vi "COD主界面（列队使用）.vi"() -> (8 "多列列表框":i32(listbox))   [LabVIEW 2016, in "斯坦道CODMn.lvlib"]
uses:
  <vilib>/Analysis/6fits.llb/Curve Fitting Criteria.ctl
  <vilib>/Utility/miscctls.llb/LVPointTypeDef.ctl
  <vilib>/Utility/config.llb/Read Key (I32).vi
  <vilib>/Utility/config.llb/Read Key (Double).vi
  <vilib>/Utility/config.llb/Read Key (Boolean).vi
  <vilib>/Utility/config.llb/Write Key (Double).vi
  <vilib>/Utility/config.llb/Write Key (Boolean).vi
  <vilib>/Utility/config.llb/Write Key (I32).vi
  <vilib>/Waveform/WDTFileIO.llb/Read Waveform from File.vi
  <vilib>/ptbypt/NI_PtbyPt.lvlib
  <vilib>/Utility/config.llb/NI_LVConfig.lvlib
  <vilib>/Analysis/NI_AALPro.lvlib
panel:
  in  "MB通信方式选择":enum16{"串口", "TCP"}(ring)
  in  "采水泵排液时间/s:":i32
  in  "采水泵润洗时间/s:":i32
  in  "采水泵沉淀时间/s:":i32
  in  "采水泵进样时间/s:":i32
  in  "常规版/认证版":enum16{"常规版", "认证版", "浮台版"}(ring)
  in  "释放串口":bool
  in  "打开串口":bool
  in  "保存参数":dbl[](array[numeric])
  out "报警数字":i16
  out "CODMn工作状态":T1(ring)
  out "ORP-K":string
  out "ORP-B":string
  out "ORP-A":string
  out "x = y?":bool
  out "稀释倍数解释":string
  in  "CODMn跨度量程选择":enum32{"H", "L", "AUTO"}(ring)=enum."AUTO"
  in  "跨度液浓度":dbl
  in  "水样":dbl
  in  "蒸馏水":dbl
  in  "标液":dbl
  in  "质控样":dbl
  in  "加标回收":dbl
  in  "草酸钠":dbl
  in  "高锰酸钾":dbl
  in  "硫酸":dbl
  out "量程解释说明":string
  in  "高切低阈值:":dbl
  in  "低切高阈值:":dbl
  in  "自动切换量程:":enum16{"关闭", "自动切换测一次", "自动切换测两次"}(ring)
  in  "修正系数":dbl
  in  "标准液浓度":dbl
  in  "温度":dbl
  in  "恒温时间":dbl
  in  "基本量程":enum16{"L", "H"}(ring)
  in  "CODMn零点核查选择":enum16{"零点核查走纯水管", "零点核查走质控管"}(ring)
  in  "锁定按钮":bool
  in  "低量程稀释倍数:":i8=1
  out "切换量程连续测两次":bool
  in  "高量程稀释倍数:":i8=2
  in  "一键写入":bool
  in  "测量模式(公式)":u16(ring)=1 items=["水样测试"=1, "标样核查"=2, "零点核查"=3, "跨度核查"=4, "空白测试"=5, "平行样"=6, "加标回收"=7]
  out "基本量程(显示)":string
  out "测量模式(显示)":string
  in  "量程切换次数":u8
  out "数据时间":string
  out "断电排液标记":bool
  out "COM":string
  in  "启用5":bool
  in  "校准5":bool
  in  "泵滴定数5":dbl
  in  "浓度5":dbl
  in  "启用4":bool
  in  "校准4":bool
  in  "泵滴定数4":dbl
  in  "浓度4":dbl
  out "波形时间":timestamp
  in  "历史波形":bool
  out "滴定数-ORP值":u16[](array[numeric]) caption="数组"
  in  "关闭 3":bool
  in  "滴定曲线":bool
  out "ORP滴定曲线":u16[](graph)
  out "空白测试标记":bool
  out "跨度核查标记":bool
  out "启动选择 2":u16(ring) items=["水样测试", "标样核查", "零点核查", "跨度核查", "空白测试", "加标回收", "平行样", "校零", "校标"]
  in  "量程选择":enum16{"低量程", "高量程", "0-2量程"}(ring)
  in  "手动控制":bool
  in  "选用水样":enum16{"葡萄糖", "草酸钠"}(ring)
  in  "方程系数":cluster{"K":dbl, "b":dbl, "X^2":dbl} {"X^2" format="%#.6g"; "b" format="%#.6g"; "K" format="%#.6g"}
  out "多项式系数":dbl[](array[numeric])
  out "XY图":cluster{"X Values":dbl[], "Y Values":dbl[]}[](graph)
  in  "模型":enum32{"线性", "多项式"}(ring)
  out "启动时间":timestamp format="%<%Y/%m/%d %H:%M:%S>T"
  in  "关闭 2":bool
  out "r^2":dbl format="%.8g"
  out "拟合公式":string
  out "b":dbl format="%#.4g"
  out "K":dbl format="%#.4f"
  out "当前校准":i32
  in  "启用3":bool
  in  "启用2":bool
  in  "启用1":bool
  in  "校准3":bool
  in  "校准2":bool
  in  "校准1":bool
  in  "泵滴定数3":dbl
  in  "泵滴定数2":dbl
  in  "泵滴定数1":dbl
  in  "浓度3":dbl
  in  "浓度2":dbl
  in  "浓度1":dbl
  in  "写入":bool
  out "测量模式数字":i32
  out "零点核查标记":bool
  out "排液故障":bool
  out "进水样超量程":bool
  out "标样核查标记":bool
  out "平行样测量":bool
  out "加标回收测量":bool
  out "质控样测量":bool
  out "待机":bool
  out "校标错误":bool
  out "校零错误":bool
  out "测量错误":bool
  out "草酸钠报警":bool
  out "高锰酸钾报警":bool
  out "加热故障":bool
  out "温控器故障":bool
  out "ORP故障":bool
  out "排液标记":bool
  out "故障标记":bool
  out "校标标记":bool
  out "校零标记":bool
  out "通讯状态":bool
  out "水样测量":bool
  in  "读取":bool
  in  "返回":bool
  in  "校准配置":bool
  in  "零点泵计量数 2":dbl
  in  "标度泵计量数 2":dbl
  out "标度滴定值":dbl
  out "零点滴定值":dbl
  in  "保存":bool
  in  "关闭":bool
  out "测量数据区":T2 {"单位" items=["ug/L", "mg/L", "ppm", "mg/m3", "cm", "ppb", "ug/m3", "%", "nmol/mol", "umol/mol", "MPN/L", "MPN/100ml", "ng/m3", "NTU", "无量纲", "ms/cm", "us/cm", "℃", "mV", "万个/L"]}
  out "仪器时间":timestamp format="%<%Y/%m/%d %H:%M:%S>T"
  out "秒":u16
  out "分":u16
  out "COD浓度（mg/L)":dbl format="%.2g"
  out "进样管":dbl
  out "高锰酸钾":dbl
  out "草酸钠":dbl
  out "硫酸":dbl
  out "ORP显示":dbl
  out "温度":dbl
  out "加热":bool
  out "搅拌":bool
  out "进硫酸":bool
  out "进加标回收样":bool
  out "进质控样":bool
  out "进标液":bool
  out "进蒸馏水":bool
  out "进水样":bool
  out "进草酸钠":bool
  out "进高锰酸钾":bool
  out "定时启动":bool
  in  "启动":bool
  in  "故障清除":bool
  in  "参数配置":bool
  in  "停止":bool
  in  "单步启动":bool
  out "系统时间":timestamp
  in  "时间校准":bool
  out "报警簇":T3
  out "模式（受控）":u16
  # "测量时间："
  # "(水样~加标回收)"
  # "mV"
  # "℃"
  # "注：遇到加热故障和排液故障时仪器不能正常启动，\n必须排查故障并点击报警清除按钮方可运行。"
  # "mg/L"
  # "基本参数设置"
  # "校零校标结果"
  # "泵计量参数设置"
  # "校零结果："
  # "校零滴定值："
  # "加热恒温温度(℃):"
  # "水样："
  # "高锰酸钾："
  # "校标结果："
  # "标度滴定值："
  # "恒温时间(分钟):"
  # "草酸钠："
  # "蒸馏水："
  # "零点泵计量值："
  # "标准液浓度(mg/L):"
  # "硫酸："
  # "标液："
  # "标度泵计量值："
  # "修正系数："
  # "跨度液浓度："
  # "质控样:"
  # "基本量程(L、H)可选:"
  # "跨度量程选择："
  # "加标回收样："
  # "是否启用"
  # "泵滴定数"
  # "浓度"
  # "辅\n助\n计\n算\n区"
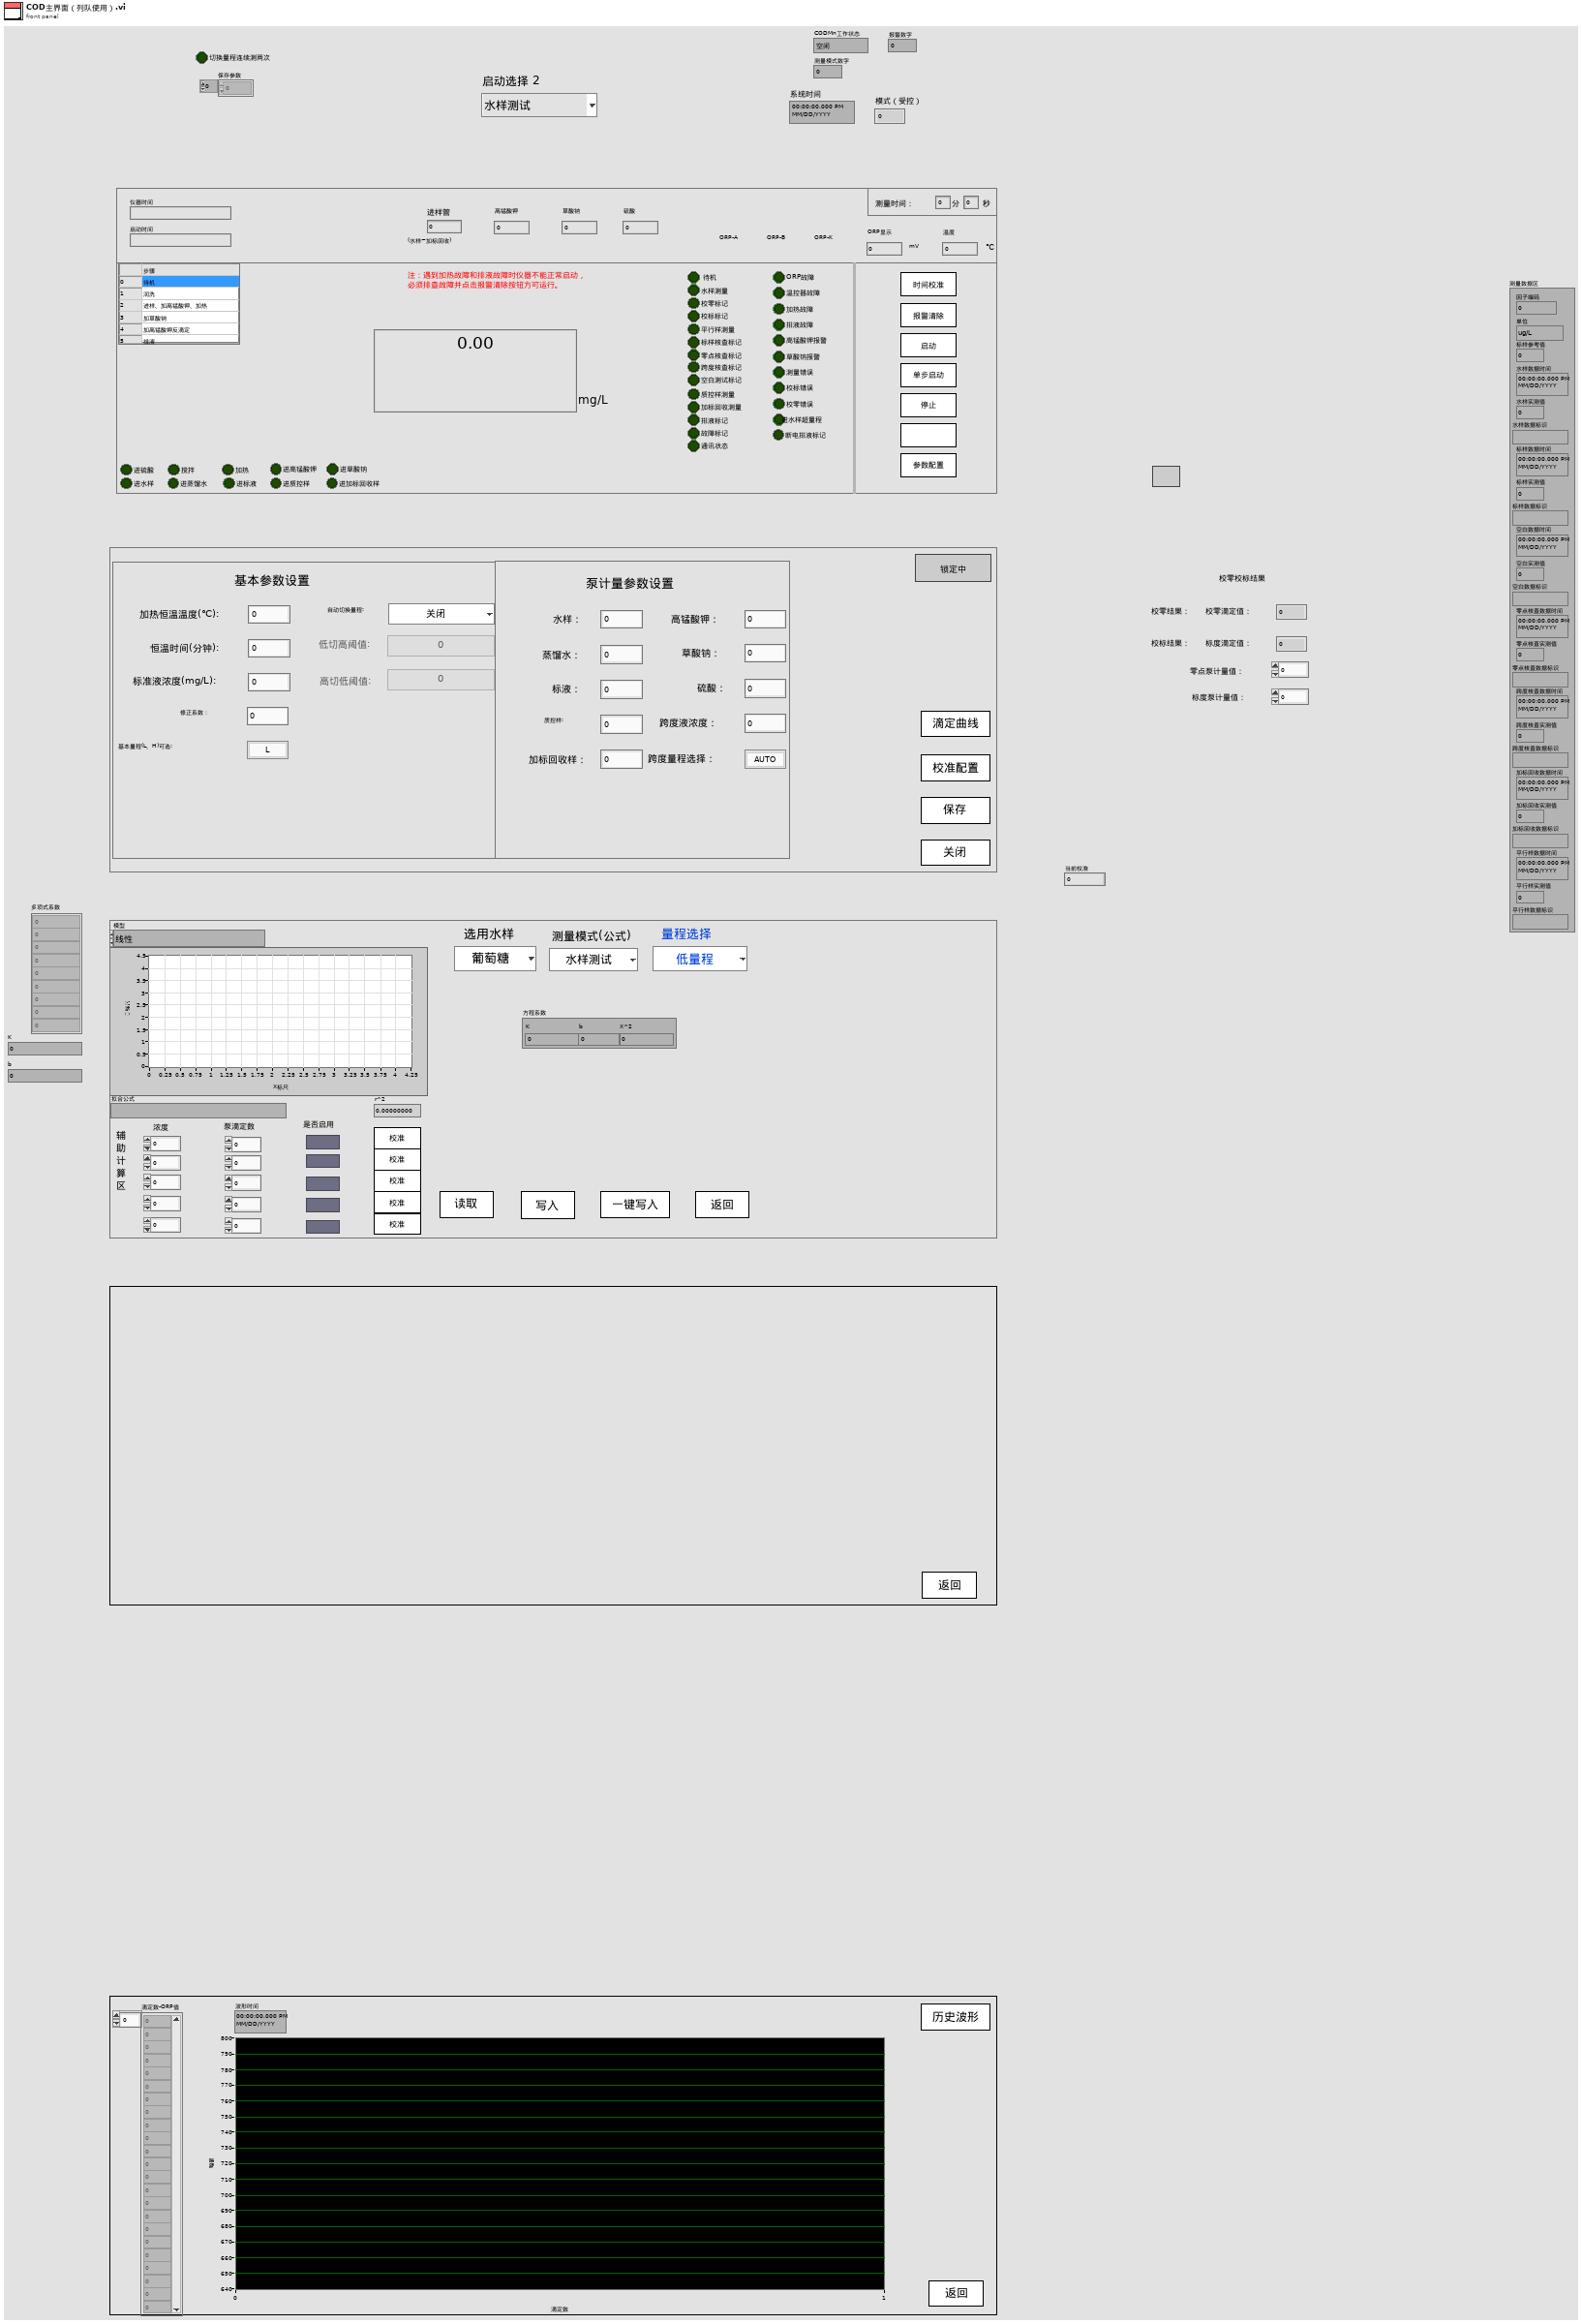
[diagram p1: front panel]
types:
  T1 = enum16{"空闲", "水样测试", "标样核查", "零点核查", "跨度核查", "空白测试", "平行样测试", "质控样", "空白校准", "标样校准", "加标回收"}
  T2 = cluster{"因子编码":u32, "单位":u16, "标样参考值":sgl, "水样数据时间":timestamp, "水样实测值":sgl, "水样数据标识":string, "标样数据时间":timestamp, "标样实测值":sgl, "标样数据标识":string, "空白数据时间":timestamp, "空白实测值":sgl, "空白数据标识":string, "零点核查数据时间":timestamp, "零点核查实测值":sgl, "零点核查数据标识":string, "跨度核查数据时间":timestamp, "跨度核查实测值":sgl, "跨度核查数据标识":string, "加标回收数据时间":timestamp, "加标回收实测值":sgl, "加标回收数据标识":string, "平行样数据时间":timestamp, "平行样实测值":sgl, "平行样数据标识":string}
  T3 = cluster{"ORP故障":bool, "温控器故障":bool, "加热故障":bool, "高锰酸钾报警":bool, "草酸钠报警":bool, "测量错误":bool, "校零错误":bool, "校标错误":bool, " 进水样超量程":bool, "排液阀故障":bool}
  T4 = cluster{"时间":timestamp, "测量模式":string, "数据类型":string, "检测值":sgl, "单位":string, "数据标识":string, "因子编码":string, "标样参考值":sgl, "ORP-A":sgl, "ORP-B":sgl, "ORP-K":sgl, "COD滴定值":sgl, "高锰酸钾滴定数":sgl, "温度":sgl, "量程":sgl}
  T5 = enum8{"Enabled", "Disabled", "Disabled and Grayed Out"}
  T6 = cluster{"数组 2[0]":sgl, "数组 2[1]":sgl, "数组 2[2]":sgl, "数组 2[3]":sgl, "数组 2[4]":sgl, "数组 2[5]":sgl, "数组 2[6]":sgl, "数组 2[7]":sgl, "数组 2[8]":sgl, "数组 2[9]":sgl, "数组 2[10]":sgl, "数组 2[11]":sgl, "数组 2[12]":sgl, "数组 2[13]":sgl, "数组 2[14]":sgl, "数组 2[15]":sgl, "数组 2[16]":sgl, "数组 2[17]":sgl, "数组 2[18]":sgl, "数组 2[19]":sgl, "数组 2[20]":sgl, "数组 2[21]":sgl, "数组 2[22]":sgl, "数组 2[23]":sgl, "数组 2[24]":sgl, "数组 2[25]":sgl, "数组 2[26]":sgl, "数组 2[27]":sgl, "数组 2[28]":sgl, "数组 2[29]":sgl, "数组 2[30]":sgl, "数组 2[31]":sgl, "数组 2[32]":sgl, "数组 2[33]":sgl, "数组 2[34]":sgl, "数组 2[35]":sgl, "数组 2[36]":sgl, "数组 2[37]":sgl, "数组 2[38]":sgl, "数组 2[39]":sgl, "数组 2[40]":sgl, "数组 2[41]":sgl}
  T7 = typedef "NI_AALPro.lvlib/Curve Fitting Criteria.ctl" = u16
  T8 = cluster{"测量模式":enum16{"水样测量", "标样核查", "零点核查", "跨度核查", "空白测试", "加标回收", "平行样", "校零", "校标"}}
  T9 = cluster{"仪器测试类型":enum16{"水样测试", "零点核查", "标样核查", "空白测试", "跨度核查", "加标回收", "平行样", "校零", "校标"}, "周期设置类型":enum16{"定点启动", "间隔启动"}, "定时功能启用":bool, "定时间隔":dbl, "24H周期设置":bool[]}
  T10 = typedef "LVDateTimeRec.ctl" = cluster{"秒数的小数部分":dbl, "秒":i32, "分":i32, "时":i32, "日":i32, "月":i32, "年":i32, "天数（周）":i32, "天数（年）":i32, "DST":i32}
  T11 = enum16{"水样测试", "零点核查", "标样核查", "空白测试", "跨度核查", "加标回收", "平行样", "校零", "校标"}
  T12 = cluster{"时间标识":timestamp, "设备":string, "日志信息":string}
  T13 = cluster{"时间标识":timestamp, "参数":string, "日志信息":string, "流程参数":string}
  T14 = cluster{"时间标识":timestamp, "设备":string, "日志信息":string, "流程参数":string}
  T15 = typedef "NI_LVConfig.lvlib/Config Data RefNum.ctl" = refnum<k1>
  T16 = typedef "LVPointTypeDef.ctl" = cluster{"Horizontal":i16, "Vertical":i16}
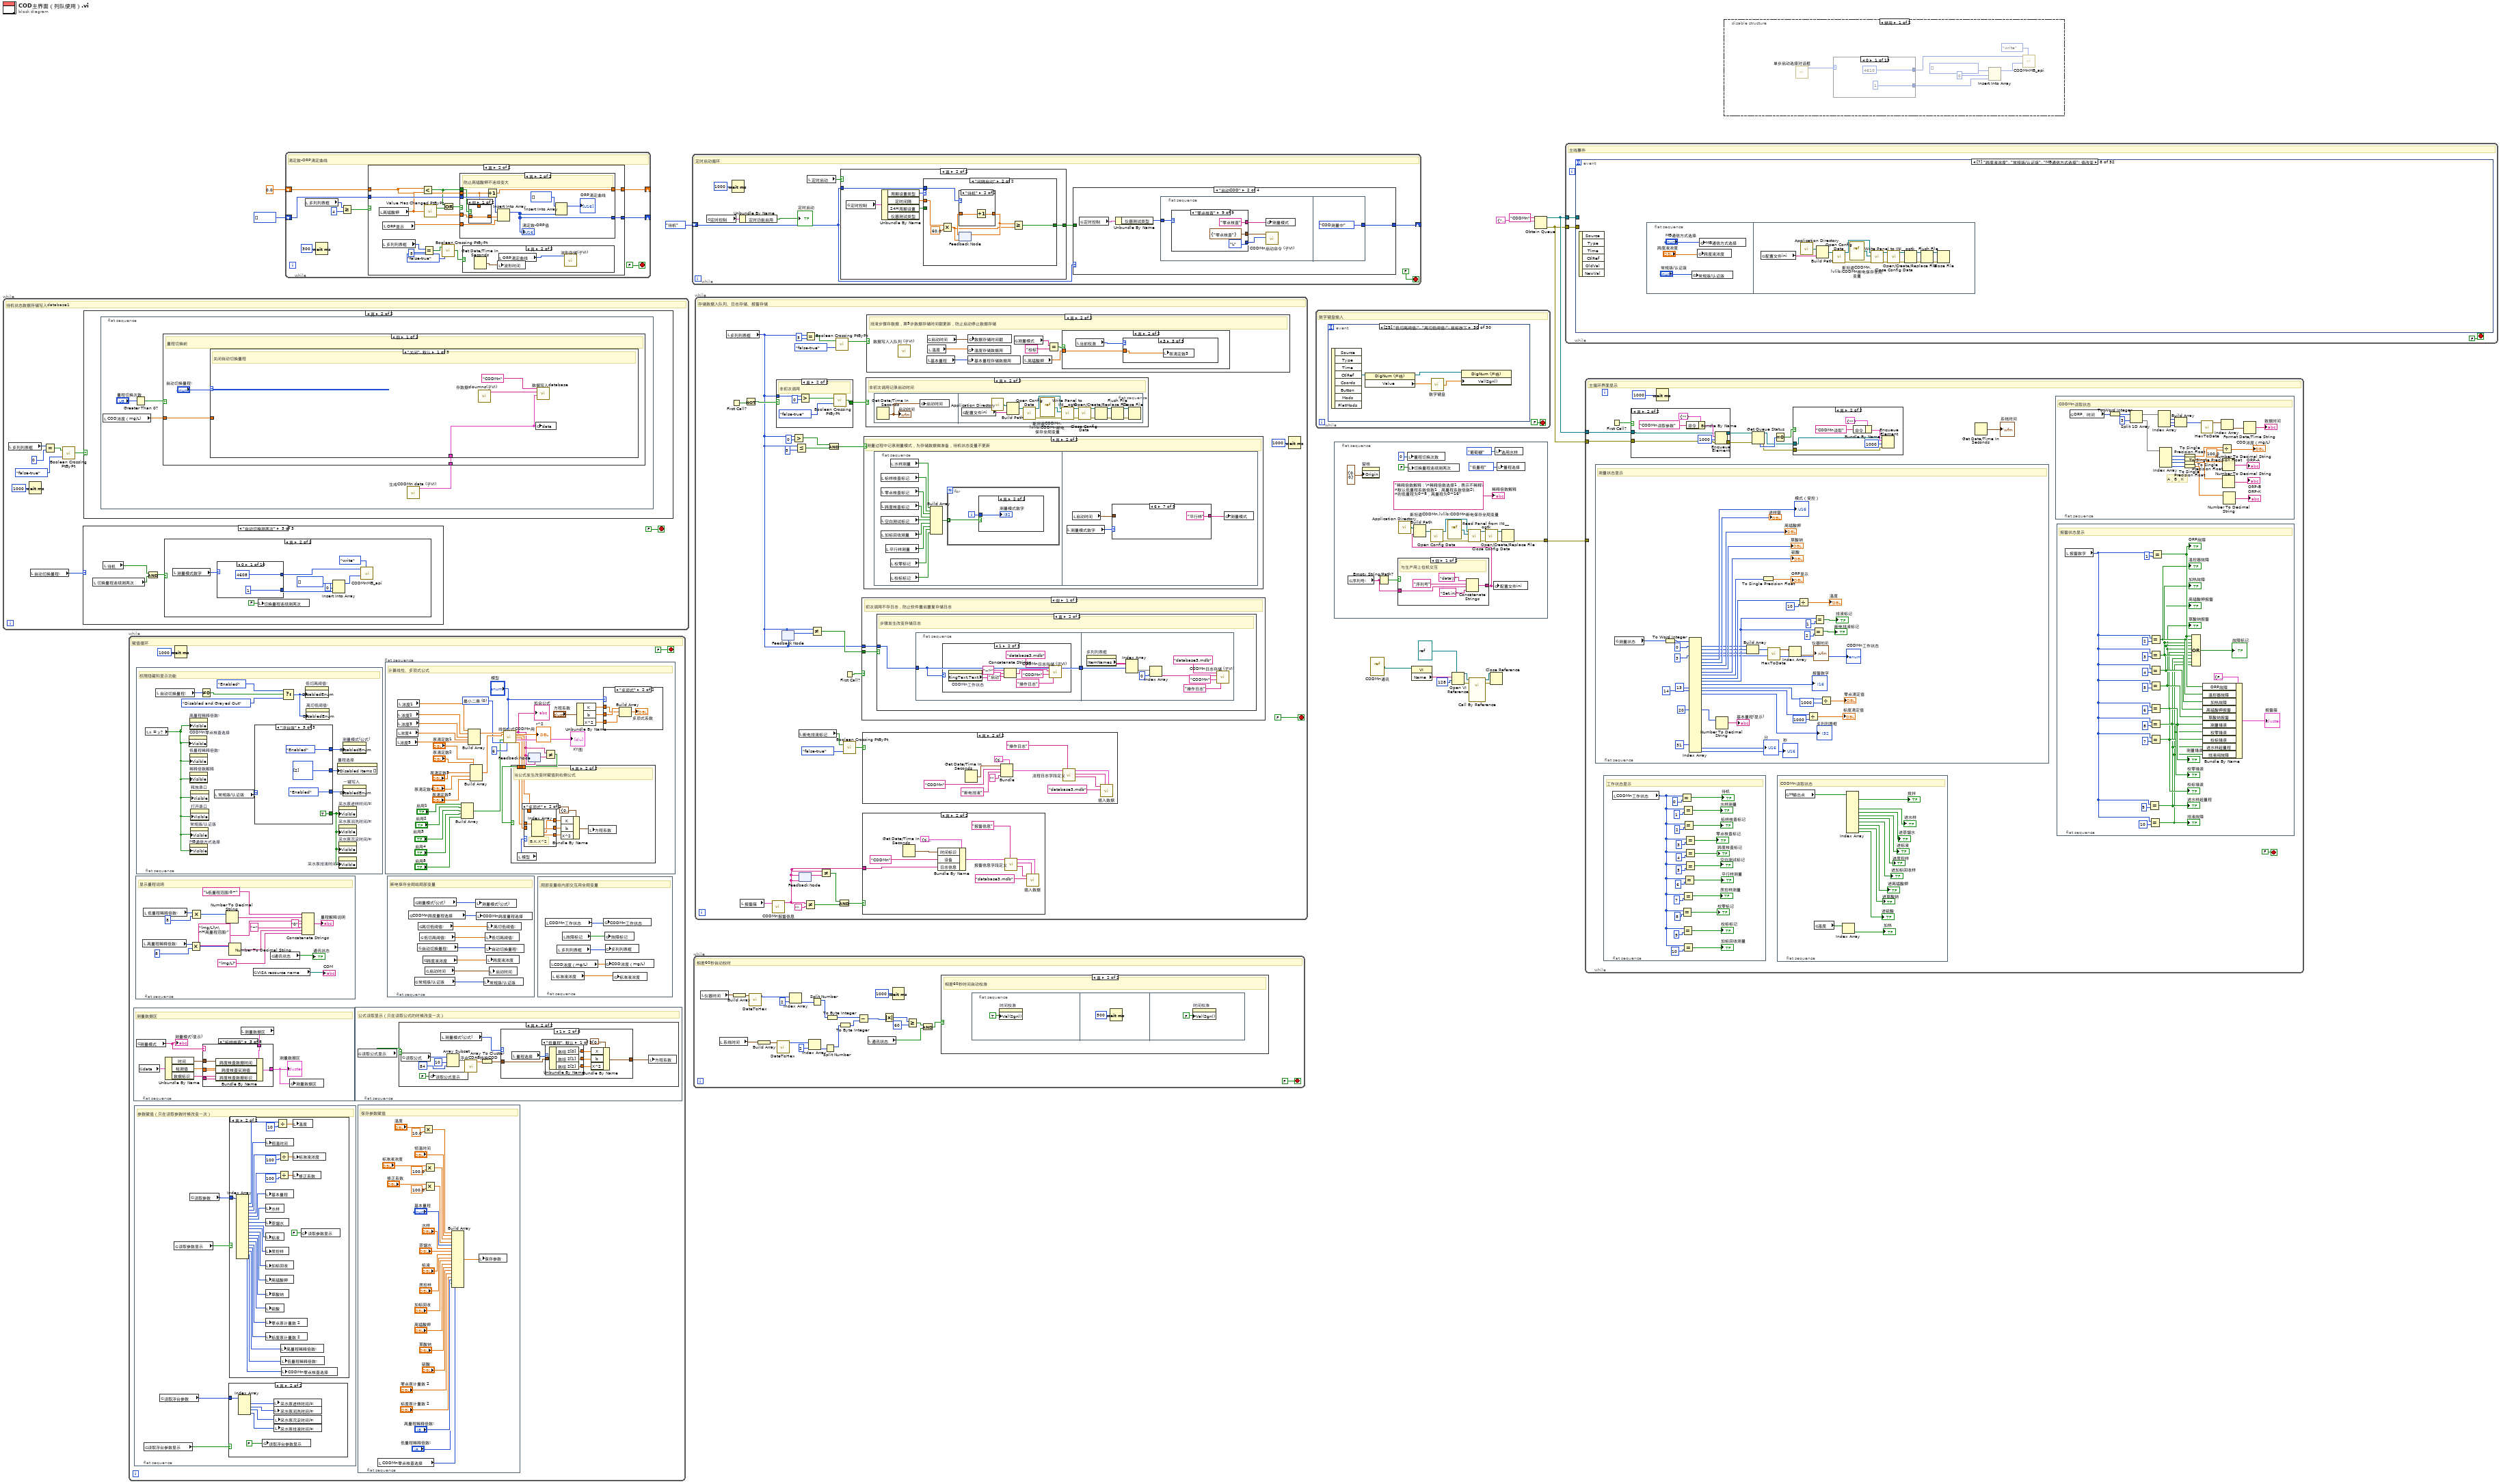
[diagram p0: block diagram]
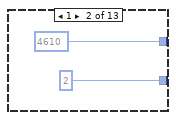
[diagram p2: hidden frame]
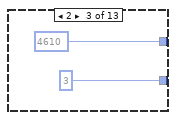
[diagram p3: hidden frame]
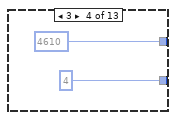
[diagram p4: hidden frame]
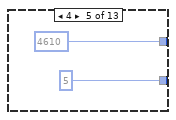
[diagram p5: hidden frame]
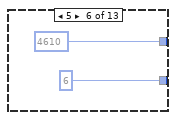
[diagram p6: hidden frame]
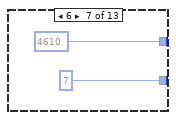
[diagram p7: hidden frame]
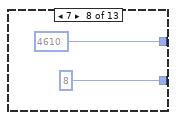
[diagram p8: hidden frame]
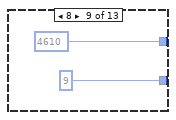
[diagram p9: hidden frame]
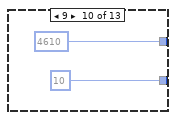
[diagram p10: hidden frame]
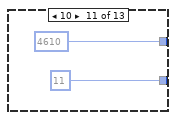
[diagram p11: hidden frame]
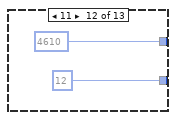
[diagram p12: hidden frame]
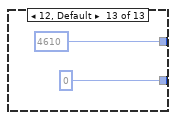
[diagram p13: hidden frame]
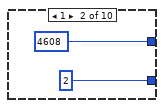
[diagram p19: hidden frame]
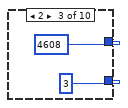
[diagram p20: hidden frame]
diagram:
  n1 = while {
    stop <- FALSE stop-if-true
    # "待机状态数据存储写入database1"
    n2 = local read "多列列表框"() -> (w22:i32)
    n3 = Wait (ms)(milliseconds to wait=u32 1000 ("等待时间（毫秒）")) -> ()  [unwired: 1 out]
    n4 = local read "自动切换量程:"() -> (w17:enum16{"关闭", "自动切换测一次", "自动切换测两次"})
    n5 = Equal?(x=w22, y=0) -> (x = y?=w20:bool)
    n6 = call <vilib>:"Boolean Crossing PtByPt.vi"("direction"=enum16{"either", "false-true", "true-false"}."false-true", "input"=w20) -> ("crossing"=w18:bool)  [unwired: 1 in]
    n7 = case shown="\"自动切换测两次\"" w17 {
      frame "关闭", Default {
      }
      frame "自动切换测一次" {
      }
      frame "自动切换测两次" {
        n8 = local read "切换量程连续测两次"() -> (w26:bool)
        n9 = local read "待机"() -> (w27:bool)
        n10 = Compound Arithmetic op=AND ("复合运算")(w27, w26) -> (w25:bool)
        n11 = case shown="真" w25 {
          frame False {
          }
          frame True {
            n12 = local read "测量模式数字"() -> (w32:i32)
            n13 = case shown="0" w32 {
              tunnel: [u16 4608 ("address") u16 4608 ("address") u16 4608 ("address") u16 4608 ("address") u16 4608 ("address") u16 4608 ("address") u16 4608 ("address") u16 4608 ("address") u16 4608 ("address") u16 4608 ("address")] -> w28
              tunnel: [u16 1 ("address") u16 2 ("address") u16 3 ("address") u16 4 ("address") u16 5 ("address") u16 7 ("address") u16 6 ("address") u16 8 ("address") u16 9 ("address") u16 0 ("address")] -> w35
              frame 0 {
              }
              frame 1 {
              }
              frame 2 {
              }
              frame 3 {
              }
              frame 4 {
              }
              frame 5 {
              }
              frame 6 {
              }
              frame 7 {
              }
              frame 8 {
              }
              frame 9, Default {
              }
            }
            n14 = local write "切换量程连续测两次"(FALSE ("切换量程连续测两次")) -> ()
            n15 = Insert Into Array(array=u16[] [] ("values"), index=0 ("索引"), new element=w35) -> (w29:u16[])
            n16 = call "CODMnMB_api.vi"("STEP"=enum16{"open", "read", "write", "close"}."write", "values"=w29, "starting address"=w28) -> ()  [unwired: 5 in, 4 out]
          }
        }
      }
    }
    n17 = case shown="真" w18 {
      frame False {
      }
      frame True {
        n18 = flat-sequence {
          frame #0 {
            n19 = local read "COD浓度（mg/L)"() -> (w56:dbl)
            n20 = Greater Than 0?(x="量程切换次数") -> (x > 0?=w57:bool)
            n21 = call "生成CODMn data (子VI).vi"() -> ("data"=w59:T4)  [unwired: 11 in]
            n22 = case shown="假" w57 {
              tunnel: w59 -> [w61 w116]
              tunnel: w56 -> [w60 _]
              frame False {
                # "量程切换前"
                n23 = case shown="\"关闭\", 默认" "自动切换量程:" {
                  tunnel: w61 -> [w63 w68 w92]
                  tunnel: w60 -> [_ w67 w91]
                  frame "关闭", Default {
                    # "关闭自动切换量程"
                    n24 = call "存数据cloumns(子VI).vi"() -> ("数组"=w65:string[])  [unwired: 11 in]
                    n25 = global write "COD读取DATA全局.vi" "data"(w63) -> ()
                    n26 = call "数据写入database.vi"("data"=w63, "columns"=w65, "table"="CODMn") -> ()  [unwired: 8 in, 1 out]
                  }
                  frame "自动切换测一次" {
                    # "自动切换量程选择是否重测"
                    n27 = global read "COD测量模式全局.vi" "测量模式"() -> (w74:string)
                    n28 = Not Equal?(x=w74, y="水样测试") -> (x != y?=w72:bool)
                    n29 = case shown="假" w72 {
                      tunnel: [w75 w76] -> w71
                      tunnel: w67 -> [w75 _]
                      frame False {
                      }
                      frame True {
                        n30 = global read "COD读取DATA全局.vi" "测量数据区"() -> (w77:T2)
                        n31 = Unbundle By Name(w77) -> ("水样实测值"=w76:sgl)
                      }
                    }
                    n32 = local read "基本量程"() -> (w66:enum16{"L", "H"})
                    n33 = case shown="\"H\"" w66 {
                      tunnel: w71 -> [w78 w84]
                      frame "L", Default {
                        n34 = Greater?(x=w78, y="低切高阈值:") -> (0:w79:bool)
                        n35 = case shown="假" w79 {
                          frame False {
                          }
                          frame True {
                            n36 = call "CODMnMB_api.vi"("STEP"=enum16{"open", "read", "write", "close"}."write", "values"=u16[] [1], "starting address"=u16 4276) -> ()  [unwired: 5 in, 4 out]
                          }
                        }
                      }
                      frame "H" {
                        n37 = Less?(x=w84, y="高切低阈值:") -> (x < y?=w85:bool)
                        n38 = case shown="真" w85 {
                          frame False {
                          }
                          frame True {
                            n39 = call "CODMnMB_api.vi"("STEP"=enum16{"open", "read", "write", "close"}."write", "values"=u16[] [0], "starting address"=u16 4276) -> ()  [unwired: 5 in, 4 out]
                          }
                        }
                      }
                    }
                    n40 = call "存数据cloumns(子VI).vi"() -> ("数组"=w70:string[])  [unwired: 11 in]
                    n41 = global write "COD读取DATA全局.vi" "data"(w68) -> ()
                    n42 = call "数据写入database.vi"("data"=w68, "columns"=w70, "table"="CODMn") -> ()  [unwired: 8 in, 1 out]
                  }
                  frame "自动切换测两次" {
                    # "自动切换量程选择是否重测"
                    n43 = local read "基本量程"() -> (w90:enum16{"L", "H"})
                    n44 = case shown="\"H\"" w90 {
                      tunnel: w91 -> [w94 w105]
                      tunnel: w92 -> [w93 w104]
                      frame "L", Default {
                        n45 = local read "低切高阈值:"() -> (w95:dbl)
                        n46 = Greater?(x=w94, y=w95) -> (0:w96:bool)
                        n47 = case shown="假" w96 {
                          tunnel: w93 -> [w97 _]
                          frame False {
                            n48 = call "存数据cloumns(子VI).vi"() -> ("数组"=w99:string[])  [unwired: 11 in]
                            n49 = global write "COD读取DATA全局.vi" "data"(w97) -> ()
                            n50 = call "数据写入database.vi"("data"=w97, "columns"=w99, "table"="CODMn") -> ()  [unwired: 8 in, 1 out]
                          }
                          frame True {
                            n51 = call "CODMnMB_api.vi"("STEP"=enum16{"open", "read", "write", "close"}."write", "values"=u16[] [1], "starting address"=u16 4276) -> ()  [unwired: 5 in, 4 out]
                            "切换量程连续测两次" <- TRUE ("切换量程连续测两次")
                          }
                        }
                      }
                      frame "H" {
                        n52 = local read "高切低阈值:"() -> (w106:dbl)
                        n53 = Less?(x=w105, y=w106) -> (x < y?=w107:bool)
                        n54 = case shown="真" w107 {
                          tunnel: w104 -> [w108 _]
                          frame False {
                            n55 = call "存数据cloumns(子VI).vi"() -> ("数组"=w110:string[])  [unwired: 11 in]
                            n56 = global write "COD读取DATA全局.vi" "data"(w108) -> ()
                            n57 = call "数据写入database.vi"("data"=w108, "columns"=w110, "table"="CODMn") -> ()  [unwired: 8 in, 1 out]
                          }
                          frame True {
                            # "重测第一次不存数据"
                            n58 = call "CODMnMB_api.vi"("STEP"=enum16{"open", "read", "write", "close"}."write", "values"=u16[] [0], "starting address"=u16 4276) -> ()  [unwired: 5 in, 4 out]
                            n59 = local write "切换量程连续测两次"(TRUE ("切换量程连续测两次")) -> ()
                          }
                        }
                      }
                    }
                  }
                }
              }
              frame True {
                # "防止无限切量程"
                n60 = local write "量程切换次数"(u8 0 ("量程切换次数")) -> ()
                n61 = call "存数据cloumns(子VI).vi"() -> ("数组"=w118:string[])  [unwired: 11 in]
                n62 = call "数据写入database.vi"("data"=w116, "columns"=w118, "table"="CODMn") -> ()  [unwired: 8 in, 1 out]
                n63 = global write "COD读取DATA全局.vi" "data"(w116) -> ()
              }
            }
          }
        }
      }
    }
  }
  n64 = while {
    stop <- FALSE stop-if-true
    # "赋值循环"
    n65 = flat-sequence {
      frame #0 {
        # "测量数据区"
        n66 = global read "COD测量模式全局.vi" "测量模式"() -> (w386:string)
        "测量模式(显示)" <- w386
        n67 = global read "COD读取DATA全局.vi" "data"() -> (w391:T4)
        n68 = Unbundle By Name(w391) -> ("时间"=w390:timestamp, "检测值"=w389:sgl, "数据标识"=w388:string)
        n69 = local read "测量数据区"() -> (w392:T2)
        n70 = case shown="\"标样核查\"" w386 {
          tunnel: w392 -> [w393 w398 w403 w408 w413 w418 w423 w428]
          tunnel: [w393 w397 w399 w407 w412 w417 w419 w427] -> w387
          tunnel: w390 -> [_ w396 w402 w406 w411 w416 w422 w426]
          tunnel: w389 -> [_ w395 w401 w405 w410 w415 w421 w425]
          tunnel: w388 -> [_ w394 w400 w404 w409 w414 w420 w424]
          frame "", Default {
          }
          frame "水样测试" {
            n71 = Bundle By Name(cluster=w398, "水样数据时间"=w396, "水样实测值"=w395, "水样数据标识"=w394) -> (w397:T2)
          }
          frame "标样核查" {
            n72 = Bundle By Name(cluster=w403, "跨度核查数据时间"=w402, "跨度核查实测值"=w401, "跨度核查数据标识"=w400) -> (w399:T2)
          }
          frame "零点核查" {
            n73 = Bundle By Name(cluster=w408, "零点核查数据时间"=w406, "零点核查实测值"=w405, "零点核查数据标识"=w404) -> (w407:T2)
          }
          frame "加标回收" {
            n74 = Bundle By Name(cluster=w413, "加标回收数据时间"=w411, "加标回收实测值"=w410, "加标回收数据标识"=w409) -> (w412:T2)
          }
          frame "平行样" {
            n75 = Bundle By Name(cluster=w418, "平行样数据时间"=w416, "平行样实测值"=w415, "平行样数据标识"=w414) -> (w417:T2)
          }
          frame "校零" {
            n76 = Bundle By Name(cluster=w423, "空白数据时间"=w422, "空白实测值"=w421, "空白数据标识"=w420) -> (w419:T2)
          }
          frame "校标" {
            n77 = Bundle By Name(cluster=w428, "标样数据时间"=w426, "标样实测值"=w425, "标样数据标识"=w424) -> (w427:T2)
          }
        }
        "测量数据区" <- w387
        n78 = global write "COD读取DATA全局.vi" "测量数据区"(w387) -> ()
      }
    }
    n79 = flat-sequence {
      frame #0 {
        # "参数赋值（只在读取参数时候改变一次）"
        n80 = global read "COD读取DATA全局.vi" "读取浮台参数显示"() -> (w152:bool)
        n81 = global read "COD读取DATA全局.vi" "读取浮台参数"() -> (w151:u16[])
        n82 = global read "COD读取DATA全局.vi" "读取参数显示"() -> (w153:bool)
        n83 = global read "COD读取DATA全局.vi" "读取参数"() -> (w154:u16[])
        n84 = case shown="真" w152 {
          tunnel: w151 -> [_ w160]
          frame False {
          }
          frame True {
            n85 = Index Array(array=w160) -> (element #1=w159:u16, element #2=w158:u16, element #3=w157:u16, element #4=w156:u16)  [unwired: 4 in]
            n86 = global write "COD读取DATA全局.vi" "读取浮台参数显示"(FALSE ("读取参数显示")) -> ()
            n87 = local write "采水泵进样时间/s:"(w159) -> ()
            n88 = local write "采水泵润洗时间/s:"(w158) -> ()
            n89 = local write "采水泵沉淀时间/s:"(w157) -> ()
            n90 = local write "采水泵排液时间/s:"(w156) -> ()
          }
        }
        n91 = case shown="真" w153 {
          tunnel: w154 -> [_ w162]
          frame False {
          }
          frame True {
            n92 = Index Array(array=w162) -> (element #1=w174:u16, element #2=w186:u16, element #3=w167:u16, element #4=w172:u16, element #5=w170:u16, element #6=w169:u16, element #7=w185:u16, element #8=w184:u16, element #9=w183:u16, element #10=w182:u16, element #11=w181:u16, element #12=w180:u16, element #13=w179:u16, element #14=w178:u16, element #15=w177:u16, element #16=w165:u16, element #17=w164:u16, element #18=w163:u16)  [unwired: 18 in]
            n93 = local write "恒温时间"(w186) -> ()
            n94 = local write "基本量程"(w170) -> ()
            n95 = local write "水样"(w169) -> ()
            n96 = local write "蒸馏水"(w185) -> ()
            n97 = local write "标液"(w184) -> ()
            n98 = local write "质控样"(w183) -> ()
            n99 = local write "加标回收"(w182) -> ()
            n100 = local write "高锰酸钾"(w181) -> ()
            n101 = local write "草酸钠"(w180) -> ()
            n102 = local write "硫酸"(w179) -> ()
            n103 = local write "零点泵计量数 2"(w178) -> ()
            n104 = local write "标度泵计量数 2"(w177) -> ()
            n105 = Divide(x=w174, y=u16 10) -> (x/y=w175:dbl)
            n106 = Divide(x=w167, y=u16 100) -> (x/y=w166:dbl)
            n107 = Divide(x=w172, y=u16 100) -> (x/y=w171:dbl)
            n108 = local write "高量程稀释倍数:"(w165) -> ()
            n109 = local write "低量程稀释倍数:"(w164) -> ()
            n110 = local write "CODMn零点核查选择"(w163) -> ()
            n111 = local write "温度"(w175) -> ()
            n112 = local write "标准液浓度"(w166) -> ()
            n113 = local write "修正系数"(w171) -> ()
            n114 = global write "COD读取DATA全局.vi" "读取参数显示"(FALSE ("读取参数显示")) -> ()
          }
        }
      }
    }
    n115 = flat-sequence {
      frame #0 {
        # "显示量程说明"
        n116 = local read "高量程稀释倍数:"() -> (w440:i8)
        n117 = local read "低量程稀释倍数:"() -> (w450:i8)
        n118 = Multiply(x=w440, y=i8 8) -> (x*y=w438:i8)
        n119 = Multiply(x=w450, y=i8 8) -> (x*y=w442:i8)
        n120 = Number To Decimal String(number=w442) -> (decimal integer string=w447:string)  [unwired: 1 in]
        n121 = Number To Decimal String(number=w438) -> (decimal integer string=w445:string)  [unwired: 1 in]
        n122 = global read "CODMn断电保存全局变量.vi" "VISA resource name"() -> (→"COM":refnum<visa-resource-name>)
        n123 = global read "COD读取DATA全局.vi" "通讯状态"() -> (→"通讯状态":bool)
        n124 = Concatenate Strings("L低量程范围:0~" ("量程解释说明"), w447, "(mg/L)\n\nH高量程范围:" ("量程解释说明"), "0" ("字符串"), "~" ("量程解释说明"), w445, "(mg/L)" ("量程解释说明")) -> (→"量程解释说明":string)
      }
    }
    n125 = flat-sequence {
      frame #0 {
        # "权限隐藏和显示功能"
        n126 = local read "x = y?"() -> (w453:bool)
        n127 = local read "自动切换量程:"() -> (w460:enum16{"关闭", "自动切换测一次", "自动切换测两次"})
        n128 = property on="CODMn零点核查选择" class="Enum (严格)"("Visible"=w453) -> ()  [unwired: 2 in, 2 out]
        n129 = property on="高量程稀释倍数:" class="DigNum (严格)"("Visible"=w453) -> ()  [unwired: 2 in, 2 out]
        n130 = property on="低量程稀释倍数:" class="DigNum (严格)"("Visible"=w453) -> ()  [unwired: 2 in, 2 out]
        n131 = property on="稀释倍数解释" class="Str"("Visible"=w453) -> ()  [unwired: 2 in, 2 out]
        n132 = property on="MB通信方式选择" class="Enum (严格)"("Visible"=w453) -> ()  [unwired: 2 in, 2 out]
        n133 = property on="常规版/认证版" class="Enum (严格)"("Visible"=w453) -> ()  [unwired: 2 in, 2 out]
        n134 = property on="释放串口" class="Bool"("Visible"=w453) -> ()  [unwired: 2 in, 2 out]
        n135 = property on="打开串口" class="Bool"("Visible"=w453) -> ()  [unwired: 2 in, 2 out]
        n136 = Not Equal To 0?(x=w460) -> (x != 0?=w459:bool)
        n137 = local read "常规版/认证版"() -> (w458:enum16{"常规版", "认证版", "浮台版"})
        n138 = case shown="\"浮台版\"" w458 {
          tunnel: [T5."Enabled" ("禁用") T5."Disabled and Grayed Out" ("禁用") T5."Enabled" ("禁用")] -> w457
          tunnel: [i32[] [2] ("禁用项[]") i32[] [] ("禁用项[]") i32[] [2] ("禁用项[]")] -> w456
          tunnel: [T5."Enabled" ("禁用") T5."Disabled and Grayed Out" ("禁用") T5."Enabled" ("禁用")] -> w455
          tunnel: [FALSE FALSE TRUE] -> w454
          frame "常规版", Default {
          }
          frame "认证版" {
            w469 = u16 1 items=["水样测试"=1, "标样核查"=2, "零点核查"=3, "跨度核查"=4, "空白测试"=5, "平行样"=6, "加标回收"=7] ("测量模式(公式)")
            n139 = global write "CODMn断电保存全局变量.vi" "测量模式(公式)"(w469) -> ()
          }
          frame "浮台版" {
          }
        }
        n140 = Select(t=T5."Enabled" ("禁用"), s=w459, f=T5."Disabled and Grayed Out" ("禁用")) -> (s? t:f=w461:T5)
        n141 = property on="低切高阈值:" class="DigNum (严格)"("DisabledEnum"=w461) -> ()  [unwired: 2 in, 2 out]
        n142 = property on="高切低阈值:" class="DigNum (严格)"("DisabledEnum"=w461) -> ()  [unwired: 2 in, 2 out]
        n143 = property on="量程选择" class="Enum (严格)"("Disabled Items []"=w456) -> ()  [unwired: 2 in, 2 out]
        n144 = property on="采水泵进样时间/s:" class="DigNum (严格)"("Visible"=w454) -> ()  [unwired: 2 in, 2 out]
        n145 = property on="采水泵润洗时间/s:" class="DigNum (严格)"("Visible"=w454) -> ()  [unwired: 2 in, 2 out]
        n146 = property on="采水泵沉淀时间/s:" class="DigNum (严格)"("Visible"=w454) -> ()  [unwired: 2 in, 2 out]
        n147 = property on="采水泵排液时间/s:" class="DigNum (严格)"("Visible"=w454) -> ()  [unwired: 2 in, 2 out]
        n148 = property on="测量模式(公式)" class="Ring (严格)"("DisabledEnum"=w457) -> ()  [unwired: 2 in, 2 out]
        n149 = property on="一键写入" class="Bool (严格)"("DisabledEnum"=w455) -> ()  [unwired: 2 in, 2 out]
      }
    }
    n150 = Wait (ms)(milliseconds to wait=u32 1000 ("等待时间（毫秒）")) -> ()  [unwired: 1 out]
    n151 = flat-sequence {
      frame #0 {
        # "公式读取显示（只在读取公式的时候改变一次）"
        n152 = global read "COD读取DATA全局.vi" "读取公式显示"() -> (w187:bool)
        n153 = case shown="真" w187 {
          frame False {
          }
          frame True {
            n154 = global read "COD读取DATA全局.vi" "读取公式"() -> (w196:u16[])
            n155 = global write "COD读取DATA全局.vi" "读取公式显示"(FALSE ("读取参数显示")) -> ()
            n156 = local read "测量模式(公式)"() -> (w194:u16)
            n157 = Array Subset(array=w196, index=10 ("索引"), length=84 ("长度")) -> (w191:u16[])
            n158 = call "浮点CDAB转换COD.vi"("数组"=w191) -> ("数组 2"=w192:sgl[])  [unwired: 10 in]
            n159 = Array To Cluster(array=w192) -> (cluster=w195:T6)
            n160 = case shown="1" w194 {
              tunnel: [cluster{"X":dbl, "b":dbl, "X^2":dbl} {"X"=999.0, "b"=999.0, "X^2"=999.0} ("方程系数") w199 w218 w237 w256 w275 w294 w313] -> w193
              tunnel: w195 -> [_ w198 w217 w236 w255 w274 w293 w312]
              frame 0, Default {
              }
              frame 1 {
                n161 = local read "量程选择"() -> (w201:enum16{"低量程", "高量程", "0-2量程"})
                n162 = case shown="\"低量程\", 默认" w201 {
                  tunnel: w198 -> [w208 w212 w216]
                  tunnel: [w207 w211 w215] -> w204
                  tunnel: [w206 w210 w214] -> w203
                  tunnel: [w205 w209 w213] -> w202
                  frame "低量程", Default {
                    n163 = Unbundle By Name(w208) -> ("数组 2[0]"=w207:sgl, "数组 2[1]"=w206:sgl, "数组 2[2]"=w205:sgl)
                  }
                  frame "高量程" {
                    n164 = Unbundle By Name(w212) -> ("数组 2[3]"=w211:sgl, "数组 2[4]"=w210:sgl, "数组 2[5]"=w209:sgl)
                  }
                  frame "0-2量程" {
                    n165 = Unbundle By Name(w216) -> ("数组 2[6]"=w215:sgl, "数组 2[7]"=w214:sgl, "数组 2[8]"=w213:sgl)
                  }
                }
                n166 = Bundle By Name(cluster=cluster{"X":dbl, "b":dbl, "X^2":dbl} {"X"=0.0, "b"=0.0, "X^2"=0.0} ("方程系数"), "X"=w204, "b"=w203, "X^2"=w202) -> (w199:cluster{"X":dbl, "b":dbl, "X^2":dbl})
              }
              frame 2 {
                n167 = local read "量程选择"() -> (w220:enum16{"低量程", "高量程", "0-2量程"})
                n168 = case shown="\"高量程\"" w220 {
                  tunnel: w217 -> [w227 w231 w235]
                  tunnel: [w226 w230 w234] -> w223
                  tunnel: [w225 w229 w233] -> w222
                  tunnel: [w224 w228 w232] -> w221
                  frame "低量程", Default {
                    n169 = Unbundle By Name(w227) -> ("数组 2[6]"=w226:sgl, "数组 2[7]"=w225:sgl, "数组 2[8]"=w224:sgl)
                  }
                  frame "高量程" {
                    n170 = Unbundle By Name(w231) -> ("数组 2[9]"=w230:sgl, "数组 2[10]"=w229:sgl, "数组 2[11]"=w228:sgl)
                  }
                  frame "0-2量程" {
                    n171 = Unbundle By Name(w235) -> ("数组 2[6]"=w234:sgl, "数组 2[7]"=w233:sgl, "数组 2[8]"=w232:sgl)
                  }
                }
                n172 = Bundle By Name(cluster=cluster{"X":dbl, "b":dbl, "X^2":dbl} {"X"=0.0, "b"=0.0, "X^2"=0.0} ("方程系数"), "X"=w223, "b"=w222, "X^2"=w221) -> (w218:cluster{"X":dbl, "b":dbl, "X^2":dbl})
              }
              frame 3 {
                n173 = local read "量程选择"() -> (w239:enum16{"低量程", "高量程", "0-2量程"})
                n174 = case shown="\"高量程\"" w239 {
                  tunnel: w236 -> [w246 w250 w254]
                  tunnel: [w245 w249 w253] -> w242
                  tunnel: [w244 w248 w252] -> w241
                  tunnel: [w243 w247 w251] -> w240
                  frame "低量程", Default {
                    n175 = Unbundle By Name(w246) -> ("数组 2[12]"=w245:sgl, "数组 2[13]"=w244:sgl, "数组 2[14]"=w243:sgl)
                  }
                  frame "高量程" {
                    n176 = Unbundle By Name(w250) -> ("数组 2[15]"=w249:sgl, "数组 2[16]"=w248:sgl, "数组 2[17]"=w247:sgl)
                  }
                  frame "0-2量程" {
                    n177 = Unbundle By Name(w254) -> ("数组 2[6]"=w253:sgl, "数组 2[7]"=w252:sgl, "数组 2[8]"=w251:sgl)
                  }
                }
                n178 = Bundle By Name(cluster=cluster{"X":dbl, "b":dbl, "X^2":dbl} {"X"=0.0, "b"=0.0, "X^2"=0.0} ("方程系数"), "X"=w242, "b"=w241, "X^2"=w240) -> (w237:cluster{"X":dbl, "b":dbl, "X^2":dbl})
              }
              frame 4 {
                n179 = local read "量程选择"() -> (w258:enum16{"低量程", "高量程", "0-2量程"})
                n180 = case shown="\"高量程\"" w258 {
                  tunnel: w255 -> [w265 w269 w273]
                  tunnel: [w264 w268 w272] -> w261
                  tunnel: [w263 w267 w271] -> w260
                  tunnel: [w262 w266 w270] -> w259
                  frame "低量程", Default {
                    n181 = Unbundle By Name(w265) -> ("数组 2[18]"=w264:sgl, "数组 2[19]"=w263:sgl, "数组 2[20]"=w262:sgl)
                  }
                  frame "高量程" {
                    n182 = Unbundle By Name(w269) -> ("数组 2[21]"=w268:sgl, "数组 2[22]"=w267:sgl, "数组 2[23]"=w266:sgl)
                  }
                  frame "0-2量程" {
                    n183 = Unbundle By Name(w273) -> ("数组 2[6]"=w272:sgl, "数组 2[7]"=w271:sgl, "数组 2[8]"=w270:sgl)
                  }
                }
                n184 = Bundle By Name(cluster=cluster{"X":dbl, "b":dbl, "X^2":dbl} {"X"=0.0, "b"=0.0, "X^2"=0.0} ("方程系数"), "X"=w261, "b"=w260, "X^2"=w259) -> (w256:cluster{"X":dbl, "b":dbl, "X^2":dbl})
              }
              frame 5 {
                n185 = local read "量程选择"() -> (w277:enum16{"低量程", "高量程", "0-2量程"})
                n186 = case shown="\"高量程\"" w277 {
                  tunnel: w274 -> [w284 w288 w292]
                  tunnel: [w283 w287 w291] -> w280
                  tunnel: [w282 w286 w290] -> w279
                  tunnel: [w281 w285 w289] -> w278
                  frame "低量程", Default {
                    n187 = Unbundle By Name(w284) -> ("数组 2[24]"=w283:sgl, "数组 2[25]"=w282:sgl, "数组 2[26]"=w281:sgl)
                  }
                  frame "高量程" {
                    n188 = Unbundle By Name(w288) -> ("数组 2[27]"=w287:sgl, "数组 2[28]"=w286:sgl, "数组 2[29]"=w285:sgl)
                  }
                  frame "0-2量程" {
                    n189 = Unbundle By Name(w292) -> ("数组 2[6]"=w291:sgl, "数组 2[7]"=w290:sgl, "数组 2[8]"=w289:sgl)
                  }
                }
                n190 = Bundle By Name(cluster=cluster{"X":dbl, "b":dbl, "X^2":dbl} {"X"=0.0, "b"=0.0, "X^2"=0.0} ("方程系数"), "X"=w280, "b"=w279, "X^2"=w278) -> (w275:cluster{"X":dbl, "b":dbl, "X^2":dbl})
              }
              frame 6 {
                n191 = local read "量程选择"() -> (w296:enum16{"低量程", "高量程", "0-2量程"})
                n192 = case shown="\"高量程\"" w296 {
                  tunnel: w293 -> [w303 w307 w311]
                  tunnel: [w302 w306 w310] -> w299
                  tunnel: [w301 w305 w309] -> w298
                  tunnel: [w300 w304 w308] -> w297
                  frame "低量程", Default {
                    n193 = Unbundle By Name(w303) -> ("数组 2[30]"=w302:sgl, "数组 2[31]"=w301:sgl, "数组 2[32]"=w300:sgl)
                  }
                  frame "高量程" {
                    n194 = Unbundle By Name(w307) -> ("数组 2[33]"=w306:sgl, "数组 2[34]"=w305:sgl, "数组 2[35]"=w304:sgl)
                  }
                  frame "0-2量程" {
                    n195 = Unbundle By Name(w311) -> ("数组 2[6]"=w310:sgl, "数组 2[7]"=w309:sgl, "数组 2[8]"=w308:sgl)
                  }
                }
                n196 = Bundle By Name(cluster=cluster{"X":dbl, "b":dbl, "X^2":dbl} {"X"=0.0, "b"=0.0, "X^2"=0.0} ("方程系数"), "X"=w299, "b"=w298, "X^2"=w297) -> (w294:cluster{"X":dbl, "b":dbl, "X^2":dbl})
              }
              frame 7 {
                n197 = local read "量程选择"() -> (w315:enum16{"低量程", "高量程", "0-2量程"})
                n198 = case shown="\"高量程\"" w315 {
                  tunnel: w312 -> [w322 w326 w330]
                  tunnel: [w321 w325 w329] -> w318
                  tunnel: [w320 w324 w328] -> w317
                  tunnel: [w319 w323 w327] -> w316
                  frame "低量程", Default {
                    n199 = Unbundle By Name(w322) -> ("数组 2[36]"=w321:sgl, "数组 2[37]"=w320:sgl, "数组 2[38]"=w319:sgl)
                  }
                  frame "高量程" {
                    n200 = Unbundle By Name(w326) -> ("数组 2[39]"=w325:sgl, "数组 2[40]"=w324:sgl, "数组 2[41]"=w323:sgl)
                  }
                  frame "0-2量程" {
                    n201 = Unbundle By Name(w330) -> ("数组 2[6]"=w329:sgl, "数组 2[7]"=w328:sgl, "数组 2[8]"=w327:sgl)
                  }
                }
                n202 = Bundle By Name(cluster=cluster{"X":dbl, "b":dbl, "X^2":dbl} {"X"=0.0, "b"=0.0, "X^2"=0.0} ("方程系数"), "X"=w318, "b"=w317, "X^2"=w316) -> (w313:cluster{"X":dbl, "b":dbl, "X^2":dbl})
              }
            }
            n203 = local write "方程系数"(w193) -> ()
          }
        }
      }
    }
    n204 = flat-sequence {
      frame #0 {
        # "保存参数赋值"
        n205 = local read "CODMn零点核查选择"() -> (w122:enum16{"零点核查走纯水管", "零点核查走质控管"})
        n206 = Multiply(x="温度", y=10.0) -> (x*y=w131:dbl)
        n207 = Multiply(x="标准液浓度", y=100.0) -> (x*y=w125:dbl)
        n208 = Multiply(x="修正系数", y=100.0) -> (x*y=w128:dbl)
        n209 = Build Array(w131, "恒温时间", w125, w128, "基本量程", "水样", "蒸馏水", "标液", "质控样", "加标回收", "高锰酸钾", "草酸钠", "硫酸", "零点泵计量数 2", "标度泵计量数 2", "高量程稀释倍数:", "低量程稀释倍数:", w122) -> (w121:dbl[])
        n210 = local write "保存参数"(w121) -> ()
      }
    }
    n211 = flat-sequence {
      frame #0 {
        w358 = T7 0 items=["最小二乘", "最小绝对残差", "Bisquare"] ("method")
        # "计算线性、多项式公式"
        n212 = local read "浓度5"() -> (w352:dbl)
        n213 = local read "浓度4"() -> (w353:dbl)
        n214 = local read "浓度2"() -> (w362:dbl)
        n215 = local read "浓度3"() -> (w363:dbl)
        n216 = local read "浓度1"() -> (w361:dbl)
        n217 = Build Array("启用1", "启用2", "启用3", "启用4", "启用5") -> (w346:bool[])
        n218 = Build Array(w361, w362, w363, w353, w352) -> (w360:dbl[])
        n219 = Build Array("泵滴定数1", "泵滴定数2", "泵滴定数3", "泵滴定数4", "泵滴定数5") -> (w359:dbl[])
        n220 = call "线性公式CODMn用.vi"("标液浓度"=w360, "监测浓度"=w359, "启用"=w346, "method"=w358, "模型"="模型", "精度"=6) -> ("拟合方程"=w339:string, "r^2"=→"r^2":dbl, "slope"=w337:dbl, "intercept"=w338:dbl, "XY图"=→"XY图":cluster{"X Values":dbl[], "Y Values":dbl[]}[], "Polynomial Coefficients"=w354:dbl[])  [unwired: 8 in]
        "拟合公式" <- w339
        n221 = feedback-in #1(w339) -> ()
        n222 = feedback #1(w339) -> (w340:string)
        n223 = Not Equal?(x=w339, y=w340) -> (x != y?=w336:bool)
        n224 = case shown="真" w336 {
          tunnel: w354 -> [_ w371]
          tunnel: w338 -> [_ w373]
          tunnel: w337 -> [_ w374]
          frame False {
          }
          frame True {
            # "当公式发生改变时赋值到右侧公式"
            n225 = local read "模型"() -> (w376:enum32{"线性", "多项式"})
            n226 = case shown="\"多项式\"" w376 {
              tunnel: [w381 w383] -> w375
              tunnel: w374 -> [w381 _]
              tunnel: w373 -> [w380 _]
              tunnel: [w380 w384] -> w372
              tunnel: w371 -> [_ w385]
              tunnel: [0.0 ("数值") w382] -> w370
              frame "线性", Default {
              }
              frame "多项式" {
                # "B,K,X^2"
                n227 = Index Array(array=w385) -> (element #1=w384:dbl, element #2=w383:dbl, element #3=w382:dbl)  [unwired: 3 in]
              }
            }
            n228 = Bundle By Name(cluster=cluster{"K":dbl, "b":dbl, "X^2":dbl} {"K"=0.0, "b"=0.0, "X^2"=0.0} ("方程系数"), "K"=w375, "b"=w372, "X^2"=w370) -> (w377:cluster{"K":dbl, "b":dbl, "X^2":dbl})
            n229 = local write "方程系数"(w377) -> ()
          }
        }
        n230 = Unbundle By Name("方程系数") -> ("K"=w333:dbl, "b"=w332:dbl, "X^2"=w331:dbl)
        n231 = case shown="\"多项式\"" "模型" {
          tunnel: w333 -> [w365 w368]
          tunnel: w332 -> [w364 w369]
          tunnel: w331 -> [_ w367]
          frame "线性", Default {
            "K" <- w365
            "b" <- w364
          }
          frame "多项式" {
            n232 = Build Array(w369, w368, w367) -> (→"多项式系数":dbl[])
          }
        }
      }
    }
    n233 = flat-sequence {
      frame #0 {
        # "断电保存全局给局部变量"
        n234 = global read "CODMn断电保存全局变量.vi" "CODMn跨度量程选择"() -> (w435:enum32{"H", "L", "AUTO"})
        n235 = global read "CODMn断电保存全局变量.vi" "测量模式(公式)"() -> (w436:u16)
        n236 = global read "CODMn断电保存全局变量.vi" "常规版/认证版"() -> (w429:enum16{"常规版", "认证版", "浮台版"})
        n237 = global read "CODMn断电保存全局变量.vi" "自动切换量程:"() -> (w432:enum16{"关闭", "自动切换测一次", "自动切换测两次"})
        n238 = global read "CODMn断电保存全局变量.vi" "高切低阈值:"() -> (w434:dbl)
        n239 = global read "CODMn断电保存全局变量.vi" "低切高阈值:"() -> (w433:dbl)
        n240 = global read "CODMn断电保存全局变量.vi" "跨度液浓度"() -> (w431:dbl)
        n241 = global read "CODMn断电保存全局变量.vi" "启动时间"() -> (w430:timestamp)
        n242 = local write "测量模式(公式)"(w436) -> ()
        n243 = local write "CODMn跨度量程选择"(w435) -> ()
        n244 = local write "常规版/认证版"(w429) -> ()
        n245 = local write "自动切换量程:"(w432) -> ()
        n246 = local write "低切高阈值:"(w433) -> ()
        n247 = local write "跨度液浓度"(w431) -> ()
        n248 = local write "高切低阈值:"(w434) -> ()
        n249 = local write "启动时间"(w430) -> ()
      }
    }
    n250 = flat-sequence {
      frame #0 {
        # "局部变量给内部交互用全局变量"
        n251 = local read "CODMn工作状态"() -> (w150:T1)
        n252 = local read "COD浓度（mg/L)"() -> (w147:dbl)
        n253 = local read "标准液浓度"() -> (w146:dbl)
        n254 = local read "多列列表框"() -> (w148:i32)
        n255 = local read "故障标记"() -> (w149:bool)
        n256 = global write "COD测量模式全局.vi" "CODMn工作状态"(w150) -> ()
        n257 = global write "COD读取DATA全局.vi" "故障标记"(w149) -> ()
        n258 = global write "运行时序全局变量.vi" "多列列表框"(w148) -> ()
        n259 = global write "COD浓度全局变量.vi" "COD浓度（mg/L)"(w147) -> ()
        n260 = global write "COD浓度全局变量.vi" "标准液浓度"(w146) -> ()
      }
    }
  }
  n261 = while {
    shift-right: [w482] -> _
    shift-left: u16[] [] ("ORP滴定曲线") -> [w483]
    shift-right: [w477] -> _
    shift-left: 0.0 -> [w478]
    stop <- FALSE stop-if-true
    # "滴定数-ORP滴定曲线"
    n262 = local read "多列列表框"() -> (w481:i32)
    n263 = Wait (ms)(milliseconds to wait=u32 300 ("等待时间（毫秒）")) -> ()  [unwired: 1 out]
    n264 = Greater Or Equal?(x=w481, y=4) -> (x >= y?=w479:bool)
    n265 = case shown="真" w479 {
      tunnel: w483 -> [_ w502]
      tunnel: [u16[] [] ("ORP滴定曲线") w501] -> w482
      tunnel: w478 -> [_ w490]
      tunnel: [0.0 w489] -> w477
      frame False {
      }
      frame True {
        n266 = local read "高锰酸钾"() -> (w492:dbl)
        n267 = local read "多列列表框"() -> (w497:i32)
        n268 = local read "ORP显示"() -> (w498:dbl)
        n269 = Less?(x=w490, y=w492) -> (x < y?=w488:bool)
        n270 = Equal?(x=w497, y=5) -> (x = y?=w495:bool)
        n271 = call <vilib>:"Value Has Changed PtByPt.vi"("input data point"=w492) -> ("has changed"=w500:bool, "output data point"=w499:dbl)  [unwired: 1 in]
        n272 = call <vilib>:"Boolean Crossing PtByPt.vi"("direction"=enum16{"either", "false-true", "true-false"}."false-true", "input"=w495) -> ("crossing"=w493:bool)  [unwired: 1 in]
        n273 = Or(x=w488, y=w500) -> (x .or. y?=w491:bool)
        n274 = case shown="真" w491 {
          tunnel: w502 -> [w509 w523]
          tunnel: [w508 w522] -> w501
          tunnel: w499 -> [w510 w516]
          tunnel: w498 -> [w506 w521]
          tunnel: w490 -> [w505 w518]
          tunnel: [w505 w520] -> w489
          tunnel: w488 -> [_ w519]
          frame False {
            n275 = Equal To 0?(x=w510) -> (x = 0?=w507:bool)
            n276 = case shown="真" w507 {
              tunnel: [w511 w514] -> w508
              tunnel: w509 -> [w511 _]
              tunnel: w506 -> [_ w513]
              frame False {
              }
              frame True {
                n277 = Insert Into Array(array=u16[] [] ("ORP滴定曲线"), index=0 ("索引"), new element=w513) -> (w514:u16[])
                n278 = local write "滴定数-ORP值"(w514) -> ()
              }
            }
          }
          frame True {
            # "防止高锰酸钾不连续变大"
            n279 = case shown="假" w519 {
              tunnel: w518 -> [_ w527]
              tunnel: [w526 w527] -> w517
              tunnel: w516 -> [w526 _]
              frame False {
              }
              frame True {
              }
            }
            n280 = Increment(x=w518) -> (x+1=w520:dbl)
            n281 = Insert Into Array(array=w523, index=w517, new element=w521) -> (w522:u16[])
            "滴定数-ORP值" <- w522
            n282 = Insert Into Array(array=u16[] [] ("ORP滴定曲线"), new element=w522) -> (→"ORP滴定曲线":u16[])  [unwired: 1 in]
          }
        }
        n283 = case shown="真" w493 {
          frame False {
          }
          frame True {
            n284 = Get Date/Time In Seconds() -> (seconds since 1Jan1904=w503:timestamp)
            n285 = local write "波形时间"(w503) -> ()
            n286 = local read "ORP滴定曲线"() -> (w504:u16[])
            n287 = call "波形存储(子VI).vi"("ORP滴定曲线"=w504) -> ()  [unwired: 11 in]
          }
        }
      }
    }
  }
  n288 = while {
    shift-right: [w533] -> _
    shift-left: enum16{"待机", "启动COD", "COD测量中", "延时"}."待机" -> [w532]
    stop <- FALSE stop-if-true
    # "定时启动循环"
    n289 = global read "CODMn断电保存全局变量.vi" "定时控制"() -> (w529:T9)
    n290 = Wait (ms)(milliseconds to wait=u32 1000 ("等待时间（毫秒）")) -> ()  [unwired: 1 out]
    n291 = Unbundle By Name(w529) -> ("定时功能启用"=→"定时启动":bool)
    n292 = local read "定时启动"() -> (w530:bool)
    n293 = case shown="真" w530 {
      tunnel: w532 -> [_ w588]
      tunnel: [_ w587] -> w531
      frame False {
      }
      frame True {
        n294 = global read "CODMn断电保存全局变量.vi" "定时控制"() -> (w586:T9)
        n295 = Unbundle By Name(w586) -> ("周期设置类型"=w589:enum16{"定点启动", "间隔启动"}, "定时间隔"=w590:dbl, "24H周期设置"=w591:bool[])  [unwired: 1 out]
        n296 = case shown="\"间隔启动\"" w589 {
          tunnel: w590 -> [_ w608]
          tunnel: w591 -> [w594 _]
          tunnel: w588 -> [w592 w611]
          tunnel: [w593 w606] -> w587
          frame "定点启动", Default {
            n297 = case shown="\"待机\", 默认" w592 {
              tunnel: w594 -> [w602 _]
              tunnel: [w595 _] -> w593
              frame "待机", Default {
                n298 = Get Date/Time In Seconds() -> (seconds since 1Jan1904=w604:timestamp)
                n299 = Seconds To Date/Time(time stamp (now)=w604) -> (date time rec=w603:T10)  [unwired: 1 in]
                n300 = Unbundle By Name(w603) -> ("时"=w601:i32, "分"=w599:i32, "秒"=w600:i32)
                n301 = Equal To 0?(x=w599) -> (x = 0?=w597:bool)
                n302 = Equal To 0?(x=w600) -> (x = 0?=w596:bool)
                n303 = Index Array(array=w602, index=w601) -> (element=w598:bool)
                n304 = Compound Arithmetic op=AND ("复合运算")(w598, w597, w596) -> (w595:bool)
              }
              frame "启动COD" {
              }
            }
          }
          frame "间隔启动" {
            n305 = Multiply(x=w608, y=60.0) -> (x*y=w605:dbl)
            n306 = feedback #2(w605) -> (w610:dbl)
            n307 = case shown="\"待机\"" w611 {
              tunnel: w610 -> [_ w613]
              tunnel: [_ w612] -> w609
              frame Default {
              }
              frame "待机" {
                n308 = Increment(x=w613) -> (x+1=w612:dbl)
              }
            }
            n309 = feedback-in #2(w609) -> ()
            n310 = Greater Or Equal?(x=w609, y=w605) -> (x >= y?=w606:bool)
          }
        }
      }
    }
    n311 = case shown="\"启动COD\"" w532 {
      tunnel: [w536 w542 w576 enum16{"待机", "启动COD", "COD测量中", "延时"}."待机"] -> w533
      tunnel: w531 -> [w539 _ _ _]
      frame "待机", Default {
        n312 = Select(t=enum16{"待机", "启动COD", "COD测量中", "延时"}."启动COD", s=w539, f=enum16{"待机", "启动COD", "COD测量中", "延时"}."待机") -> (s? t:f=w536:enum16{"待机", "启动COD", "COD测量中", "延时"})
      }
      frame "启动COD" {
        n313 = global read "CODMn断电保存全局变量.vi" "定时控制"() -> (w540:T9)
        n314 = Unbundle By Name(w540) -> ("仪器测试类型"=w541:T11)
        n315 = flat-sequence {
          tunnel: w541 -> [w546]
          tunnel: [enum16{"待机", "启动COD", "COD测量中", "延时"}."COD测量中"] -> w542
          frame #0 {
            n316 = case shown="\"零点核查\"" w546 {
              tunnel: [T8 {"测量模式"=enum."水样测量"} ("启动测量模式") T8 {"测量模式"=enum."标样核查"} ("启动测量模式") T8 {"测量模式"=enum."空白测试"} ("启动测量模式") T8 {"测量模式"=enum."跨度核查"} ("启动测量模式") T8 {"测量模式"=enum."加标回收"} ("启动测量模式") T8 {"测量模式"=enum."平行样"} ("启动测量模式") T8 {"测量模式"=enum."校零"} ("启动测量模式") T8 {"测量模式"=enum."校标"} ("启动测量模式") T8 {"测量模式"=enum."零点核查"} ("启动测量模式")] -> w545
              tunnel: ["水样测试" ("测量模式") "标样核查" ("测量模式") "空白测试" ("测量模式") "跨度核查" ("测量模式") "加标回收" ("测量模式") "平行样" ("测量模式") "校零" ("测量模式") "校标" ("测量模式") "零点核查" ("测量模式")] -> w544
              tunnel: [enum32{"H", "L", "AUTO"}."AUTO" ("CODMn跨度量程选择") w550 enum32{"H", "L", "AUTO"}."L" ("CODMn跨度量程选择") w556 enum32{"H", "L", "AUTO"}."AUTO" ("CODMn跨度量程选择") enum32{"H", "L", "AUTO"}."AUTO" ("CODMn跨度量程选择") enum32{"H", "L", "AUTO"}."L" ("CODMn跨度量程选择") enum32{"H", "L", "AUTO"}."AUTO" ("CODMn跨度量程选择") enum32{"H", "L", "AUTO"}."L" ("CODMn跨度量程选择")] -> w543
              frame "水样测试", Default {
              }
              frame "标样核查" {
                n317 = local read "CODMn跨度量程选择"() -> (w550:enum32{"H", "L", "AUTO"})
              }
              frame "空白测试" {
              }
              frame "跨度核查" {
                n318 = local read "CODMn跨度量程选择"() -> (w556:enum32{"H", "L", "AUTO"})
              }
              frame "加标回收" {
              }
              frame "平行样" {
              }
              frame "校零" {
              }
              frame "校标" {
              }
              frame "零点核查" {
              }
            }
            n319 = global write "COD测量模式全局.vi" "测量模式"(w544) -> ()
            n320 = call "CODMn启动命令 (子VI).vi"("CODMn量程切换"=w543, "启动测量模式"=w545) -> ()  [unwired: 10 in]
          }
          frame #1 {
          }
        }
      }
      frame "COD测量中" {
        n321 = flat-sequence {
          tunnel: [w577] -> w575
          tunnel: [w584] -> w576
          tunnel: w575 -> [w584]
          frame #0 {
            n322 = global read "运行时序全局变量.vi" "多列列表框"() -> (w582:i32)
            n323 = Equal?(x=w582, y=0) -> (x = y?=w580:bool)
            n324 = Select(t=enum16{"待机", "启动COD", "COD测量中", "延时"}."延时", s=w580, f=enum16{"待机", "启动COD", "COD测量中", "延时"}."COD测量中") -> (s? t:f=w577:enum16{"待机", "启动COD", "COD测量中", "延时"})
          }
          frame #1 {
            n325 = Wait (ms)(milliseconds to wait=u32 5000 ("等待时间（毫秒）")) -> ()  [unwired: 1 out]
          }
        }
      }
      frame "延时" {
      }
    }
  }
  n326 = while {
    stop <- FALSE stop-if-true
    # "相差60秒自动校时"
    n327 = local read "仪器时间"() -> (w617:timestamp)
    n328 = local read "系统时间"() -> (w618:timestamp)
    n329 = Build Array(w617) -> (w616:timestamp[])
    n330 = call "DateToHex.vi"("DATE"=w616) -> ("数组"=w629:u16[])  [unwired: 10 in]
    n331 = Build Array(w618) -> (w635:timestamp[])
    n332 = call "DateToHex.vi"("DATE"=w635) -> ("数组"=w634:u16[])  [unwired: 10 in]
    n333 = Index Array(array=w629, index=2 ("索引")) -> (element=w631:u16)
    n334 = Index Array(array=w634, index=2 ("索引")) -> (element=w632:u16)
    n335 = Split Number(x=w631) -> (hi(x)=w625:u8)  [unwired: 1 out]
    n336 = Split Number(x=w632) -> (hi(x)=w628:u8)  [unwired: 1 out]
    n337 = To Byte Integer(number=w625) -> (8bit integer=w624:i8)
    n338 = To Byte Integer(number=w628) -> (8bit integer=w627:i8)
    n339 = Subtract(x=w624, y=w627) -> (x-y=w626:i8)
    n340 = local read "通讯状态"() -> (w620:bool)
    n341 = Absolute Value(x=w626) -> (abs(x)=w623:i8)
    n342 = Wait (ms)(milliseconds to wait=u32 1000 ("等待时间（毫秒）")) -> ()  [unwired: 1 out]
    n343 = Greater Or Equal?(x=w623, y=i8 60) -> (x >= y?=w621:bool)
    n344 = And(x=w621, y=w620) -> (x .and. y?=w619:bool)
    n345 = case shown="真" w619 {
      frame False {
      }
      frame True {
        # "相差60秒时间自动校准"
        n346 = flat-sequence {
          frame #0 {
            n347 = property on="时间校准" class="Bool (严格)"("Val(Sgnl)"=TRUE ("值(信号)")) -> ()  [unwired: 2 in, 2 out]
          }
          frame #1 {
            n348 = Wait (ms)(milliseconds to wait=u32 500 ("等待时间（毫秒）")) -> ()  [unwired: 1 out]
          }
          frame #2 {
            n349 = property on="时间校准" class="Bool (严格)"("Val(Sgnl)"=FALSE ("值(信号)")) -> ()  [unwired: 2 in, 2 out]
          }
        }
      }
    }
  }
  n350 = while {
    stop <- FALSE stop-if-true
    # "存储数据入队列、日志存储、报警存储"
    n351 = local read "多列列表框"() -> (w639:i32)
    n352 = First Call?() -> (First Call?: T/F=w642:bool)
    n353 = local read "报警簇"() -> (w643:T3)
    n354 = Not(x=w642) -> (.not. x?=w640:bool)
    n355 = call "CODMn报警信息.vi"("报警簇"=w643) -> ("CODMN报警信息"=w644:string)  [unwired: 10 in]
    n356 = case shown="真" w640 {
      selector: w640 -> [w667 _]
      tunnel: w639 -> [_ w669]
      tunnel: [w667 w668] -> w641
      frame False {
      }
      frame True {
        # "非初次调用"
        n357 = Greater?(x=w669, y=u16 0) -> (0:w672:bool)
        n358 = call <vilib>:"Boolean Crossing PtByPt.vi"("direction"=enum16{"either", "false-true", "true-false"}."false-true", "input"=w672) -> ("crossing"=w668:bool)  [unwired: 1 in]
      }
    }
    n359 = feedback #3(w639) -> (w655:i32)
    n360 = feedback-in #3(w639) -> ()
    n361 = Greater?(x=w639, y=u16 0) -> (0:w666:bool)
    n362 = Less Or Equal?(x=w639, y=u16 5) -> (x <= y?=w663:bool)
    n363 = local read "断电排液标记"() -> (w651:bool)
    n364 = feedback #4(w644) -> (w645:string)
    n365 = feedback-in #4(w644) -> ()
    n366 = Not Equal?(x=w644, y="") -> (x != y?=w649:bool)
    n367 = Equal?(x=w639, y=u16 5) -> (x = y?=w659:bool)
    n368 = Not Equal?(x=w639, y=w655) -> (x != y?=w656:bool)
    n369 = Not Equal?(x=w644, y=w645) -> (x != y?=w646:bool)
    n370 = And(x=w666, y=w663) -> (x .and. y?=w664:bool)
    n371 = call <vilib>:"Boolean Crossing PtByPt.vi"("direction"=enum16{"either", "false-true", "true-false"}."false-true", "input"=w659) -> ("crossing"=w661:bool)  [unwired: 1 in]
    n372 = And(x=w646, y=w649) -> (x .and. y?=w647:bool)
    n373 = call <vilib>:"Boolean Crossing PtByPt.vi"("direction"=enum16{"either", "false-true", "true-false"}."false-true", "input"=w651) -> ("crossing"=w650:bool)  [unwired: 1 in]
    n374 = First Call?() -> (First Call?: T/F=w657:bool)
    n375 = case shown="假" w657 {
      tunnel: w656 -> [w695 _]
      tunnel: w639 -> [w694 _]
      frame False {
        # "初次调用不存日志，防止软件重启重复存储日志"
        n376 = case shown="真" w695 {
          tunnel: w694 -> [_ w697]
          frame False {
          }
          frame True {
            # "步骤发生改变存储日志"
            n377 = flat-sequence {
              tunnel: w697 -> [w698]
              tunnel: [w698] -> w696
              tunnel: w696 -> [w718]
              frame #0 {
                n378 = case shown="1" w698 {
                  frame 0 {
                    n379 = global read "COD测量模式全局.vi" "测量模式"() -> (w705:string)
                    n380 = Concatenate Strings("-->", w705, "结束" ("字符串")) -> (w704:string)
                    n381 = call "CODMn日志存储 (子VI).vi"("table输入"="操作日志", "参数"="CODMn" ("table输入"), "日志信息"=w704, "database"="database3.mdb") -> ()  [unwired: 8 in]
                  }
                  frame 1 {
                    n382 = property on="CODMn工作状态" class="Enum (严格)"() -> ("RingText.Text"=w708:string)  [unwired: 2 in, 2 out]
                    n383 = Concatenate Strings("-->", w708, "启动" ("字符串")) -> (w706:string)
                    n384 = call "CODMn日志存储 (子VI).vi"("table输入"="操作日志", "参数"="CODMn" ("table输入"), "日志信息"=w706, "database"="database3.mdb") -> ()  [unwired: 8 in]
                  }
                  frame 2, Default {
                  }
                }
              }
              frame #1 {
                n385 = property on="多列列表框" class="MCListbox (严格)"() -> ("ItemNames"=w716:string[][])  [unwired: 2 in, 2 out]
                n386 = Index Array(array=w716, index (row)=w718) -> (element=w715:string[])  [unwired: 1 in]
                n387 = Index Array(array=w715, index=0 ("索引")) -> (element=w713:string)
                n388 = call "CODMn日志存储 (子VI).vi"("table输入"="操作日志", "参数"="CODMn" ("table输入"), "日志信息"=w713, "database"="database3.mdb") -> ()  [unwired: 8 in]
              }
            }
          }
        }
      }
      frame True {
      }
    }
    n389 = case shown="真" w650 {
      frame False {
      }
      frame True {
        n390 = Get Date/Time In Seconds() -> (seconds since 1Jan1904=w688:timestamp)
        n391 = Bundle(cluster=T13 {"时间标识"=timestamp(0 s since 1904-01-01), "参数"="", "日志信息"="", "流程参数"=""} ("data in"), "时间标识"=w688, "参数"="CODMn" ("table输入"), "日志信息"="断电排液", "流程参数"="" ("table输入")) -> (w686:T13)
        n392 = call "流程日志字段定义.vi"("table输入"="操作日志", "data in"=w686) -> ("table输出"=w691:string, "columns"=w692:string[], "data out"=w693:T14)  [unwired: 7 in]
        n393 = call "插入数据.vi"("data"=w693, "columns"=w692, "database"="database3.mdb", "table"=w691) -> ()  [unwired: 7 in, 1 out]
      }
    }
    n394 = case shown="真" w647 {
      tunnel: w644 -> [_ w673]
      frame False {
      }
      frame True {
        n395 = Get Date/Time In Seconds() -> (seconds since 1Jan1904=w675:timestamp)
        n396 = Bundle By Name(cluster=T12 {"时间标识"=timestamp(0 s since 1904-01-01), "设备"="", "日志信息"=""} ("data in"), "时间标识"=w675, "设备"="CODMn", "日志信息"=w673) -> (w676:T12)
        n397 = call "报警信息字段定义.vi"("table输入"="报警信息", "data in"=w676) -> ("table输出"=w680:string, "columns"=w681:string[], "data out"=w682:T12)  [unwired: 7 in]
        n398 = call "插入数据.vi"("data"=w682, "columns"=w681, "database"="database3.mdb", "table"=w680) -> ()  [unwired: 7 in, 1 out]
      }
    }
    n399 = case shown="真" w664 {
      frame False {
      }
      frame True {
        # "测量过程中记录测量模式，为存储数据做准备，待机状态变量不更新"
        n400 = flat-sequence {
          frame #0 {
            n401 = local read "标样核查标记"() -> (w744:bool)
            n402 = local read "零点核查标记"() -> (w743:bool)
            n403 = local read "跨度核查标记"() -> (w741:bool)
            n404 = local read "空白测试标记"() -> (w740:bool)
            n405 = local read "加标回收测量"() -> (w739:bool)
            n406 = local read "平行样测量"() -> (w738:bool)
            n407 = local read "水样测量"() -> (w745:bool)
            n408 = local read "校零标记"() -> (w737:bool)
            n409 = local read "校标标记"() -> (w736:bool)
            n410 = Build Array(w745, w744, w743, w741, w740, w739, w738, w737, w736) -> (w742:bool[])
            n411 = for {
              tunnel: w742 -> [w747] mode=indexing
              i -> [w746]
              n412 = case shown="真" w747 {
                tunnel: w746 -> [_ w748]
                frame False {
                }
                frame True {
                  "测量模式数字" <- w748
                }
              }
            }
          }
          frame #1 {
            n413 = local read "测量模式数字"() -> (w751:i32)
            n414 = local read "启动时间"() -> (w749:timestamp)
            n415 = case shown="6" w751 {
              tunnel: ["水样测试" ("测量模式") "标样核查" ("测量模式") "零点核查" ("测量模式") "跨度核查" ("测量模式") "空白测试" ("测量模式") "加标回收" ("测量模式") "平行样" ("测量模式") "校零" ("测量模式") "校标" ("测量模式")] -> w750
              tunnel: w749 -> [w752 _ _ _ _ w758 _ _ _]
              frame 0, Default {
                n416 = global write "COD测量模式全局.vi" "水样启动时间"(w752) -> ()
              }
              frame 1 {
              }
              frame 2 {
              }
              frame 3 {
              }
              frame 4 {
              }
              frame 5 {
                n417 = global write "COD测量模式全局.vi" "加标回收启动时间"(w758) -> ()
              }
              frame 6 {
              }
              frame 7 {
              }
              frame 8 {
              }
            }
            n418 = global write "COD测量模式全局.vi" "测量模式"(w750) -> ()
          }
        }
      }
    }
    n419 = case shown="真" w641 {
      frame False {
      }
      frame True {
        # "非初次调用记录启动时间"
        n420 = flat-sequence {
          frame #0 {
            n421 = Get Date/Time In Seconds() -> (seconds since 1Jan1904=w721:timestamp)
            "启动时间" <- w721
            n422 = global write "CODMn断电保存全局变量.vi" "启动时间"(w721) -> ()
          }
          frame #1 {
            n423 = global read "COD读取DATA全局.vi" "配置文件ini"() -> (w722:string)
            n424 = call <vilib>:"Application Directory.vi"() -> ("Application Directory"=w735:path)
            n425 = Build Path(base path=w735, name or relative path=w722) -> (appended path=w734:path)
            n426 = call <vilib>:"Open Config Data.vi"("configuration file path"=w734) -> ("error out"=w730:errorcluster, "refnum"=w733:T15)  [unwired: 8 in, 1 out]
            n427 = vi-ref "斯坦道CODMn.lvlib:CODMn断电保存全局变量.vi"() -> (w732:refnum<vi>)
            n428 = call <userlib>:"Write Panel to INI__ogtk.vi"("error in (no error)"=w730, "VI ref"=w732, "refnum"=w733) -> ("error out"=w729:errorcluster, "refnum out"=w731:T15)  [unwired: 7 in]
            n429 = call <vilib>:"Close Config Data.vi"("error in (no error)"=w729, "refnum"=w731) -> ("error out"=w724:errorcluster, "file path"=w723:path)  [unwired: 8 in]
            n430 = Open/Create/Replace File(file path (use dialog)=w723, error in=w724) -> (refnum out=w727:refnum<file>, error out=w728:errorcluster)  [unwired: 4 in, 1 out]
            n431 = Flush File(refnum=w727, error in=w728) -> (refnum out=w726:refnum<file>, error out=w725:errorcluster)
            n432 = Close File(refnum=w726, error in=w725) -> ()  [unwired: 2 out]
          }
        }
      }
    }
    n433 = case shown="真" w661 {
      frame False {
      }
      frame True {
        # "排液步骤存数据，第5步数据存储时间戳更新，防止启动停止数据存储"
        n434 = call "数据写入入队列 (子VI).vi"() -> ()  [unwired: 12 in]
        n435 = local read "基本量程"() -> (w763:enum16{"L", "H"})
        n436 = global read "CODMn断电保存全局变量.vi" "启动时间"() -> (w769:timestamp)
        n437 = local read "温度"() -> (w764:dbl)
        n438 = global write "COD读取DATA全局.vi" "温度存储数据用"(w764) -> ()
        n439 = global write "COD读取DATA全局.vi" "基本量程存储数据用"(w763) -> ()
        n440 = global write "COD读取DATA全局.vi" "数据存储时间戳"(w769) -> ()
        n441 = global read "COD测量模式全局.vi" "测量模式"() -> (w768:string)
        n442 = local read "高锰酸钾"() -> (w765:dbl)
        n443 = Equal?(x=w768, y="校标") -> (x = y?=w766:bool)
        n444 = case shown="真" w766 {
          tunnel: w765 -> [_ w770]
          frame False {
          }
          frame True {
            n445 = local read "当前校准"() -> (w771:i32)
            n446 = case shown="3" w771 {
              tunnel: w770 -> [w772 w773 w774 w775 w776]
              frame 1, Default {
                n447 = local write "泵滴定数1"(w772) -> ()
              }
              frame 2 {
                n448 = local write "泵滴定数2"(w773) -> ()
              }
              frame 3 {
                n449 = local write "泵滴定数3"(w774) -> ()
              }
              frame 4 {
                n450 = local write "泵滴定数4"(w775) -> ()
              }
              frame 5 {
                n451 = local write "泵滴定数5"(w776) -> ()
              }
            }
          }
        }
      }
    }
    n452 = Wait (ms)(milliseconds to wait=u32 1000 ("等待时间（毫秒）")) -> ()  [unwired: 1 out]
  }
  n453 = while {
    stop <- FALSE stop-if-true
    # "数字键盘输入"
    n454 = event shown="[29] \"低切高阈值:\", \"高切低阈值:\": 鼠标按下" {
      selector: _ -> [_ _ _ _ _ _ _ _ _ _ _ _ _ _ _ _ _ _ _ _ _ _ _ _ _ _ _ _ _ _]
      dyn-events: _ -> [_ _ _ _ _ _ _ _ _ _ _ _ _ _ _ _ _ _ _ _ _ _ _ _ _ _ _ _ _ _]
      timeout: _ -> [_ _ _ _ _ _ _ _ _ _ _ _ _ _ _ _ _ _ _ _ _ _ _ _ _ _ _ _ _ _]
      event Timeout {
        n455 = event-data() -> ()  [unwired: 1 in, 3 out]
      }
      event "温度": Mouse Down {
        n456 = event-data() -> ()  [unwired: 1 in, 8 out]
        n457 = local read "温度"() -> (w779:dbl)
        n458 = call "数字键盘.vi"("OldNumber"=w779) -> ("NewNumber"=w778:sgl)
        n459 = local write "温度"(w778) -> ()
      }
      event "恒温时间": Mouse Down {
        n460 = event-data() -> ()  [unwired: 1 in, 8 out]
        n461 = local read "恒温时间"() -> (w780:dbl)
        n462 = call "数字键盘.vi"("OldNumber"=w780) -> ("NewNumber"=w781:sgl)
        n463 = local write "恒温时间"(w781) -> ()
      }
      event "标准液浓度": Mouse Down {
        n464 = event-data() -> ()  [unwired: 1 in, 8 out]
        n465 = local read "标准液浓度"() -> (w783:dbl)
        n466 = call "数字键盘.vi"("OldNumber"=w783) -> ("NewNumber"=w782:sgl)
        n467 = local write "标准液浓度"(w782) -> ()
      }
      event "修正系数": Mouse Down {
        n468 = event-data() -> ()  [unwired: 1 in, 8 out]
        n469 = local read "修正系数"() -> (w784:dbl)
        n470 = call "数字键盘.vi"("OldNumber"=w784) -> ("NewNumber"=w785:sgl)
        n471 = local write "修正系数"(w785) -> ()
      }
      event "水样": Mouse Down {
        n472 = event-data() -> ()  [unwired: 1 in, 8 out]
        n473 = local read "水样"() -> (w786:dbl)
        n474 = call "数字键盘.vi"("OldNumber"=w786) -> ("NewNumber"=w787:sgl)
        n475 = local write "水样"(w787) -> ()
      }
      event "蒸馏水": Mouse Down {
        n476 = event-data() -> ()  [unwired: 1 in, 8 out]
        n477 = local read "蒸馏水"() -> (w788:dbl)
        n478 = call "数字键盘.vi"("OldNumber"=w788) -> ("NewNumber"=w789:sgl)
        n479 = local write "蒸馏水"(w789) -> ()
      }
      event "标液": Mouse Down {
        n480 = event-data() -> ()  [unwired: 1 in, 8 out]
        n481 = local read "标液"() -> (w790:dbl)
        n482 = call "数字键盘.vi"("OldNumber"=w790) -> ("NewNumber"=w791:sgl)
        n483 = local write "标液"(w791) -> ()
      }
      event "质控样": Mouse Down {
        n484 = event-data() -> ()  [unwired: 1 in, 8 out]
        n485 = local read "质控样"() -> (w792:dbl)
        n486 = call "数字键盘.vi"("OldNumber"=w792) -> ("NewNumber"=w793:sgl)
        n487 = local write "质控样"(w793) -> ()
      }
      event "加标回收": Mouse Down {
        n488 = event-data() -> ()  [unwired: 1 in, 8 out]
        n489 = local read "加标回收"() -> (w794:dbl)
        n490 = call "数字键盘.vi"("OldNumber"=w794) -> ("NewNumber"=w795:sgl)
        n491 = local write "加标回收"(w795) -> ()
      }
      event "草酸钠": Mouse Down {
        n492 = event-data() -> ()  [unwired: 1 in, 8 out]
        n493 = local read "草酸钠"() -> (w796:dbl)
        n494 = call "数字键盘.vi"("OldNumber"=w796) -> ("NewNumber"=w797:sgl)
        n495 = local write "草酸钠"(w797) -> ()
      }
      event "高锰酸钾": Mouse Down {
        n496 = event-data() -> ()  [unwired: 1 in, 8 out]
        n497 = local read "高锰酸钾"() -> (w798:dbl)
        n498 = call "数字键盘.vi"("OldNumber"=w798) -> ("NewNumber"=w799:sgl)
        n499 = local write "高锰酸钾"(w799) -> ()
      }
      event "硫酸": Mouse Down {
        n500 = event-data() -> ()  [unwired: 1 in, 8 out]
        n501 = local read "硫酸"() -> (w800:dbl)
        n502 = call "数字键盘.vi"("OldNumber"=w800) -> ("NewNumber"=w801:sgl)
        n503 = local write "硫酸"(w801) -> ()
      }
      event "零点泵计量数 2": Mouse Down {
        n504 = event-data() -> ()  [unwired: 1 in, 8 out]
        n505 = local read "零点泵计量数 2"() -> (w802:dbl)
        n506 = call "数字键盘.vi"("OldNumber"=w802) -> ("NewNumber"=w803:sgl)
        n507 = local write "零点泵计量数 2"(w803) -> ()
      }
      event "标度泵计量数 2": Mouse Down {
        n508 = event-data() -> ()  [unwired: 1 in, 8 out]
        n509 = local read "标度泵计量数 2"() -> (w804:dbl)
        n510 = call "数字键盘.vi"("OldNumber"=w804) -> ("NewNumber"=w805:sgl)
        n511 = local write "标度泵计量数 2"(w805) -> ()
      }
      event "高量程稀释倍数:": Mouse Down {
        n512 = event-data() -> ()  [unwired: 1 in, 8 out]
        n513 = local read "高量程稀释倍数:"() -> (w807:i8)
        n514 = call "数字键盘.vi"("OldNumber"=w807) -> ("NewNumber"=w806:sgl)
        n515 = local write "高量程稀释倍数:"(w806) -> ()
      }
      event "低量程稀释倍数:": Mouse Down {
        n516 = event-data() -> ()  [unwired: 1 in, 8 out]
        n517 = local read "低量程稀释倍数:"() -> (w809:i8)
        n518 = call "数字键盘.vi"("OldNumber"=w809) -> ("NewNumber"=w808:sgl)
        n519 = local write "低量程稀释倍数:"(w808) -> ()
      }
      event "浓度1": Mouse Down {
        n520 = event-data() -> ()  [unwired: 1 in, 8 out]
        n521 = local read "浓度1"() -> (w811:dbl)
        n522 = call "数字键盘.vi"("OldNumber"=w811) -> ("NewNumber"=w810:sgl)
        n523 = property on="浓度1" class="DigNum (严格)"("Val(Sgnl)"=w810) -> ()  [unwired: 2 in, 2 out]
      }
      event "浓度2": Mouse Down {
        n524 = event-data() -> ()  [unwired: 1 in, 8 out]
        n525 = local read "浓度2"() -> (w813:dbl)
        n526 = call "数字键盘.vi"("OldNumber"=w813) -> ("NewNumber"=w812:sgl)
        n527 = property on="浓度2" class="DigNum (严格)"("Val(Sgnl)"=w812) -> ()  [unwired: 2 in, 2 out]
      }
      event "浓度3": Mouse Down {
        n528 = event-data() -> ()  [unwired: 1 in, 8 out]
        n529 = local read "浓度3"() -> (w815:dbl)
        n530 = call "数字键盘.vi"("OldNumber"=w815) -> ("NewNumber"=w814:sgl)
        n531 = property on="浓度3" class="DigNum (严格)"("Val(Sgnl)"=w814) -> ()  [unwired: 2 in, 2 out]
      }
      event "浓度4": Mouse Down {
        n532 = event-data() -> ()  [unwired: 1 in, 8 out]
        n533 = local read "浓度4"() -> (w817:dbl)
        n534 = call "数字键盘.vi"("OldNumber"=w817) -> ("NewNumber"=w816:sgl)
        n535 = property on="浓度4" class="DigNum (严格)"("Val(Sgnl)"=w816) -> ()  [unwired: 2 in, 2 out]
      }
      event "浓度5": Mouse Down {
        n536 = event-data() -> ()  [unwired: 1 in, 8 out]
        n537 = local read "浓度5"() -> (w819:dbl)
        n538 = call "数字键盘.vi"("OldNumber"=w819) -> ("NewNumber"=w818:sgl)
        n539 = property on="浓度5" class="DigNum (严格)"("Val(Sgnl)"=w818) -> ()  [unwired: 2 in, 2 out]
      }
      event "跨度液浓度": Mouse Down {
        n540 = event-data() -> ()  [unwired: 1 in, 8 out]
        n541 = local read "跨度液浓度"() -> (w821:dbl)
        n542 = call "数字键盘.vi"("OldNumber"=w821) -> ("NewNumber"=w820:sgl)
        n543 = property on="跨度液浓度" class="DigNum (严格)"("Val(Sgnl)"=w820) -> ()  [unwired: 2 in, 2 out]
      }
      event "跨度液浓度": Value Change {
        n544 = event-data() -> ()  [unwired: 1 in, 6 out]
        n545 = call <vilib>:"Application Directory.vi"() -> ("Application Directory"=w825:path)
        n546 = Build Path(base path=w825, name or relative path="data\\Set.ini" ("名称或相对路径")) -> (appended path=w827:path)
        n547 = local read "跨度液浓度"() -> (w822:dbl)
        n548 = call <vilib>:"Open Config Data.vi"("configuration file path"=w827) -> ("error out"=w829:errorcluster, "refnum"=w828:T15)  [unwired: 8 in, 1 out]
        n549 = call-poly <vilib>:"Write Key.vi"("section"="CODMn参数" ("key"), "error in (no error)"=w829, "value"=w822, "key"="跨度液浓度", "refnum"=w828) -> ("error out"=w831:errorcluster, "refnum out"=w830:T15)  [unwired: 4 in, 1 out]
        n550 = call <vilib>:"Close Config Data.vi"("error in (no error)"=w831, "refnum"=w830) -> ()  [unwired: 8 in, 2 out]
      }
      event "泵滴定数1": Mouse Down {
        n551 = event-data() -> ()  [unwired: 1 in, 8 out]
        n552 = local read "泵滴定数1"() -> (w833:dbl)
        n553 = call "数字键盘.vi"("OldNumber"=w833) -> ("NewNumber"=w832:sgl)
        n554 = property on="泵滴定数1" class="DigNum (严格)"("Val(Sgnl)"=w832) -> ()  [unwired: 2 in, 2 out]
      }
      event "泵滴定数2": Mouse Down {
        n555 = event-data() -> ()  [unwired: 1 in, 8 out]
        n556 = local read "泵滴定数2"() -> (w835:dbl)
        n557 = call "数字键盘.vi"("OldNumber"=w835) -> ("NewNumber"=w834:sgl)
        n558 = property on="泵滴定数2" class="DigNum (严格)"("Val(Sgnl)"=w834) -> ()  [unwired: 2 in, 2 out]
      }
      event "泵滴定数3": Mouse Down {
        n559 = event-data() -> ()  [unwired: 1 in, 8 out]
        n560 = local read "泵滴定数3"() -> (w837:dbl)
        n561 = call "数字键盘.vi"("OldNumber"=w837) -> ("NewNumber"=w836:sgl)
        n562 = property on="泵滴定数3" class="DigNum (严格)"("Val(Sgnl)"=w836) -> ()  [unwired: 2 in, 2 out]
      }
      event "泵滴定数4": Mouse Down {
        n563 = event-data() -> ()  [unwired: 1 in, 8 out]
        n564 = local read "泵滴定数4"() -> (w839:dbl)
        n565 = call "数字键盘.vi"("OldNumber"=w839) -> ("NewNumber"=w838:sgl)
        n566 = property on="泵滴定数4" class="DigNum (严格)"("Val(Sgnl)"=w838) -> ()  [unwired: 2 in, 2 out]
      }
      event "泵滴定数5": Mouse Down {
        n567 = event-data() -> ()  [unwired: 1 in, 8 out]
        n568 = local read "泵滴定数5"() -> (w841:dbl)
        n569 = call "数字键盘.vi"("OldNumber"=w841) -> ("NewNumber"=w840:sgl)
        n570 = property on="泵滴定数5" class="DigNum (严格)"("Val(Sgnl)"=w840) -> ()  [unwired: 2 in, 2 out]
      }
      event "低切高阈值:", "高切低阈值:": Mouse Down {
        n571 = event-data() -> ("CtlRef"=w845:refnum<vi>)  [unwired: 1 in, 7 out]
        n572 = property class="DigNum (严格)"(reference=w845) -> (reference out=w844:refnum<vi>, "Value"=w843:dbl)  [unwired: 1 in, 1 out]
        n573 = call "数字键盘.vi"("OldNumber"=w843) -> ("NewNumber"=w842:sgl)
        n574 = property class="DigNum (严格)"(reference=w844, "Val(Sgnl)"=w842) -> ()  [unwired: 1 in, 2 out]
      }
    }
  }
  n575 = flat-sequence {
    tunnel: [w849] -> w3
    frame #0 {
      n576 = global read "COD读取DATA全局.vi" "序列号:"() -> (w847:string)
      n577 = property on="窗格" class="Pane"("Origin"=T16 {"Horizontal"=0, "Vertical"=0} ("原点")) -> ()  [unwired: 2 in, 2 out]
      n578 = Empty String/Path?(string/path=w847) -> (empty?=w848:bool)
      n579 = case shown="假" w848 {
        tunnel: w847 -> [w866 _]
        tunnel: [w865 "data\\sys.ini" ("名称或相对路径")] -> w846
        frame False {
          # "与生产用上位机交互"
          n580 = Concatenate Strings("data\\" ("字符串"), "序列号" ("字符串"), w866, "Set.ini" ("名称或相对路径")) -> (w865:string)
        }
        frame True {
        }
      }
      n581 = call <vilib>:"Application Directory.vi"() -> ("Application Directory"=w858:path)
      n582 = local write "量程切换次数"(u8 0 ("量程切换次数")) -> ()
      n583 = local write "切换量程连续测两次"(FALSE ("切换量程连续测两次")) -> ()
      n584 = Build Path(base path=w858, name or relative path=w846) -> (appended path=w857:path)
      n585 = call <vilib>:"Open Config Data.vi"("configuration file path"=w857) -> ("error out"=w853:errorcluster, "refnum"=w856:T15)  [unwired: 8 in, 1 out]
      n586 = vi-ref "斯坦道CODMn.lvlib:CODMn断电保存全局变量.vi"() -> (w855:refnum<vi>)
      n587 = call <userlib>:"Read Panel from INI__ogtk.vi"("error in (no error)"=w853, "VI ref"=w855, "refnum"=w856) -> ("error out"=w852:errorcluster, "refnum out"=w854:T15)  [unwired: 7 in]
      n588 = call <vilib>:"Close Config Data.vi"("error in (no error)"=w852, "refnum"=w854) -> ("error out"=w851:errorcluster, "file path"=w850:path)  [unwired: 8 in]
      n589 = global write "COD读取DATA全局.vi" "配置文件ini"(w846) -> ()
      n590 = local write "选用水样"(enum16{"葡萄糖", "草酸钠"}."葡萄糖" ("选用水样")) -> ()
      n591 = local write "量程选择"(enum16{"低量程", "高量程", "0-2量程"}."低量程" ("量程选择")) -> ()
      n592 = Open/Create/Replace File(file path (use dialog)=w850, error in=w851) -> (error out=w849:errorcluster)  [unwired: 4 in, 2 out]
      "稀释倍数解释" <- "稀释倍数解释：\n稀释倍数选择1，表示不稀释\n默认低量程系数倍数1，高量程系数倍数2\n则低量程为0~8，高量程为0~16" ("稀释倍数解释")
    }
  }
  n593 = vi-ref "CODMn通讯.vi"() -> (w2:refnum<vi>)
  n594 = property class="VI"(reference=w2) -> ("Name"=w4:string)  [unwired: 1 in, 2 out]
  n595 = Open VI Reference(type specifier VI Refnum (for type only)=refnum<vi> refnum, vi path=w4, options=128 ("选项")) -> (vi reference=w6:refnum<vi>, error out=w8:errorcluster)  [unwired: 3 in]
  n596 = call-by-ref "?"(reference=w6, error in=w8) -> (reference out=w10:refnum<vi>, error out=w9:errorcluster)  [unwired: 12 in]
  n597 = Close Reference(reference=w10, error in (no error)=w9) -> ()  [unwired: 1 out]
  n598 = Obtain Queue(name (unnamed)="CODMn" ("名称（未命名）"), element data type=cluster{"命令":string} {"命令"="启用模块"} ("元素")) -> (queue out=w12:refnum<queue>, error out=w11:errorcluster)  [unwired: 3 in, 1 out]
  n599 = while {
    tunnel: w12 -> [w872]
    tunnel: w11 -> [w871]
    stop <- FALSE stop-if-true
    # "主线事件"
    n600 = event shown="[7] \"跨度液浓度\", \"常规版/认证版\", \"MB通信方式选择\": 值改变" {
      selector: _ -> [_ _ _ _ _ _ _ _ _ _ _ _ _ _ _ _ _ _ _ _ _ _ _ _ _ _ _ _ _ _ _ _]
      dyn-events: _ -> [_ _ _ _ _ _ _ _ _ _ _ _ _ _ _ _ _ _ _ _ _ _ _ _ _ _ _ _ _ _ _ _]
      timeout: _ -> [_ _ _ _ _ _ _ _ _ _ _ _ _ _ _ _ _ _ _ _ _ _ _ _ _ _ _ _ _ _ _ _]
      tunnel: w872 -> [_ _ _ _ _ w929 _ _ _ _ _ _ _ _ _ _ _ _ _ _ _ _ _ _ w1520 _ _ _ _ w1738 w1749 _]
      tunnel: w871 -> [_ _ _ _ _ w928 _ _ _ _ _ _ _ _ _ _ _ _ _ _ _ _ _ _ w1519 _ _ _ _ w1737 w1748 _]
      event "单步启动": Mouse Down {
        n601 = event-data() -> ()  [unwired: 1 in, 8 out]
        n602 = call "CODMn手动控制框.vi"() -> ()  [unwired: 12 in]
      }
      event "启动": Mouse Down {
        n603 = event-data() -> ()  [unwired: 1 in, 8 out]
        n604 = flat-sequence {
          tunnel: [w875] -> w874
          tunnel: w874 -> [w881]
          frame #0 {
            n605 = call "启动测量模式选择对话框.vi"() -> ("启动选择 2"=w875:u16)  [unwired: 11 in]
            "启动选择 2" <- w875
          }
          frame #1 {
            n606 = case shown="9, 默认" w881 {
              tunnel: [u16 4608 ("address") u16 4608 ("address") u16 4608 ("address") u16 4608 ("address") u16 4608 ("address") u16 4608 ("address") u16 4608 ("address") u16 4608 ("address") u16 4608 ("address") u16 4608 ("address")] -> w877
              tunnel: [u16 1 ("address") u16 2 ("address") u16 3 ("address") u16 4 ("address") u16 5 ("address") u16 7 ("address") u16 6 ("address") u16 8 ("address") u16 9 ("address") u16 0 ("address")] -> w882
              frame 0 {
              }
              frame 1 {
              }
              frame 2 {
              }
              frame 3 {
              }
              frame 4 {
              }
              frame 5 {
              }
              frame 6 {
              }
              frame 7 {
              }
              frame 8 {
              }
              frame 9, Default {
              }
            }
            n607 = Not Equal?(x=w881, y=u16 9) -> (x != y?=w879:bool)
            n608 = global write "CODMN外部API.vi" "手动启动CODMn"(w879) -> ()
            n609 = Insert Into Array(array=u16[] [] ("values"), index=0 ("索引"), new element=w882) -> (w876:u16[])
            n610 = call "CODMnMB_api.vi"("STEP"=enum16{"open", "read", "write", "close"}."write", "values"=w876, "starting address"=w877) -> ()  [unwired: 5 in, 4 out]
          }
        }
      }
      event "停止": Value Change {
        n611 = event-data() -> ()  [unwired: 1 in, 6 out]
        n612 = Two Button Dialog(message="确认是否停止？" ("消息"), 1:"否" ("F按钮名称（“取消”）"), 2:"是" ("T按钮名称（“确定”）")) -> (T button?=w907:bool)
        n613 = case shown="真" w907 {
          frame False {
          }
          frame True {
            n614 = call "CODMnMB_api.vi"("STEP"=enum16{"open", "read", "write", "close"}."write", "values"=u16[] [11], "starting address"=u16 4608) -> ()  [unwired: 5 in, 4 out]
          }
        }
      }
      event "手动控制": Value Change {
        n615 = event-data() -> ()  [unwired: 1 in, 6 out]
        n616 = call "数字密码键盘.vi"() -> ("NewNumber"=w912:sgl)  [unwired: 1 in]
        n617 = Equal?(x=w912, y=8.0) -> (x = y?=w913:bool)
        n618 = case shown="假" w913 {
          frame False {
            n619 = call "窗口弹出对话框(子VI).vi"("消息"="密码错误") -> ()  [unwired: 10 in, 1 out]
          }
          frame True {
          }
        }
      }
      event "锁定按钮": Mouse Down {
        n620 = event-data() -> ("CtlRef"=w918:refnum<vi>)  [unwired: 1 in, 7 out]
        n621 = property class="Bool (严格)"(reference=w918) -> ("Value"=w917:bool)  [unwired: 1 in, 2 out]
        n622 = case shown="真" w917 {
          selector: w917 -> [w919 _]
          tunnel: [w919 w920] -> w916
          frame False {
          }
          frame True {
            n623 = call "数字密码键盘.vi"() -> ("NewNumber"=w921:sgl)  [unwired: 1 in]
            n624 = Equal?(x=w921, y=8.0) -> (x = y?=w920:bool)
            n625 = case shown="假" w920 {
              selector: w920 -> [w924 _]
              frame False {
                n626 = One Button Dialog(message="密码错误!" ("消息")) -> ()  [unwired: 1 in, 1 out]
                n627 = local write "锁定按钮"(w924) -> ()
              }
              frame True {
                n628 = One Button Dialog(message="解锁成功!" ("消息")) -> ()  [unwired: 1 in, 1 out]
              }
            }
          }
        }
        "x = y?" <- w916
      }
      event "参数配置": Value Change {
        (unwired) u16 20 ("number of holding registers")
        (unwired) u16 4272 ("starting address")
        n629 = event-data() -> ()  [unwired: 1 in, 6 out]
        n630 = property on="窗格" class="Pane"("Origin"=T16 {"Horizontal"=0, "Vertical"=650} ("原点")) -> ()  [unwired: 2 in, 2 out]
        n631 = Bundle By Name(cluster=cluster{"命令":string} {"命令"=""} ("元素"), "命令"="CODMn读取参数" ("名称（未命名）")) -> (w930:cluster{"命令":string})
        n632 = Enqueue Element(queue=w929, element=w930, error in (no error)=w928) -> ()  [unwired: 1 in, 3 out]
        n633 = global read "COD读取DATA全局.vi" "配置文件ini"() -> (w926:string)
        n634 = call <vilib>:"Application Directory.vi"() -> ("Application Directory"=w933:path)
        n635 = Build Path(base path=w933, name or relative path=w926) -> (appended path=w934:path)
        n636 = call <vilib>:"Open Config Data.vi"("configuration file path"=w934) -> ("error out"=w938:errorcluster, "refnum"=w935:T15)  [unwired: 8 in, 1 out]
        n637 = vi-ref "斯坦道CODMn.lvlib:CODMn断电保存全局变量.vi"() -> (w936:refnum<vi>)
        n638 = call <userlib>:"Read Panel from INI__ogtk.vi"("error in (no error)"=w938, "VI ref"=w936, "refnum"=w935) -> ("error out"=w939:errorcluster, "refnum out"=w937:T15)  [unwired: 7 in]
        n639 = call <vilib>:"Close Config Data.vi"("error in (no error)"=w939, "refnum"=w937) -> ("error out"=w940:errorcluster, "file path"=w941:path)  [unwired: 8 in]
        n640 = Open/Create/Replace File(file path (use dialog)=w941, error in=w940) -> (error out=w927:errorcluster)  [unwired: 4 in, 2 out]
        n641 = call <vilib>:"Clear Errors.vi"("error in (no error)"=w927) -> ()  [unwired: 5 in, 2 out]
      }
      event "保存": Mouse Down {
        n642 = event-data() -> ()  [unwired: 1 in, 8 out]
        n643 = call "CODMnMB_api.vi"("STEP"=enum16{"open", "read", "write", "close"}."write", "values"="保存参数", "starting address"=u16 4272) -> ("error out"=w949:errorcluster)  [unwired: 5 in, 3 out]
        n644 = Build Array("采水泵进样时间/s:", "采水泵润洗时间/s:", "采水泵沉淀时间/s:", "采水泵排液时间/s:") -> (w943:i32[])
        n645 = call "CODMnMB_api.vi"("STEP"=enum16{"open", "read", "write", "close"}."write", "Error in"=w949, "values"=w943, "starting address"=u16 5596) -> ()  [unwired: 4 in, 4 out]
      }
      event "跨度液浓度", "常规版/认证版", "MB通信方式选择": Value Change {
        n646 = event-data() -> ()  [unwired: 1 in, 6 out]
        n647 = flat-sequence {
          frame #0 {
            n648 = global write "CODMn断电保存全局变量.vi" "常规版/认证版"("常规版/认证版") -> ()
            n649 = global write "CODMn断电保存全局变量.vi" "跨度液浓度"("跨度液浓度") -> ()
            n650 = global write "CODMn断电保存全局变量.vi" "MB通信方式选择"("MB通信方式选择") -> ()
          }
          frame #1 {
            n651 = global read "COD读取DATA全局.vi" "配置文件ini"() -> (w957:string)
            n652 = call <vilib>:"Application Directory.vi"() -> ("Application Directory"=w970:path)
            n653 = Build Path(base path=w970, name or relative path=w957) -> (appended path=w969:path)
            n654 = call <vilib>:"Open Config Data.vi"("configuration file path"=w969) -> ("error out"=w965:errorcluster, "refnum"=w968:T15)  [unwired: 8 in, 1 out]
            n655 = vi-ref "斯坦道CODMn.lvlib:CODMn断电保存全局变量.vi"() -> (w967:refnum<vi>)
            n656 = call <userlib>:"Write Panel to INI__ogtk.vi"("error in (no error)"=w965, "VI ref"=w967, "refnum"=w968) -> ("error out"=w964:errorcluster, "refnum out"=w966:T15)  [unwired: 7 in]
            n657 = call <vilib>:"Close Config Data.vi"("error in (no error)"=w964, "refnum"=w966) -> ("error out"=w959:errorcluster, "file path"=w958:path)  [unwired: 8 in]
            n658 = Open/Create/Replace File(file path (use dialog)=w958, error in=w959) -> (refnum out=w962:refnum<file>, error out=w963:errorcluster)  [unwired: 4 in, 1 out]
            n659 = Flush File(refnum=w962, error in=w963) -> (refnum out=w961:refnum<file>, error out=w960:errorcluster)
            n660 = Close File(refnum=w961, error in=w960) -> ()  [unwired: 2 out]
          }
        }
      }
      event "校准配置": Value Change {
        n661 = event-data() -> ()  [unwired: 1 in, 6 out]
        n662 = property on="窗格" class="Pane"("Origin"=T16 {"Horizontal"=0, "Vertical"=1300} ("原点")) -> ()  [unwired: 2 in, 2 out]
        n663 = global read "COD读取DATA全局.vi" "配置文件ini"() -> (w971:string)
        n664 = call <vilib>:"Application Directory.vi"() -> ("Application Directory"=w1021:path)
        n665 = Build Path(base path=w1021, name or relative path=w971) -> (appended path=w1020:path)
        n666 = call <vilib>:"Open Config Data.vi"("configuration file path"=w1020) -> ("error out"=w990:errorcluster, "refnum"=w991:T15)  [unwired: 8 in, 1 out]
        n667 = local read "量程选择"() -> (w997:enum16{"低量程", "高量程", "0-2量程"})
        n668 = call-poly <vilib>:"Read Key.vi"("section"="CODMn模型选择" ("key"), "error in (no error)"=w990, "key"="线性和多项式", "refnum"=w991) -> ("error out"=w987:errorcluster, "value"=w989:i32, "refnum out"=w988:T15)  [unwired: 4 in, 1 out]
        n669 = case shown="\"0-2量程\"" w997 {
          tunnel: ["低量程" "高量程" "0-2量程"] -> w995
          frame "低量程", Default {
          }
          frame "高量程" {
          }
          frame "0-2量程" {
          }
        }
        n670 = local write "模型"(w989) -> ()
        n671 = call-poly <vilib>:"Read Key.vi"("section"="标线选择", "error in (no error)"=w987, "key"="选用水样", "refnum"=w988) -> ("error out"=w985:errorcluster, "value"=w972:i32, "refnum out"=w986:T15)  [unwired: 4 in, 1 out]
        n672 = case shown="0, 默认" w972 {
          tunnel: ["葡萄糖标线" ("section") "草酸钠标线" ("section")] -> w996
          frame 0, Default {
          }
          frame 1 {
          }
        }
        n673 = local write "选用水样"(w972) -> ()
        n674 = Concatenate Strings(w996, w995) -> (w994:string)
        n675 = call-poly <vilib>:"Read Key.vi"("section"=w994, "error in (no error)"=w985, "key"="浓度1", "refnum"=w986) -> ("error out"=w1025:errorcluster, "value"=w1023:dbl, "refnum out"=w1024:T15)  [unwired: 4 in, 1 out]
        n676 = local write "浓度1"(w1023) -> ()
        n677 = call-poly <vilib>:"Read Key.vi"("section"=w994, "error in (no error)"=w1025, "key"="浓度2", "refnum"=w1024) -> ("error out"=w1039:errorcluster, "value"=w1026:dbl, "refnum out"=w1038:T15)  [unwired: 4 in, 1 out]
        n678 = local write "浓度2"(w1026) -> ()
        n679 = call-poly <vilib>:"Read Key.vi"("section"=w994, "error in (no error)"=w1039, "key"="浓度3", "refnum"=w1038) -> ("error out"=w1040:errorcluster, "value"=w1028:dbl, "refnum out"=w1037:T15)  [unwired: 4 in, 1 out]
        n680 = local write "浓度3"(w1028) -> ()
        n681 = call-poly <vilib>:"Read Key.vi"("section"=w994, "error in (no error)"=w1040, "key"="泵滴定数1", "refnum"=w1037) -> ("error out"=w1041:errorcluster, "value"=w1030:dbl, "refnum out"=w1036:T15)  [unwired: 4 in, 1 out]
        n682 = local write "泵滴定数1"(w1030) -> ()
        n683 = call-poly <vilib>:"Read Key.vi"("section"=w994, "error in (no error)"=w1041, "key"="泵滴定数2", "refnum"=w1036) -> ("error out"=w1035:errorcluster, "value"=w1033:dbl, "refnum out"=w1042:T15)  [unwired: 4 in, 1 out]
        n684 = local write "泵滴定数2"(w1033) -> ()
        n685 = call-poly <vilib>:"Read Key.vi"("section"=w994, "error in (no error)"=w1035, "key"="泵滴定数3", "refnum"=w1042) -> ("error out"=w1047:errorcluster, "value"=w1046:dbl, "refnum out"=w1043:T15)  [unwired: 4 in, 1 out]
        n686 = local write "泵滴定数3"(w1046) -> ()
        n687 = call-poly <vilib>:"Read Key.vi"("section"=w994, "error in (no error)"=w1047, "key"="浓度4", "refnum"=w1043) -> ("error out"=w1048:errorcluster, "value"=w978:dbl, "refnum out"=w1044:T15)  [unwired: 4 in, 1 out]
        n688 = local write "浓度4"(w978) -> ()
        n689 = call-poly <vilib>:"Read Key.vi"("section"=w994, "error in (no error)"=w1048, "key"="浓度5", "refnum"=w1044) -> ("error out"=w983:errorcluster, "value"=w977:dbl, "refnum out"=w984:T15)  [unwired: 4 in, 1 out]
        n690 = local write "浓度5"(w977) -> ()
        n691 = call-poly <vilib>:"Read Key.vi"("section"=w994, "error in (no error)"=w983, "key"="泵滴定数4", "refnum"=w984) -> ("error out"=w1049:errorcluster, "value"=w976:dbl, "refnum out"=w1045:T15)  [unwired: 4 in, 1 out]
        n692 = local write "泵滴定数4"(w976) -> ()
        n693 = call-poly <vilib>:"Read Key.vi"("section"=w994, "error in (no error)"=w1049, "key"="泵滴定数5", "refnum"=w1045) -> ("error out"=w981:errorcluster, "value"=w975:dbl, "refnum out"=w982:T15)  [unwired: 4 in, 1 out]
        n694 = local write "泵滴定数5"(w975) -> ()
        n695 = call-poly <vilib>:"Read Key.vi"("section"=w994, "error in (no error)"=w981, "key"="当前选用的校准", "refnum"=w982) -> ("error out"=w1016:errorcluster, "value"=w1018:i32, "refnum out"=w1017:T15)  [unwired: 4 in, 1 out]
        n696 = local write "当前校准"(w1018) -> ()
        n697 = call-poly <vilib>:"Read Key.vi"("section"=w994, "error in (no error)"=w1016, "key"="启用1", "refnum"=w1017) -> ("error out"=w1013:errorcluster, "value"=w1002:bool, "refnum out"=w1014:T15)  [unwired: 4 in, 1 out]
        n698 = local write "启用1"(w1002) -> ()
        n699 = call-poly <vilib>:"Read Key.vi"("section"=w994, "error in (no error)"=w1013, "key"="启用2", "refnum"=w1014) -> ("error out"=w1011:errorcluster, "value"=w1001:bool, "refnum out"=w1012:T15)  [unwired: 4 in, 1 out]
        n700 = local write "启用2"(w1001) -> ()
        n701 = call-poly <vilib>:"Read Key.vi"("section"=w994, "error in (no error)"=w1011, "key"="启用3", "refnum"=w1012) -> ("error out"=w1009:errorcluster, "value"=w1000:bool, "refnum out"=w1010:T15)  [unwired: 4 in, 1 out]
        n702 = local write "启用3"(w1000) -> ()
        n703 = call-poly <vilib>:"Read Key.vi"("section"=w994, "error in (no error)"=w1009, "key"="启用4", "refnum"=w1010) -> ("error out"=w1007:errorcluster, "value"=w974:bool, "refnum out"=w1008:T15)  [unwired: 4 in, 1 out]
        n704 = local write "启用4"(w974) -> ()
        n705 = call-poly <vilib>:"Read Key.vi"("section"=w994, "error in (no error)"=w1007, "key"="启用5", "refnum"=w1008) -> ("error out"=w979:errorcluster, "value"=w973:bool, "refnum out"=w980:T15)  [unwired: 4 in, 1 out]
        n706 = local write "启用5"(w973) -> ()
        n707 = call <vilib>:"Close Config Data.vi"("error in (no error)"=w979, "refnum"=w980) -> ()  [unwired: 8 in, 2 out]
      }
      event "选用水样": Value Change {
        (unwired) "浓度6" ("key")
        n708 = event-data() -> ()  [unwired: 1 in, 6 out]
        n709 = property on="窗格" class="Pane"("Origin"=T16 {"Horizontal"=0, "Vertical"=1300} ("原点")) -> ()  [unwired: 2 in, 2 out]
        n710 = local read "量程选择"() -> (w1074:enum16{"低量程", "高量程", "0-2量程"})
        n711 = global read "COD读取DATA全局.vi" "配置文件ini"() -> (w1060:string)
        n712 = case shown="\"0-2量程\"" w1074 {
          tunnel: ["低量程" "高量程" "0-2量程"] -> w1075
          frame "低量程", Default {
          }
          frame "高量程" {
          }
          frame "0-2量程" {
          }
        }
        n713 = case shown="\"葡萄糖\", 默认" "选用水样" {
          tunnel: ["葡萄糖标线" ("section") "草酸钠标线" ("section")] -> w1076
          frame "葡萄糖", Default {
          }
          frame "草酸钠" {
          }
        }
        n714 = call <vilib>:"Application Directory.vi"() -> ("Application Directory"=w1099:path)
        n715 = Build Path(base path=w1099, name or relative path=w1060) -> (appended path=w1098:path)
        n716 = call <vilib>:"Open Config Data.vi"("configuration file path"=w1098) -> ("error out"=w1100:errorcluster, "refnum"=w1101:T15)  [unwired: 8 in, 1 out]
        n717 = Concatenate Strings(w1076, w1075) -> (w1073:string)
        n718 = call-poly <vilib>:"Read Key.vi"("section"=w1073, "error in (no error)"=w1100, "key"="浓度1", "refnum"=w1101) -> ("error out"=w1105:errorcluster, "value"=w1103:dbl, "refnum out"=w1104:T15)  [unwired: 4 in, 1 out]
        n719 = local write "浓度1"(w1103) -> ()
        n720 = call-poly <vilib>:"Read Key.vi"("section"=w1073, "error in (no error)"=w1105, "key"="浓度2", "refnum"=w1104) -> ("error out"=w1119:errorcluster, "value"=w1106:dbl, "refnum out"=w1118:T15)  [unwired: 4 in, 1 out]
        n721 = local write "浓度2"(w1106) -> ()
        n722 = call-poly <vilib>:"Read Key.vi"("section"=w1073, "error in (no error)"=w1119, "key"="浓度3", "refnum"=w1118) -> ("error out"=w1120:errorcluster, "value"=w1108:dbl, "refnum out"=w1117:T15)  [unwired: 4 in, 1 out]
        n723 = local write "浓度3"(w1108) -> ()
        n724 = call-poly <vilib>:"Read Key.vi"("section"=w1073, "error in (no error)"=w1120, "key"="泵滴定数1", "refnum"=w1117) -> ("error out"=w1121:errorcluster, "value"=w1110:dbl, "refnum out"=w1116:T15)  [unwired: 4 in, 1 out]
        n725 = local write "泵滴定数1"(w1110) -> ()
        n726 = call-poly <vilib>:"Read Key.vi"("section"=w1073, "error in (no error)"=w1121, "key"="泵滴定数2", "refnum"=w1116) -> ("error out"=w1115:errorcluster, "value"=w1113:dbl, "refnum out"=w1122:T15)  [unwired: 4 in, 1 out]
        n727 = local write "泵滴定数2"(w1113) -> ()
        n728 = call-poly <vilib>:"Read Key.vi"("section"=w1073, "error in (no error)"=w1115, "key"="泵滴定数3", "refnum"=w1122) -> ("error out"=w1127:errorcluster, "value"=w1126:dbl, "refnum out"=w1123:T15)  [unwired: 4 in, 1 out]
        n729 = local write "泵滴定数3"(w1126) -> ()
        n730 = call-poly <vilib>:"Read Key.vi"("section"=w1073, "error in (no error)"=w1127, "key"="浓度4", "refnum"=w1123) -> ("error out"=w1128:errorcluster, "value"=w1068:dbl, "refnum out"=w1124:T15)  [unwired: 4 in, 1 out]
        n731 = local write "浓度4"(w1068) -> ()
        n732 = call-poly <vilib>:"Read Key.vi"("section"=w1073, "error in (no error)"=w1128, "key"="浓度5", "refnum"=w1124) -> ("error out"=w1071:errorcluster, "value"=w1067:dbl, "refnum out"=w1072:T15)  [unwired: 4 in, 1 out]
        n733 = local write "浓度5"(w1067) -> ()
        n734 = call-poly <vilib>:"Read Key.vi"("section"=w1073, "error in (no error)"=w1071, "key"="泵滴定数4", "refnum"=w1072) -> ("error out"=w1129:errorcluster, "value"=w1066:dbl, "refnum out"=w1125:T15)  [unwired: 4 in, 1 out]
        n735 = local write "泵滴定数4"(w1066) -> ()
        n736 = call-poly <vilib>:"Read Key.vi"("section"=w1073, "error in (no error)"=w1129, "key"="泵滴定数5", "refnum"=w1125) -> ("error out"=w1069:errorcluster, "value"=w1065:dbl, "refnum out"=w1070:T15)  [unwired: 4 in, 1 out]
        n737 = local write "泵滴定数5"(w1065) -> ()
        n738 = call-poly <vilib>:"Read Key.vi"("section"=w1073, "error in (no error)"=w1069, "key"="当前选用的校准", "refnum"=w1070) -> ("error out"=w1094:errorcluster, "value"=w1096:i32, "refnum out"=w1095:T15)  [unwired: 4 in, 1 out]
        n739 = call-poly <vilib>:"Read Key.vi"("section"=w1073, "error in (no error)"=w1094, "key"="启用1", "refnum"=w1095) -> ("error out"=w1091:errorcluster, "value"=w1080:bool, "refnum out"=w1092:T15)  [unwired: 4 in, 1 out]
        n740 = local write "当前校准"(w1096) -> ()
        n741 = local write "启用1"(w1080) -> ()
        n742 = call-poly <vilib>:"Read Key.vi"("section"=w1073, "error in (no error)"=w1091, "key"="启用2", "refnum"=w1092) -> ("error out"=w1089:errorcluster, "value"=w1079:bool, "refnum out"=w1090:T15)  [unwired: 4 in, 1 out]
        n743 = local write "启用2"(w1079) -> ()
        n744 = call-poly <vilib>:"Read Key.vi"("section"=w1073, "error in (no error)"=w1089, "key"="启用3", "refnum"=w1090) -> ("error out"=w1087:errorcluster, "value"=w1078:bool, "refnum out"=w1088:T15)  [unwired: 4 in, 1 out]
        n745 = local write "启用3"(w1078) -> ()
        n746 = call-poly <vilib>:"Read Key.vi"("section"=w1073, "error in (no error)"=w1087, "key"="启用4", "refnum"=w1088) -> ("error out"=w1085:errorcluster, "value"=w1062:bool, "refnum out"=w1086:T15)  [unwired: 4 in, 1 out]
        n747 = local write "启用4"(w1062) -> ()
        n748 = call-poly <vilib>:"Read Key.vi"("section"=w1073, "error in (no error)"=w1085, "key"="启用5", "refnum"=w1086) -> ("error out"=w1063:errorcluster, "value"=w1061:bool, "refnum out"=w1064:T15)  [unwired: 4 in, 1 out]
        n749 = local write "启用5"(w1061) -> ()
        n750 = call <vilib>:"Close Config Data.vi"("error in (no error)"=w1063, "refnum"=w1064) -> ()  [unwired: 8 in, 2 out]
      }
      event "量程选择": Value Change {
        n751 = event-data() -> ()  [unwired: 1 in, 6 out]
        n752 = local read "选用水样"() -> (w1157:enum16{"葡萄糖", "草酸钠"})
        n753 = global read "COD读取DATA全局.vi" "配置文件ini"() -> (w1140:string)
        n754 = property on="窗格" class="Pane"("Origin"=T16 {"Horizontal"=0, "Vertical"=1300} ("原点")) -> ()  [unwired: 2 in, 2 out]
        n755 = case shown="\"葡萄糖\", 默认" w1157 {
          tunnel: ["葡萄糖标线" ("section") "草酸钠标线" ("section")] -> w1156
          frame "葡萄糖", Default {
          }
          frame "草酸钠" {
          }
        }
        n756 = case shown="\"0-2量程\"" "量程选择" {
          tunnel: ["低量程" "高量程" "0-2量程"] -> w1153
          frame "低量程", Default {
          }
          frame "高量程" {
          }
          frame "0-2量程" {
          }
        }
        n757 = call <vilib>:"Application Directory.vi"() -> ("Application Directory"=w1179:path)
        n758 = Build Path(base path=w1179, name or relative path=w1140) -> (appended path=w1178:path)
        n759 = call <vilib>:"Open Config Data.vi"("configuration file path"=w1178) -> ("error out"=w1180:errorcluster, "refnum"=w1181:T15)  [unwired: 8 in, 1 out]
        n760 = Concatenate Strings(w1156, w1153) -> (w1155:string)
        n761 = call-poly <vilib>:"Read Key.vi"("section"=w1155, "error in (no error)"=w1180, "key"="浓度1", "refnum"=w1181) -> ("error out"=w1185:errorcluster, "value"=w1183:dbl, "refnum out"=w1184:T15)  [unwired: 4 in, 1 out]
        n762 = local write "浓度1"(w1183) -> ()
        n763 = call-poly <vilib>:"Read Key.vi"("section"=w1155, "error in (no error)"=w1185, "key"="浓度2", "refnum"=w1184) -> ("error out"=w1199:errorcluster, "value"=w1186:dbl, "refnum out"=w1198:T15)  [unwired: 4 in, 1 out]
        n764 = local write "浓度2"(w1186) -> ()
        n765 = call-poly <vilib>:"Read Key.vi"("section"=w1155, "error in (no error)"=w1199, "key"="浓度3", "refnum"=w1198) -> ("error out"=w1200:errorcluster, "value"=w1188:dbl, "refnum out"=w1197:T15)  [unwired: 4 in, 1 out]
        n766 = local write "浓度3"(w1188) -> ()
        n767 = call-poly <vilib>:"Read Key.vi"("section"=w1155, "error in (no error)"=w1200, "key"="泵滴定数1", "refnum"=w1197) -> ("error out"=w1201:errorcluster, "value"=w1190:dbl, "refnum out"=w1196:T15)  [unwired: 4 in, 1 out]
        n768 = local write "泵滴定数1"(w1190) -> ()
        n769 = call-poly <vilib>:"Read Key.vi"("section"=w1155, "error in (no error)"=w1201, "key"="泵滴定数2", "refnum"=w1196) -> ("error out"=w1195:errorcluster, "value"=w1193:dbl, "refnum out"=w1202:T15)  [unwired: 4 in, 1 out]
        n770 = local write "泵滴定数2"(w1193) -> ()
        n771 = call-poly <vilib>:"Read Key.vi"("section"=w1155, "error in (no error)"=w1195, "key"="泵滴定数3", "refnum"=w1202) -> ("error out"=w1207:errorcluster, "value"=w1206:dbl, "refnum out"=w1203:T15)  [unwired: 4 in, 1 out]
        n772 = local write "泵滴定数3"(w1206) -> ()
        n773 = call-poly <vilib>:"Read Key.vi"("section"=w1155, "error in (no error)"=w1207, "key"="浓度4", "refnum"=w1203) -> ("error out"=w1208:errorcluster, "value"=w1144:dbl, "refnum out"=w1204:T15)  [unwired: 4 in, 1 out]
        n774 = local write "浓度4"(w1144) -> ()
        n775 = call-poly <vilib>:"Read Key.vi"("section"=w1155, "error in (no error)"=w1208, "key"="浓度5", "refnum"=w1204) -> ("error out"=w1151:errorcluster, "value"=w1143:dbl, "refnum out"=w1152:T15)  [unwired: 4 in, 1 out]
        n776 = local write "浓度5"(w1143) -> ()
        n777 = call-poly <vilib>:"Read Key.vi"("section"=w1155, "error in (no error)"=w1151, "key"="泵滴定数4", "refnum"=w1152) -> ("error out"=w1209:errorcluster, "value"=w1142:dbl, "refnum out"=w1205:T15)  [unwired: 4 in, 1 out]
        n778 = local write "泵滴定数4"(w1142) -> ()
        n779 = call-poly <vilib>:"Read Key.vi"("section"=w1155, "error in (no error)"=w1209, "key"="泵滴定数5", "refnum"=w1205) -> ("error out"=w1149:errorcluster, "value"=w1141:dbl, "refnum out"=w1150:T15)  [unwired: 4 in, 1 out]
        n780 = local write "泵滴定数5"(w1141) -> ()
        n781 = call-poly <vilib>:"Read Key.vi"("section"=w1155, "error in (no error)"=w1149, "key"="当前选用的校准", "refnum"=w1150) -> ("error out"=w1174:errorcluster, "value"=w1176:i32, "refnum out"=w1175:T15)  [unwired: 4 in, 1 out]
        n782 = local write "当前校准"(w1176) -> ()
        n783 = call-poly <vilib>:"Read Key.vi"("section"=w1155, "error in (no error)"=w1174, "key"="启用1", "refnum"=w1175) -> ("error out"=w1171:errorcluster, "value"=w1160:bool, "refnum out"=w1172:T15)  [unwired: 4 in, 1 out]
        n784 = local write "启用1"(w1160) -> ()
        n785 = call-poly <vilib>:"Read Key.vi"("section"=w1155, "error in (no error)"=w1171, "key"="启用2", "refnum"=w1172) -> ("error out"=w1169:errorcluster, "value"=w1159:bool, "refnum out"=w1170:T15)  [unwired: 4 in, 1 out]
        n786 = local write "启用2"(w1159) -> ()
        n787 = call-poly <vilib>:"Read Key.vi"("section"=w1155, "error in (no error)"=w1169, "key"="启用3", "refnum"=w1170) -> ("error out"=w1167:errorcluster, "value"=w1158:bool, "refnum out"=w1168:T15)  [unwired: 4 in, 1 out]
        n788 = local write "启用3"(w1158) -> ()
        n789 = call-poly <vilib>:"Read Key.vi"("section"=w1155, "error in (no error)"=w1167, "key"="启用4", "refnum"=w1168) -> ("error out"=w1165:errorcluster, "value"=w1146:bool, "refnum out"=w1166:T15)  [unwired: 4 in, 1 out]
        n790 = local write "启用4"(w1146) -> ()
        n791 = call-poly <vilib>:"Read Key.vi"("section"=w1155, "error in (no error)"=w1165, "key"="启用5", "refnum"=w1166) -> ("error out"=w1147:errorcluster, "value"=w1145:bool, "refnum out"=w1148:T15)  [unwired: 4 in, 1 out]
        n792 = local write "启用5"(w1145) -> ()
        n793 = call <vilib>:"Close Config Data.vi"("error in (no error)"=w1147, "refnum"=w1148) -> ()  [unwired: 8 in, 2 out]
      }
      event "返回": Value Change {
        w1234 = "CODMn" ("section")
        n794 = event-data() -> ()  [unwired: 1 in, 6 out]
        n795 = global read "COD读取DATA全局.vi" "配置文件ini"() -> (w1220:string)
        n796 = property on="窗格" class="Pane"("Origin"=T16 {"Horizontal"=0, "Vertical"=0} ("原点")) -> ()  [unwired: 2 in, 2 out]
        n797 = call <vilib>:"Application Directory.vi"() -> ("Application Directory"=w1286:path)
        n798 = Build Path(base path=w1286, name or relative path=w1220) -> (appended path=w1285:path)
        n799 = local read "浓度1"() -> (w1281:dbl)
        n800 = call <vilib>:"Open Config Data.vi"("configuration file path"=w1285) -> ("error out"=w1283:errorcluster, "refnum"=w1284:T15)  [unwired: 8 in, 1 out]
        n801 = local read "浓度2"() -> (w1265:dbl)
        n802 = call-poly <vilib>:"Write Key.vi"("section"=w1234, "error in (no error)"=w1283, "value"=w1281, "key"="浓度1", "refnum"=w1284) -> ("error out"=w1280:errorcluster, "refnum out"=w1279:T15)  [unwired: 4 in, 1 out]
        n803 = local read "浓度3"() -> (w1261:dbl)
        n804 = call-poly <vilib>:"Write Key.vi"("section"=w1234, "error in (no error)"=w1280, "value"=w1265, "key"="浓度2", "refnum"=w1279) -> ("error out"=w1278:errorcluster, "refnum out"=w1277:T15)  [unwired: 4 in, 1 out]
        n805 = local read "泵滴定数1"() -> (w1259:dbl)
        n806 = call-poly <vilib>:"Write Key.vi"("section"=w1234, "error in (no error)"=w1278, "value"=w1261, "key"="浓度3", "refnum"=w1277) -> ("error out"=w1276:errorcluster, "refnum out"=w1275:T15)  [unwired: 4 in, 1 out]
        n807 = call-poly <vilib>:"Write Key.vi"("section"=w1234, "error in (no error)"=w1276, "value"=w1259, "key"="泵滴定数1", "refnum"=w1275) -> ("error out"=w1274:errorcluster, "refnum out"=w1273:T15)  [unwired: 4 in, 1 out]
        n808 = local read "泵滴定数2"() -> (w1257:dbl)
        n809 = call-poly <vilib>:"Write Key.vi"("section"=w1234, "error in (no error)"=w1274, "value"=w1257, "key"="泵滴定数2", "refnum"=w1273) -> ("error out"=w1272:errorcluster, "refnum out"=w1271:T15)  [unwired: 4 in, 1 out]
        n810 = local read "泵滴定数3"() -> (w1255:dbl)
        n811 = local read "浓度4"() -> (w1222:dbl)
        n812 = call-poly <vilib>:"Write Key.vi"("section"=w1234, "error in (no error)"=w1272, "value"=w1255, "key"="泵滴定数3", "refnum"=w1271) -> ("error out"=w1270:errorcluster, "refnum out"=w1269:T15)  [unwired: 4 in, 1 out]
        n813 = call-poly <vilib>:"Write Key.vi"("section"=w1234, "error in (no error)"=w1270, "value"=w1222, "key"="浓度4", "refnum"=w1269) -> ("error out"=w1263:errorcluster, "refnum out"=w1264:T15)  [unwired: 4 in, 1 out]
        n814 = local read "浓度5"() -> (w1221:dbl)
        n815 = call-poly <vilib>:"Write Key.vi"("section"=w1234, "error in (no error)"=w1263, "value"=w1221, "key"="浓度5", "refnum"=w1264) -> ("error out"=w1231:errorcluster, "refnum out"=w1232:T15)  [unwired: 4 in, 1 out]
        n816 = local read "泵滴定数4"() -> (w1223:dbl)
        n817 = call-poly <vilib>:"Write Key.vi"("section"=w1234, "error in (no error)"=w1231, "value"=w1223, "key"="泵滴定数4", "refnum"=w1232) -> ("error out"=w1268:errorcluster, "refnum out"=w1267:T15)  [unwired: 4 in, 1 out]
        n818 = local read "泵滴定数5"() -> (w1224:dbl)
        n819 = call-poly <vilib>:"Write Key.vi"("section"=w1234, "error in (no error)"=w1268, "value"=w1224, "key"="泵滴定数5", "refnum"=w1267) -> ("error out"=w1229:errorcluster, "refnum out"=w1230:T15)  [unwired: 4 in, 1 out]
        n820 = local read "启用1"() -> (w1243:bool)
        n821 = call-poly <vilib>:"Write Key.vi"("section"=w1234, "error in (no error)"=w1229, "value"=w1243, "key"="启用1", "refnum"=w1230) -> ("error out"=w1239:errorcluster, "refnum out"=w1242:T15)  [unwired: 4 in, 1 out]
        n822 = local read "启用2"() -> (w1240:bool)
        n823 = call-poly <vilib>:"Write Key.vi"("section"=w1234, "error in (no error)"=w1239, "value"=w1240, "key"="启用2", "refnum"=w1242) -> ("error out"=w1250:errorcluster, "refnum out"=w1249:T15)  [unwired: 4 in, 1 out]
        n824 = local read "启用3"() -> (w1238:bool)
        n825 = call-poly <vilib>:"Write Key.vi"("section"=w1234, "error in (no error)"=w1250, "value"=w1238, "key"="启用3", "refnum"=w1249) -> ("error out"=w1248:errorcluster, "refnum out"=w1247:T15)  [unwired: 4 in, 1 out]
        n826 = local read "启用4"() -> (w1226:bool)
        n827 = call-poly <vilib>:"Write Key.vi"("section"=w1234, "error in (no error)"=w1248, "value"=w1226, "key"="启用4", "refnum"=w1247) -> ("error out"=w1246:errorcluster, "refnum out"=w1245:T15)  [unwired: 4 in, 1 out]
        n828 = local read "启用5"() -> (w1225:bool)
        n829 = call-poly <vilib>:"Write Key.vi"("section"=w1234, "error in (no error)"=w1246, "value"=w1225, "key"="启用5", "refnum"=w1245) -> ("error out"=w1227:errorcluster, "refnum out"=w1228:T15)  [unwired: 4 in, 1 out]
        n830 = call <vilib>:"Close Config Data.vi"("error in (no error)"=w1227, "refnum"=w1228) -> ()  [unwired: 8 in, 2 out]
      }
      event "关闭", "关闭 2", "关闭 3": Value Change {
        n831 = event-data() -> ()  [unwired: 1 in, 6 out]
        n832 = property on="窗格" class="Pane"("Origin"=T16 {"Horizontal"=0, "Vertical"=0} ("原点")) -> ()  [unwired: 2 in, 2 out]
      }
      event Application Instance Close {
        n833 = event-data() -> ()  [unwired: 1 in, 4 out]
      }
      event "时间校准": Value Change {
        n834 = event-data() -> ()  [unwired: 1 in, 6 out]
        n835 = Get Date/Time In Seconds() -> (seconds since 1Jan1904=w1296:timestamp)
        n836 = Build Array(w1296) -> (w1295:timestamp[])
        n837 = call "DateToHex.vi"("DATE"=w1295) -> ("数组"=w1293:u16[])  [unwired: 10 in]
        n838 = Insert Into Array(array=u16[] [1] ("values"), index=1 ("索引"), new element=w1293) -> (w1289:u16[])
        n839 = call "CODMnMB_api.vi"("STEP"=enum16{"open", "read", "write", "close"}."write", "values"=w1289, "starting address"=u16 4612) -> ("error out"=w1288:errorcluster)  [unwired: 5 in, 3 out]
        n840 = call <vilib>:"Clear Errors.vi"("error in (no error)"=w1288) -> ()  [unwired: 5 in, 2 out]
      }
      event "故障清除": Value Change {
        n841 = event-data() -> ()  [unwired: 1 in, 6 out]
        n842 = call "CODMnMB_api.vi"("STEP"=enum16{"open", "read", "write", "close"}."write", "values"=u16[] [1], "starting address"=u16 4611) -> ()  [unwired: 5 in, 4 out]
      }
      event "定时启动": Mouse Down {
        n843 = event-data() -> ()  [unwired: 1 in, 8 out]
        n844 = flat-sequence {
          frame #0 {
            n845 = global read "CODMn断电保存全局变量.vi" "定时控制"() -> (w1301:T9)
            n846 = call "周期设置.vi"("定时控制参数输入"=w1301) -> ("定时控制参数输出"=w1300:T9)  [unwired: 10 in]
            n847 = global write "CODMn断电保存全局变量.vi" "定时控制"(w1300) -> ()
          }
          frame #1 {
            n848 = global read "COD读取DATA全局.vi" "配置文件ini"() -> (w1302:string)
            n849 = call <vilib>:"Application Directory.vi"() -> ("Application Directory"=w1315:path)
            n850 = Build Path(base path=w1315, name or relative path=w1302) -> (appended path=w1314:path)
            n851 = call <vilib>:"Open Config Data.vi"("configuration file path"=w1314) -> ("error out"=w1310:errorcluster, "refnum"=w1313:T15)  [unwired: 8 in, 1 out]
            n852 = vi-ref "斯坦道CODMn.lvlib:CODMn断电保存全局变量.vi"() -> (w1312:refnum<vi>)
            n853 = call <userlib>:"Write Panel to INI__ogtk.vi"("error in (no error)"=w1310, "VI ref"=w1312, "refnum"=w1313) -> ("error out"=w1309:errorcluster, "refnum out"=w1311:T15)  [unwired: 7 in]
            n854 = call <vilib>:"Close Config Data.vi"("error in (no error)"=w1309, "refnum"=w1311) -> ("error out"=w1304:errorcluster, "file path"=w1303:path)  [unwired: 8 in]
            n855 = Open/Create/Replace File(file path (use dialog)=w1303, error in=w1304) -> (refnum out=w1307:refnum<file>, error out=w1308:errorcluster)  [unwired: 4 in, 1 out]
            n856 = Flush File(refnum=w1307, error in=w1308) -> (refnum out=w1306:refnum<file>, error out=w1305:errorcluster)
            n857 = Close File(refnum=w1306, error in=w1305) -> ()  [unwired: 2 out]
          }
        }
      }
      event "测量模式(公式)": Value Change {
        n858 = event-data() -> ()  [unwired: 1 in, 6 out]
        n859 = flat-sequence {
          frame #0 {
            n860 = global write "CODMn断电保存全局变量.vi" "测量模式(公式)"("测量模式(公式)") -> ()
          }
          frame #1 {
            n861 = global read "COD读取DATA全局.vi" "配置文件ini"() -> (w1317:string)
            n862 = call <vilib>:"Application Directory.vi"() -> ("Application Directory"=w1330:path)
            n863 = Build Path(base path=w1330, name or relative path=w1317) -> (appended path=w1329:path)
            n864 = call <vilib>:"Open Config Data.vi"("configuration file path"=w1329) -> ("error out"=w1325:errorcluster, "refnum"=w1328:T15)  [unwired: 8 in, 1 out]
            n865 = vi-ref "斯坦道CODMn.lvlib:CODMn断电保存全局变量.vi"() -> (w1327:refnum<vi>)
            n866 = call <userlib>:"Write Panel to INI__ogtk.vi"("error in (no error)"=w1325, "VI ref"=w1327, "refnum"=w1328) -> ("error out"=w1324:errorcluster, "refnum out"=w1326:T15)  [unwired: 7 in]
            n867 = call <vilib>:"Close Config Data.vi"("error in (no error)"=w1324, "refnum"=w1326) -> ("error out"=w1319:errorcluster, "file path"=w1318:path)  [unwired: 8 in]
            n868 = Open/Create/Replace File(file path (use dialog)=w1318, error in=w1319) -> (refnum out=w1322:refnum<file>, error out=w1323:errorcluster)  [unwired: 4 in, 1 out]
            n869 = Flush File(refnum=w1322, error in=w1323) -> (refnum out=w1321:refnum<file>, error out=w1320:errorcluster)
            n870 = Close File(refnum=w1321, error in=w1320) -> ()  [unwired: 2 out]
          }
        }
      }
      event "CODMn跨度量程选择": Value Change {
        n871 = event-data() -> ()  [unwired: 1 in, 6 out]
        n872 = flat-sequence {
          frame #0 {
            n873 = global write "CODMn断电保存全局变量.vi" "CODMn跨度量程选择"("CODMn跨度量程选择") -> ()
          }
          frame #1 {
            n874 = global read "COD读取DATA全局.vi" "配置文件ini"() -> (w1332:string)
            n875 = call <vilib>:"Application Directory.vi"() -> ("Application Directory"=w1345:path)
            n876 = Build Path(base path=w1345, name or relative path=w1332) -> (appended path=w1344:path)
            n877 = call <vilib>:"Open Config Data.vi"("configuration file path"=w1344) -> ("error out"=w1340:errorcluster, "refnum"=w1343:T15)  [unwired: 8 in, 1 out]
            n878 = vi-ref "斯坦道CODMn.lvlib:CODMn断电保存全局变量.vi"() -> (w1342:refnum<vi>)
            n879 = call <userlib>:"Write Panel to INI__ogtk.vi"("error in (no error)"=w1340, "VI ref"=w1342, "refnum"=w1343) -> ("error out"=w1339:errorcluster, "refnum out"=w1341:T15)  [unwired: 7 in]
            n880 = call <vilib>:"Close Config Data.vi"("error in (no error)"=w1339, "refnum"=w1341) -> ("error out"=w1334:errorcluster, "file path"=w1333:path)  [unwired: 8 in]
            n881 = Open/Create/Replace File(file path (use dialog)=w1333, error in=w1334) -> (refnum out=w1337:refnum<file>, error out=w1338:errorcluster)  [unwired: 4 in, 1 out]
            n882 = Flush File(refnum=w1337, error in=w1338) -> (refnum out=w1336:refnum<file>, error out=w1335:errorcluster)
            n883 = Close File(refnum=w1336, error in=w1335) -> ()  [unwired: 2 out]
          }
        }
      }
      event "CODMn零点核查选择": Value Change {
        n884 = event-data() -> ()  [unwired: 1 in, 6 out]
        n885 = global write "CODMn断电保存全局变量.vi" "CODMn零点核查选择"("CODMn零点核查选择") -> ()
      }
      event "校准1", "校准2", "校准3", "校准4", "校准5": Value Change {
        n886 = event-data() -> ()  [unwired: 1 in, 6 out]
        n887 = flat-sequence {
          frame #0 {
            n888 = Build Array("校准1", "校准2", "校准3", "校准4", "校准5") -> (w1349:bool[])
            n889 = for {
              tunnel: w1349 -> [w1360] mode=indexing
              i -> [w1353]
              n890 = case shown="4" w1353 {
                tunnel: ["浓度1" "浓度2" "浓度3" "浓度4" "浓度5"] -> w1356
                frame 0, Default {
                }
                frame 1 {
                }
                frame 2 {
                }
                frame 3 {
                }
                frame 4 {
                }
              }
              n891 = Multiply(x=w1356, y=100.0) -> (x*y=w1354:dbl)
              n892 = Insert Into Array(array=u16[] [] ("values"), index=0 ("索引"), new element=w1354) -> (w1357:u16[])
              n893 = case shown="真" w1360 {
                tunnel: w1357 -> [_ w1367]
                tunnel: w1353 -> [_ w1370]
                frame False {
                }
                frame True {
                  n894 = Increment(x=w1370) -> (x+1=→"当前校准":i32)
                  n895 = call "CODMnMB_api.vi"("STEP"=enum16{"open", "read", "write", "close"}."write", "values"=w1367, "starting address"=u16 4274) -> ()  [unwired: 5 in, 4 out]
                }
              }
            }
          }
          frame #1 {
            n896 = local read "当前校准"() -> (w1377:i32)
            n897 = case shown="5" w1377 {
              tunnel: [w1381 w1382 w1383 w1384 w1385] -> w1376
              frame 1, Default {
                n898 = local read "浓度1"() -> (w1381:dbl)
              }
              frame 2 {
                n899 = local read "浓度2"() -> (w1382:dbl)
              }
              frame 3 {
                n900 = local read "浓度3"() -> (w1383:dbl)
              }
              frame 4 {
                n901 = local read "浓度4"() -> (w1384:dbl)
              }
              frame 5 {
                n902 = local read "浓度5"() -> (w1385:dbl)
              }
            }
            n903 = Not Equal To 0?(x=w1376) -> (x != 0?=w1374:bool)
            n904 = case shown="真" w1374 {
              tunnel: [u16 8 ("address") u16 9 ("address")] -> w1380
              tunnel: ["校零" ("测量模式") "校标" ("测量模式")] -> w1375
              frame False {
              }
              frame True {
              }
            }
            n905 = global write "COD测量模式全局.vi" "测量模式"(w1375) -> ()
            n906 = Insert Into Array(array=u16[] [] ("values"), index=0 ("索引"), new element=w1380) -> (w1371:u16[])
            n907 = call "CODMnMB_api.vi"("STEP"=enum16{"open", "read", "write", "close"}."write", "values"=w1371, "starting address"=u16 4608 ("address")) -> ()  [unwired: 5 in, 4 out]
          }
          frame #2 {
            n908 = local read "选用水样"() -> (w1393:enum16{"葡萄糖", "草酸钠"})
            n909 = local read "量程选择"() -> (w1392:enum16{"低量程", "高量程", "0-2量程"})
            n910 = case shown="\"葡萄糖\", 默认" w1393 {
              tunnel: ["葡萄糖标线" ("section") "草酸钠标线" ("section")] -> w1394
              frame "葡萄糖", Default {
              }
              frame "草酸钠" {
              }
            }
            n911 = global read "COD读取DATA全局.vi" "配置文件ini"() -> (w1390:string)
            n912 = case shown="\"0-2量程\"" w1392 {
              tunnel: ["低量程" "高量程" "0-2量程"] -> w1395
              frame "低量程", Default {
              }
              frame "高量程" {
              }
              frame "0-2量程" {
              }
            }
            n913 = call <vilib>:"Application Directory.vi"() -> ("Application Directory"=w1402:path)
            n914 = Concatenate Strings(w1394, w1395) -> (w1391:string)
            n915 = Build Path(base path=w1402, name or relative path=w1390) -> (appended path=w1403:path)
            n916 = local read "当前校准"() -> (w1398:i32)
            n917 = call <vilib>:"Open Config Data.vi"("configuration file path"=w1403) -> ("error out"=w1400:errorcluster, "refnum"=w1401:T15)  [unwired: 8 in, 1 out]
            n918 = call-poly <vilib>:"Write Key.vi"("section"=w1391, "error in (no error)"=w1400, "value"=w1398, "key"="当前选用的校准" ("section"), "refnum"=w1401) -> ("error out"=w1396:errorcluster, "refnum out"=w1397:T15)  [unwired: 4 in, 1 out]
            n919 = call <vilib>:"Close Config Data.vi"("error in (no error)"=w1396, "refnum"=w1397) -> ()  [unwired: 8 in, 2 out]
          }
        }
      }
      event "自动切换量程:", "低切高阈值:", "高切低阈值:": Value Change {
        n920 = event-data() -> ()  [unwired: 1 in, 6 out]
        n921 = flat-sequence {
          frame #0 {
            n922 = local read "自动切换量程:"() -> (w1411:enum16{"关闭", "自动切换测一次", "自动切换测两次"})
            n923 = local read "低切高阈值:"() -> (w1410:dbl)
            n924 = local read "高切低阈值:"() -> (w1409:dbl)
            n925 = global write "CODMn断电保存全局变量.vi" "自动切换量程:"(w1411) -> ()
            n926 = global write "CODMn断电保存全局变量.vi" "低切高阈值:"(w1410) -> ()
            n927 = global write "CODMn断电保存全局变量.vi" "高切低阈值:"(w1409) -> ()
          }
          frame #1 {
            n928 = global read "COD读取DATA全局.vi" "配置文件ini"() -> (w1412:string)
            n929 = call <vilib>:"Application Directory.vi"() -> ("Application Directory"=w1425:path)
            n930 = Build Path(base path=w1425, name or relative path=w1412) -> (appended path=w1424:path)
            n931 = call <vilib>:"Open Config Data.vi"("configuration file path"=w1424) -> ("error out"=w1420:errorcluster, "refnum"=w1423:T15)  [unwired: 8 in, 1 out]
            n932 = vi-ref "斯坦道CODMn.lvlib:CODMn断电保存全局变量.vi"() -> (w1422:refnum<vi>)
            n933 = call <userlib>:"Write Panel to INI__ogtk.vi"("error in (no error)"=w1420, "VI ref"=w1422, "refnum"=w1423) -> ("error out"=w1419:errorcluster, "refnum out"=w1421:T15)  [unwired: 7 in]
            n934 = call <vilib>:"Close Config Data.vi"("error in (no error)"=w1419, "refnum"=w1421) -> ("error out"=w1414:errorcluster, "file path"=w1413:path)  [unwired: 8 in]
            n935 = Open/Create/Replace File(file path (use dialog)=w1413, error in=w1414) -> (refnum out=w1417:refnum<file>, error out=w1418:errorcluster)  [unwired: 4 in, 1 out]
            n936 = Flush File(refnum=w1417, error in=w1418) -> (refnum out=w1416:refnum<file>, error out=w1415:errorcluster)
            n937 = Close File(refnum=w1416, error in=w1415) -> ()  [unwired: 2 out]
          }
        }
      }
      event "模型": Value Change {
        n938 = event-data() -> ()  [unwired: 1 in, 6 out]
        n939 = global read "COD读取DATA全局.vi" "配置文件ini"() -> (w1426:string)
        n940 = call <vilib>:"Application Directory.vi"() -> ("Application Directory"=w1435:path)
        n941 = Build Path(base path=w1435, name or relative path=w1426) -> (appended path=w1434:path)
        n942 = call <vilib>:"Open Config Data.vi"("configuration file path"=w1434) -> ("error out"=w1432:errorcluster, "refnum"=w1433:T15)  [unwired: 8 in, 1 out]
        n943 = local read "模型"() -> (w1427:enum32{"线性", "多项式"})
        n944 = call-poly <vilib>:"Write Key.vi"("section"="CODMn模型选择" ("key"), "error in (no error)"=w1432, "value"=w1427, "key"="线性和多项式", "refnum"=w1433) -> ("error out"=w1428:errorcluster, "refnum out"=w1429:T15)  [unwired: 4 in, 1 out]
        n945 = call <vilib>:"Close Config Data.vi"("error in (no error)"=w1428, "refnum"=w1429) -> ()  [unwired: 8 in, 2 out]
      }
      event "浓度1", "浓度2", "浓度3", "泵滴定数1", "泵滴定数2", "泵滴定数3", "启用1", "启用2", "启用3", "浓度4", "浓度5", "泵滴定数4", "泵滴定数5", "启用4", "启用5": Value Change {
        n946 = event-data() -> ()  [unwired: 1 in, 6 out]
        n947 = global read "COD读取DATA全局.vi" "配置文件ini"() -> (w1436:string)
        n948 = local read "选用水样"() -> (w1452:enum16{"葡萄糖", "草酸钠"})
        n949 = local read "量程选择"() -> (w1451:enum16{"低量程", "高量程", "0-2量程"})
        n950 = case shown="\"0-2量程\"" w1451 {
          tunnel: ["低量程" "高量程" "0-2量程"] -> w1449
          frame "低量程", Default {
          }
          frame "高量程" {
          }
          frame "0-2量程" {
          }
        }
        n951 = call <vilib>:"Application Directory.vi"() -> ("Application Directory"=w1510:path)
        n952 = case shown="\"葡萄糖\", 默认" w1452 {
          tunnel: ["葡萄糖标线" ("section") "草酸钠标线" ("section")] -> w1458
          frame "葡萄糖", Default {
          }
          frame "草酸钠" {
          }
        }
        n953 = Build Path(base path=w1510, name or relative path=w1436) -> (appended path=w1509:path)
        n954 = call <vilib>:"Open Config Data.vi"("configuration file path"=w1509) -> ("error out"=w1507:errorcluster, "refnum"=w1508:T15)  [unwired: 8 in, 1 out]
        n955 = local read "浓度1"() -> (w1505:dbl)
        n956 = Concatenate Strings(w1458, w1449) -> (w1450:string)
        n957 = local read "浓度2"() -> (w1489:dbl)
        n958 = call-poly <vilib>:"Write Key.vi"("section"=w1450, "error in (no error)"=w1507, "value"=w1505, "key"="浓度1", "refnum"=w1508) -> ("error out"=w1504:errorcluster, "refnum out"=w1503:T15)  [unwired: 4 in, 1 out]
        n959 = local read "浓度3"() -> (w1485:dbl)
        n960 = call-poly <vilib>:"Write Key.vi"("section"=w1450, "error in (no error)"=w1504, "value"=w1489, "key"="浓度2", "refnum"=w1503) -> ("error out"=w1502:errorcluster, "refnum out"=w1501:T15)  [unwired: 4 in, 1 out]
        n961 = local read "泵滴定数1"() -> (w1483:dbl)
        n962 = call-poly <vilib>:"Write Key.vi"("section"=w1450, "error in (no error)"=w1502, "value"=w1485, "key"="浓度3", "refnum"=w1501) -> ("error out"=w1500:errorcluster, "refnum out"=w1499:T15)  [unwired: 4 in, 1 out]
        n963 = call-poly <vilib>:"Write Key.vi"("section"=w1450, "error in (no error)"=w1500, "value"=w1483, "key"="泵滴定数1", "refnum"=w1499) -> ("error out"=w1498:errorcluster, "refnum out"=w1497:T15)  [unwired: 4 in, 1 out]
        n964 = local read "泵滴定数2"() -> (w1481:dbl)
        n965 = call-poly <vilib>:"Write Key.vi"("section"=w1450, "error in (no error)"=w1498, "value"=w1481, "key"="泵滴定数2", "refnum"=w1497) -> ("error out"=w1496:errorcluster, "refnum out"=w1495:T15)  [unwired: 4 in, 1 out]
        n966 = local read "泵滴定数3"() -> (w1479:dbl)
        n967 = local read "浓度4"() -> (w1448:dbl)
        n968 = call-poly <vilib>:"Write Key.vi"("section"=w1450, "error in (no error)"=w1496, "value"=w1479, "key"="泵滴定数3", "refnum"=w1495) -> ("error out"=w1494:errorcluster, "refnum out"=w1493:T15)  [unwired: 4 in, 1 out]
        n969 = local read "浓度5"() -> (w1447:dbl)
        n970 = call-poly <vilib>:"Write Key.vi"("section"=w1450, "error in (no error)"=w1494, "value"=w1448, "key"="浓度4", "refnum"=w1493) -> ("error out"=w1487:errorcluster, "refnum out"=w1488:T15)  [unwired: 4 in, 1 out]
        n971 = call-poly <vilib>:"Write Key.vi"("section"=w1450, "error in (no error)"=w1487, "value"=w1447, "key"="浓度5", "refnum"=w1488) -> ("error out"=w1445:errorcluster, "refnum out"=w1446:T15)  [unwired: 4 in, 1 out]
        n972 = local read "泵滴定数4"() -> (w1444:dbl)
        n973 = call-poly <vilib>:"Write Key.vi"("section"=w1450, "error in (no error)"=w1445, "value"=w1444, "key"="泵滴定数4", "refnum"=w1446) -> ("error out"=w1492:errorcluster, "refnum out"=w1491:T15)  [unwired: 4 in, 1 out]
        n974 = local read "泵滴定数5"() -> (w1443:dbl)
        n975 = call-poly <vilib>:"Write Key.vi"("section"=w1450, "error in (no error)"=w1492, "value"=w1443, "key"="泵滴定数5", "refnum"=w1491) -> ("error out"=w1441:errorcluster, "refnum out"=w1442:T15)  [unwired: 4 in, 1 out]
        n976 = local read "启用1"() -> (w1467:bool)
        n977 = call-poly <vilib>:"Write Key.vi"("section"=w1450, "error in (no error)"=w1441, "value"=w1467, "key"="启用1", "refnum"=w1442) -> ("error out"=w1463:errorcluster, "refnum out"=w1466:T15)  [unwired: 4 in, 1 out]
        n978 = local read "启用2"() -> (w1464:bool)
        n979 = call-poly <vilib>:"Write Key.vi"("section"=w1450, "error in (no error)"=w1463, "value"=w1464, "key"="启用2", "refnum"=w1466) -> ("error out"=w1474:errorcluster, "refnum out"=w1473:T15)  [unwired: 4 in, 1 out]
        n980 = local read "启用3"() -> (w1462:bool)
        n981 = call-poly <vilib>:"Write Key.vi"("section"=w1450, "error in (no error)"=w1474, "value"=w1462, "key"="启用3", "refnum"=w1473) -> ("error out"=w1472:errorcluster, "refnum out"=w1471:T15)  [unwired: 4 in, 1 out]
        n982 = local read "启用4"() -> (w1437:bool)
        n983 = call-poly <vilib>:"Write Key.vi"("section"=w1450, "error in (no error)"=w1472, "value"=w1437, "key"="启用4", "refnum"=w1471) -> ("error out"=w1470:errorcluster, "refnum out"=w1469:T15)  [unwired: 4 in, 1 out]
        n984 = local read "启用5"() -> (w1438:bool)
        n985 = call-poly <vilib>:"Write Key.vi"("section"=w1450, "error in (no error)"=w1470, "value"=w1438, "key"="启用5", "refnum"=w1469) -> ("error out"=w1439:errorcluster, "refnum out"=w1440:T15)  [unwired: 4 in, 1 out]
        n986 = local read "选用水样"() -> (w1457:enum16{"葡萄糖", "草酸钠"})
        n987 = call-poly <vilib>:"Write Key.vi"("section"="标线选择", "error in (no error)"=w1439, "value"=w1457, "key"="选用水样", "refnum"=w1440) -> ("error out"=w1454:errorcluster, "refnum out"=w1455:T15)  [unwired: 4 in, 1 out]
        n988 = call <vilib>:"Close Config Data.vi"("error in (no error)"=w1454, "refnum"=w1455) -> ()  [unwired: 8 in, 2 out]
      }
      event "读取": Value Change {
        (unwired) u16 94 ("number of holding registers")
        (unwired) u16 4616 ("starting address")
        n989 = event-data() -> ()  [unwired: 1 in, 6 out]
        n990 = Bundle By Name(cluster=cluster{"命令":string} {"命令"=""} ("元素"), "命令"="CODMn读取公式" ("名称（未命名）")) -> (w1516:cluster{"命令":string})
        n991 = Enqueue Element(queue=w1520, element=w1516, error in (no error)=w1519) -> ()  [unwired: 1 in, 3 out]
      }
      event "写入": Mouse Down {
        n992 = event-data() -> ()  [unwired: 1 in, 8 out]
        n993 = Two Button Dialog(message="确认是否写入公式，写入会覆盖原有公式！" ("消息")) -> (T button?=w1521:bool)  [unwired: 2 in]
        n994 = case shown="真" w1521 {
          frame False {
          }
          frame True {
            n995 = local read "模型"() -> (w1528:enum32{"线性", "多项式"})
            n996 = case shown="\"多项式\"" w1528 {
              tunnel: [w1532 w1575] -> w1526
              tunnel: [w1531 w1574] -> w1525
              frame "线性", Default {
                n997 = local read "测量模式(公式)"() -> (w1533:u16)
                n998 = case shown="1" w1533 {
                  tunnel: [u16 4626 ("starting address") w1540 w1545 w1550 w1555 w1560 w1565 w1570] -> w1532
                  frame 0, Default {
                  }
                  frame 1 {
                    n999 = local read "量程选择"() -> (w1539:enum16{"低量程", "高量程", "0-2量程"})
                    n1000 = case shown="\"低量程\", 默认" w1539 {
                      tunnel: [u16 4626 ("starting address") u16 4632 ("starting address") u16 4638 ("starting address")] -> w1540
                      frame "低量程", Default {
                      }
                      frame "高量程" {
                      }
                      frame "0-2量程" {
                      }
                    }
                  }
                  frame 2 {
                    n1001 = local read "量程选择"() -> (w1544:enum16{"低量程", "高量程", "0-2量程"})
                    n1002 = case shown="\"低量程\", 默认" w1544 {
                      tunnel: [u16 4638 ("starting address") u16 4644 ("starting address") u16 4638 ("starting address")] -> w1545
                      frame "低量程", Default {
                      }
                      frame "高量程" {
                      }
                      frame "0-2量程" {
                      }
                    }
                  }
                  frame 3 {
                    n1003 = local read "量程选择"() -> (w1549:enum16{"低量程", "高量程", "0-2量程"})
                    n1004 = case shown="\"低量程\", 默认" w1549 {
                      tunnel: [u16 4650 ("starting address") u16 4656 ("starting address") u16 4638 ("starting address")] -> w1550
                      frame "低量程", Default {
                      }
                      frame "高量程" {
                      }
                      frame "0-2量程" {
                      }
                    }
                  }
                  frame 4 {
                    n1005 = local read "量程选择"() -> (w1554:enum16{"低量程", "高量程", "0-2量程"})
                    n1006 = case shown="\"低量程\", 默认" w1554 {
                      tunnel: [u16 4662 ("starting address") u16 4668 ("starting address") u16 4638 ("starting address")] -> w1555
                      frame "低量程", Default {
                      }
                      frame "高量程" {
                      }
                      frame "0-2量程" {
                      }
                    }
                  }
                  frame 5 {
                    n1007 = local read "量程选择"() -> (w1559:enum16{"低量程", "高量程", "0-2量程"})
                    n1008 = case shown="\"低量程\", 默认" w1559 {
                      tunnel: [u16 4674 ("starting address") u16 4680 ("starting address") u16 4638 ("starting address")] -> w1560
                      frame "低量程", Default {
                      }
                      frame "高量程" {
                      }
                      frame "0-2量程" {
                      }
                    }
                  }
                  frame 6 {
                    n1009 = local read "量程选择"() -> (w1564:enum16{"低量程", "高量程", "0-2量程"})
                    n1010 = case shown="\"低量程\", 默认" w1564 {
                      tunnel: [u16 4686 ("starting address") u16 4692 ("starting address") u16 4638 ("starting address")] -> w1565
                      frame "低量程", Default {
                      }
                      frame "高量程" {
                      }
                      frame "0-2量程" {
                      }
                    }
                  }
                  frame 7 {
                    n1011 = local read "量程选择"() -> (w1569:enum16{"低量程", "高量程", "0-2量程"})
                    n1012 = case shown="\"低量程\", 默认" w1569 {
                      tunnel: [u16 4698 ("starting address") u16 4704 ("starting address") u16 4638 ("starting address")] -> w1570
                      frame "低量程", Default {
                      }
                      frame "高量程" {
                      }
                      frame "0-2量程" {
                      }
                    }
                  }
                }
                n1013 = local read "K"() -> (w1537:dbl)
                n1014 = local read "b"() -> (w1536:dbl)
                n1015 = Build Array(w1537, w1536, 0.0 ("元素")) -> (w1535:dbl[])
                n1016 = call "浮点转CDAB整形cod.vi"("浮点数"=w1535) -> ("CDAB整形输出"=w1531:u16[])  [unwired: 10 in]
              }
              frame "多项式" {
                # "b,k,c"
                n1017 = local read "测量模式(公式)"() -> (w1576:u16)
                n1018 = case shown="1" w1576 {
                  tunnel: [u16 4626 ("starting address") w1584 w1589 w1594 w1599 w1604 w1609 w1614] -> w1575
                  frame 0, Default {
                  }
                  frame 1 {
                    n1019 = local read "量程选择"() -> (w1583:enum16{"低量程", "高量程", "0-2量程"})
                    n1020 = case shown="\"低量程\", 默认" w1583 {
                      tunnel: [u16 4626 ("starting address") u16 4632 ("starting address") u16 4638 ("starting address")] -> w1584
                      frame "低量程", Default {
                      }
                      frame "高量程" {
                      }
                      frame "0-2量程" {
                      }
                    }
                  }
                  frame 2 {
                    n1021 = local read "量程选择"() -> (w1588:enum16{"低量程", "高量程", "0-2量程"})
                    n1022 = case shown="\"低量程\", 默认" w1588 {
                      tunnel: [u16 4638 ("starting address") u16 4644 ("starting address") u16 4638 ("starting address")] -> w1589
                      frame "低量程", Default {
                      }
                      frame "高量程" {
                      }
                      frame "0-2量程" {
                      }
                    }
                  }
                  frame 3 {
                    n1023 = local read "量程选择"() -> (w1593:enum16{"低量程", "高量程", "0-2量程"})
                    n1024 = case shown="\"低量程\", 默认" w1593 {
                      tunnel: [u16 4650 ("starting address") u16 4656 ("starting address") u16 4638 ("starting address")] -> w1594
                      frame "低量程", Default {
                      }
                      frame "高量程" {
                      }
                      frame "0-2量程" {
                      }
                    }
                  }
                  frame 4 {
                    n1025 = local read "量程选择"() -> (w1598:enum16{"低量程", "高量程", "0-2量程"})
                    n1026 = case shown="\"低量程\", 默认" w1598 {
                      tunnel: [u16 4662 ("starting address") u16 4668 ("starting address") u16 4638 ("starting address")] -> w1599
                      frame "低量程", Default {
                      }
                      frame "高量程" {
                      }
                      frame "0-2量程" {
                      }
                    }
                  }
                  frame 5 {
                    n1027 = local read "量程选择"() -> (w1603:enum16{"低量程", "高量程", "0-2量程"})
                    n1028 = case shown="\"低量程\", 默认" w1603 {
                      tunnel: [u16 4674 ("starting address") u16 4680 ("starting address") u16 4638 ("starting address")] -> w1604
                      frame "低量程", Default {
                      }
                      frame "高量程" {
                      }
                      frame "0-2量程" {
                      }
                    }
                  }
                  frame 6 {
                    n1029 = local read "量程选择"() -> (w1608:enum16{"低量程", "高量程", "0-2量程"})
                    n1030 = case shown="\"低量程\", 默认" w1608 {
                      tunnel: [u16 4686 ("starting address") u16 4692 ("starting address") u16 4638 ("starting address")] -> w1609
                      frame "低量程", Default {
                      }
                      frame "高量程" {
                      }
                      frame "0-2量程" {
                      }
                    }
                  }
                  frame 7 {
                    n1031 = local read "量程选择"() -> (w1613:enum16{"低量程", "高量程", "0-2量程"})
                    n1032 = case shown="\"低量程\", 默认" w1613 {
                      tunnel: [u16 4698 ("starting address") u16 4704 ("starting address") u16 4638 ("starting address")] -> w1614
                      frame "低量程", Default {
                      }
                      frame "高量程" {
                      }
                      frame "0-2量程" {
                      }
                    }
                  }
                }
                n1033 = local read "多项式系数"() -> (w1581:dbl[])
                n1034 = Index Array(array=w1581) -> (element #1=w1578:dbl, element #2=w1579:dbl, element #3=w1577:dbl)  [unwired: 3 in]
                n1035 = Build Array(w1579, w1578, w1577) -> (w1580:dbl[])
                n1036 = call "浮点转CDAB整形cod.vi"("浮点数"=w1580) -> ("CDAB整形输出"=w1574:u16[])  [unwired: 10 in]
              }
            }
            n1037 = call "CODMnMB_api.vi"("STEP"=enum16{"open", "read", "write", "close"}."write", "values"=w1525, "starting address"=w1526) -> ("error out"=w1524:errorcluster)  [unwired: 5 in, 3 out]
            n1038 = case shown="错误" w1524 {
              tunnel: ["写入成功！" "写入失败！"] -> w1523
              frame No Error {
              }
              frame Error {
              }
            }
            n1039 = One Button Dialog(message=w1523) -> ()  [unwired: 1 in, 1 out]
          }
        }
      }
      event "一键写入": Value Change {
        n1040 = event-data() -> ()  [unwired: 1 in, 6 out]
        n1041 = Two Button Dialog(message="确认是否写入公式，写入会覆盖原有公式！" ("消息")) -> (T button?=w1618:bool)  [unwired: 2 in]
        n1042 = case shown="真" w1618 {
          frame False {
          }
          frame True {
            n1043 = local read "模型"() -> (w1622:enum32{"线性", "多项式"})
            n1044 = case shown="\"多项式\"" w1622 {
              tunnel: [w1625 w1676] -> w1620
              frame "线性", Default {
                n1045 = property on="测量模式(公式)" class="Ring (严格)"() -> ("NumItems"=w1626:u32)  [unwired: 2 in, 2 out]
                n1046 = for {
                  N: w1626 -> [_]
                  tunnel: [w1627] -> w1625
                  i -> [w1632]
                  n1047 = Increment(x=w1632) -> (x+1=w1631:i32)
                  n1048 = local read "K"() -> (w1636:dbl)
                  n1049 = case shown="1" w1631 {
                    tunnel: [u16 4626 ("starting address") w1642 w1647 w1652 w1657 w1662 w1667 w1672] -> w1629
                    frame 0, Default {
                    }
                    frame 1 {
                      n1050 = local read "量程选择"() -> (w1641:enum16{"低量程", "高量程", "0-2量程"})
                      n1051 = case shown="\"低量程\", 默认" w1641 {
                        tunnel: [u16 4626 ("starting address") u16 4632 ("starting address") u16 4638 ("starting address")] -> w1642
                        frame "低量程", Default {
                        }
                        frame "高量程" {
                        }
                        frame "0-2量程" {
                        }
                      }
                    }
                    frame 2 {
                      n1052 = local read "量程选择"() -> (w1646:enum16{"低量程", "高量程", "0-2量程"})
                      n1053 = case shown="\"低量程\", 默认" w1646 {
                        tunnel: [u16 4638 ("starting address") u16 4644 ("starting address") u16 4638 ("starting address")] -> w1647
                        frame "低量程", Default {
                        }
                        frame "高量程" {
                        }
                        frame "0-2量程" {
                        }
                      }
                    }
                    frame 3 {
                      n1054 = local read "量程选择"() -> (w1651:enum16{"低量程", "高量程", "0-2量程"})
                      n1055 = case shown="\"低量程\", 默认" w1651 {
                        tunnel: [u16 4650 ("starting address") u16 4656 ("starting address") u16 4638 ("starting address")] -> w1652
                        frame "低量程", Default {
                        }
                        frame "高量程" {
                        }
                        frame "0-2量程" {
                        }
                      }
                    }
                    frame 4 {
                      n1056 = local read "量程选择"() -> (w1656:enum16{"低量程", "高量程", "0-2量程"})
                      n1057 = case shown="\"高量程\"" w1656 {
                        tunnel: [u16 4662 ("starting address") u16 4668 ("starting address") u16 4638 ("starting address")] -> w1657
                        frame "低量程", Default {
                        }
                        frame "高量程" {
                        }
                        frame "0-2量程" {
                        }
                      }
                    }
                    frame 5 {
                      n1058 = local read "量程选择"() -> (w1661:enum16{"低量程", "高量程", "0-2量程"})
                      n1059 = case shown="\"低量程\", 默认" w1661 {
                        tunnel: [u16 4674 ("starting address") u16 4680 ("starting address") u16 4638 ("starting address")] -> w1662
                        frame "低量程", Default {
                        }
                        frame "高量程" {
                        }
                        frame "0-2量程" {
                        }
                      }
                    }
                    frame 6 {
                      n1060 = local read "量程选择"() -> (w1666:enum16{"低量程", "高量程", "0-2量程"})
                      n1061 = case shown="\"低量程\", 默认" w1666 {
                        tunnel: [u16 4686 ("starting address") u16 4692 ("starting address") u16 4638 ("starting address")] -> w1667
                        frame "低量程", Default {
                        }
                        frame "高量程" {
                        }
                        frame "0-2量程" {
                        }
                      }
                    }
                    frame 7 {
                      n1062 = local read "量程选择"() -> (w1671:enum16{"低量程", "高量程", "0-2量程"})
                      n1063 = case shown="\"低量程\", 默认" w1671 {
                        tunnel: [u16 4698 ("starting address") u16 4704 ("starting address") u16 4638 ("starting address")] -> w1672
                        frame "低量程", Default {
                        }
                        frame "高量程" {
                        }
                        frame "0-2量程" {
                        }
                      }
                    }
                  }
                  n1064 = local read "b"() -> (w1637:dbl)
                  n1065 = Build Array(w1636, w1637, 0.0 ("元素")) -> (w1638:dbl[])
                  n1066 = call "浮点转CDAB整形cod.vi"("浮点数"=w1638) -> ("CDAB整形输出"=w1635:u16[])  [unwired: 10 in]
                  n1067 = Insert Into Array(array=u16[] [], index=0 ("索引"), new element=w1635) -> (w1628:u16[])
                  n1068 = call "CODMnMB_api.vi"("STEP"=enum16{"open", "read", "write", "close"}."write", "values"=w1628, "starting address"=w1629) -> ("error out"=w1627:errorcluster)  [unwired: 5 in, 3 out]
                }
              }
              frame "多项式" {
                # "b,k,c"
                n1069 = property on="测量模式(公式)" class="Ring (严格)"() -> ("NumItems"=w1677:u32)  [unwired: 2 in, 2 out]
                n1070 = for {
                  N: w1677 -> [_]
                  tunnel: [w1678] -> w1676
                  i -> [w1683]
                  n1071 = local read "多项式系数"() -> (w1687:dbl[])
                  n1072 = Increment(x=w1683) -> (x+1=w1682:i32)
                  n1073 = case shown="2" w1682 {
                    tunnel: [u16 4626 ("starting address") w1694 w1699 w1704 w1709 w1714 w1719 w1724] -> w1679
                    frame 0, Default {
                    }
                    frame 1 {
                      n1074 = local read "量程选择"() -> (w1693:enum16{"低量程", "高量程", "0-2量程"})
                      n1075 = case shown="\"低量程\", 默认" w1693 {
                        tunnel: [u16 4626 ("starting address") u16 4632 ("starting address") u16 4638 ("starting address")] -> w1694
                        frame "低量程", Default {
                        }
                        frame "高量程" {
                        }
                        frame "0-2量程" {
                        }
                      }
                    }
                    frame 2 {
                      n1076 = local read "量程选择"() -> (w1698:enum16{"低量程", "高量程", "0-2量程"})
                      n1077 = case shown="\"低量程\", 默认" w1698 {
                        tunnel: [u16 4638 ("starting address") u16 4644 ("starting address") u16 4638 ("starting address")] -> w1699
                        frame "低量程", Default {
                        }
                        frame "高量程" {
                        }
                        frame "0-2量程" {
                        }
                      }
                    }
                    frame 3 {
                      n1078 = local read "量程选择"() -> (w1703:enum16{"低量程", "高量程", "0-2量程"})
                      n1079 = case shown="\"低量程\", 默认" w1703 {
                        tunnel: [u16 4650 ("starting address") u16 4656 ("starting address") u16 4638 ("starting address")] -> w1704
                        frame "低量程", Default {
                        }
                        frame "高量程" {
                        }
                        frame "0-2量程" {
                        }
                      }
                    }
                    frame 4 {
                      n1080 = local read "量程选择"() -> (w1708:enum16{"低量程", "高量程", "0-2量程"})
                      n1081 = case shown="\"低量程\", 默认" w1708 {
                        tunnel: [u16 4662 ("starting address") u16 4668 ("starting address") u16 4638 ("starting address")] -> w1709
                        frame "低量程", Default {
                        }
                        frame "高量程" {
                        }
                        frame "0-2量程" {
                        }
                      }
                    }
                    frame 5 {
                      n1082 = local read "量程选择"() -> (w1713:enum16{"低量程", "高量程", "0-2量程"})
                      n1083 = case shown="\"低量程\", 默认" w1713 {
                        tunnel: [u16 4674 ("starting address") u16 4680 ("starting address") u16 4638 ("starting address")] -> w1714
                        frame "低量程", Default {
                        }
                        frame "高量程" {
                        }
                        frame "0-2量程" {
                        }
                      }
                    }
                    frame 6 {
                      n1084 = local read "量程选择"() -> (w1718:enum16{"低量程", "高量程", "0-2量程"})
                      n1085 = case shown="\"低量程\", 默认" w1718 {
                        tunnel: [u16 4686 ("starting address") u16 4692 ("starting address") u16 4638 ("starting address")] -> w1719
                        frame "低量程", Default {
                        }
                        frame "高量程" {
                        }
                        frame "0-2量程" {
                        }
                      }
                    }
                    frame 7 {
                      n1086 = local read "量程选择"() -> (w1723:enum16{"低量程", "高量程", "0-2量程"})
                      n1087 = case shown="\"低量程\", 默认" w1723 {
                        tunnel: [u16 4698 ("starting address") u16 4704 ("starting address") u16 4638 ("starting address")] -> w1724
                        frame "低量程", Default {
                        }
                        frame "高量程" {
                        }
                        frame "0-2量程" {
                        }
                      }
                    }
                  }
                  n1088 = Index Array(array=w1687) -> (element #1=w1690:dbl, element #2=w1689:dbl, element #3=w1691:dbl)  [unwired: 3 in]
                  n1089 = Build Array(w1689, w1690, w1691) -> (w1688:dbl[])
                  n1090 = call "浮点转CDAB整形cod.vi"("浮点数"=w1688) -> ("CDAB整形输出"=w1686:u16[])  [unwired: 10 in]
                  n1091 = Insert Into Array(array=u16[] [], index=0 ("索引"), new element=w1686) -> (w1680:u16[])
                  n1092 = call "CODMnMB_api.vi"("STEP"=enum16{"open", "read", "write", "close"}."write", "values"=w1680, "starting address"=w1679) -> ("error out"=w1678:errorcluster)  [unwired: 5 in, 3 out]
                }
              }
            }
            n1093 = case shown="无错误" w1620 {
              tunnel: ["写入成功！" "写入失败！"] -> w1621
              frame No Error {
              }
              frame Error {
              }
            }
            n1094 = One Button Dialog(message=w1621) -> ()  [unwired: 1 in, 1 out]
          }
        }
      }
      event "滴定曲线": Value Change {
        n1095 = event-data() -> ()  [unwired: 1 in, 6 out]
        n1096 = property on="窗格" class="Pane"("Origin"=T16 {"Horizontal"=0, "Vertical"=3200} ("原点")) -> ()  [unwired: 2 in, 2 out]
      }
      event "历史波形": Value Change {
        n1097 = event-data() -> ()  [unwired: 1 in, 6 out]
        n1098 = call-poly <vilib>:"Read Waveforms from File.vi"() -> ("error out"=w1729:errorcluster, "first waveform in record"=w1730:waveform(dbl))  [unwired: 6 in, 2 out]
        n1099 = case shown="无错误" w1729 {
          tunnel: w1730 -> [w1733 _]
          frame No Error {
            n1100 = Unbundle By Name(w1733) -> ("t0"=→"波形时间":timestamp, "Y"=w1732:dbl[])  [unwired: 2 out]
            n1101 = local write "滴定数-ORP值"(w1732) -> ()
            n1102 = local write "ORP滴定曲线"(w1732) -> ()
          }
          frame Error {
            n1103 = One Button Dialog(message="打开失败" ("消息")) -> ()  [unwired: 1 in, 1 out]
          }
        }
      }
      event "释放串口": Value Change {
        n1104 = event-data() -> ()  [unwired: 1 in, 6 out]
        n1105 = Two Button Dialog(message="确认是否释放串口，释放串口将导致通信失败！" ("消息")) -> (T button?=w1735:bool)  [unwired: 2 in]
        n1106 = case shown="真" w1735 {
          tunnel: w1738 -> [_ w1740]
          tunnel: w1737 -> [_ w1739]
          frame False {
          }
          frame True {
            n1107 = Bundle By Name(cluster=cluster{"命令":string} {"命令"=""} ("元素"), "命令"="停用模块" ("名称（未命名）")) -> (w1741:cluster{"命令":string})
            n1108 = Enqueue Element(queue=w1740, element=w1741, error in (no error)=w1739) -> ()  [unwired: 1 in, 3 out]
          }
        }
      }
      event "打开串口": Value Change {
        n1109 = event-data() -> ()  [unwired: 1 in, 6 out]
        n1110 = global read "CODMn断电保存全局变量.vi" "VISA resource name"() -> (w1752:refnum<visa-resource-name>)
        n1111 = global read "CODMn断电保存全局变量.vi" "PORT"() -> (w1744:string)
        n1112 = global read "CODMn断电保存全局变量.vi" "IP"() -> (w1745:string)
        n1113 = call "串口配置.vi"("PORT"=w1744, "IP"=w1745, "请选择串口:"=w1752) -> ("PORT 2"=w1746:string, "IP 2"=w1747:string, "确认 2"=w1750:bool, "VISA资源名称 2"=w1751:refnum<visa-resource-name>)  [unwired: 5 in]
        n1114 = case shown="真" w1750 {
          tunnel: w1751 -> [_ w1760]
          tunnel: w1749 -> [_ w1756]
          tunnel: w1748 -> [_ w1755]
          tunnel: w1747 -> [_ w1754]
          tunnel: w1746 -> [_ w1753]
          frame False {
          }
          frame True {
            n1115 = global write "CODMn断电保存全局变量.vi" "VISA resource name"(w1760) -> ()
            n1116 = global write "CODMn断电保存全局变量.vi" "PORT"(w1753) -> ()
            n1117 = global write "CODMn断电保存全局变量.vi" "IP"(w1754) -> ()
            n1118 = Bundle By Name(cluster=cluster{"命令":string} {"命令"=""} ("元素"), "命令"="启用模块" ("名称（未命名）")) -> (w1757:cluster{"命令":string})
            n1119 = Enqueue Element(queue=w1756, element=w1757, error in (no error)=w1755) -> ()  [unwired: 1 in, 3 out]
          }
        }
      }
      event Timeout {
        n1120 = event-data() -> ()  [unwired: 1 in, 3 out]
      }
    }
  }
  n1121 = while {
    tunnel: w12 -> [w1770]
    tunnel: w11 -> [w1769]
    tunnel: w3 -> [_]
    stop <- FALSE stop-if-true
    # "主循环界面显示"
    n1122 = flat-sequence {
      frame #0 {
        # "测量状态显示"
        n1123 = global read "COD读取DATA全局.vi" "测量状态"() -> (w1804:u16[])
        n1124 = To Word Integer(number=w1804) -> (16bit integer=w1815:i16[])
        n1125 = Index Array(array=w1815, index #1=0 ("索引"), index #4=3 ("索引"), index #14=13 ("索引"), index #15=14 ("索引"), index #21=20 ("索引"), index #32=31 ("索引")) -> (element #1=w1820:i16, element #2=w1819:i16, element #3=w1818:i16, element #4=→"CODMn工作状态":i16, element #5=→"模式（受控）":i16, element #6=→"进样管":i16, element #7=→"高锰酸钾":i16, element #8=→"草酸钠":i16, element #9=→"硫酸":i16, element #10=w1814:i16, element #11=w1835:i16, element #12=w1810:i16, element #13=→"报警数字":i16, element #14=w1841:i16, element #15=w1826:i16, element #16=→"多列列表框":i16, element #21=w1802:i16, element #33=→"分":i16, element #34=→"秒":i16)  [unwired: 28 in, 15 out]
        n1126 = Number To Decimal String(number=w1802) -> (decimal integer string=→"基本量程(显示)":string)  [unwired: 1 in]
        n1127 = Build Array(w1820, w1819, w1818) -> (w1821:i16[])
        n1128 = To Single Precision Float(number=w1814) -> (single precision float=→"ORP显示":sgl)
        n1129 = call "HexToDate.vi"("数组"=w1821) -> ("DATE"=w1816:timestamp[])  [unwired: 10 in]
        n1130 = Index Array(array=w1816) -> (element=→"仪器时间":timestamp)  [unwired: 1 in]
        n1131 = Divide(x=w1835, y=u16 10) -> (x/y=→"温度":dbl)
        n1132 = Divide(x=w1826, y=u16 1000) -> (x/y=→"标度滴定值":dbl)
        n1133 = Equal?(x=w1810, y=u16 2) -> (x = y?=→"断电排液标记":bool)
        n1134 = Equal?(x=w1810, y=u16 1) -> (x = y?=→"排液标记":bool)
        n1135 = Divide(x=w1841, y=u16 1000) -> (x/y=→"零点滴定值":dbl)
      }
    }
    n1136 = flat-sequence {
      frame #0 {
        # "工作状态显示"
        n1137 = local read "CODMn工作状态"() -> (w1779:T1)
        n1138 = Equal?(x=w1779, y=u16 0) -> (x = y?=→"待机":bool)
        n1139 = Equal?(x=w1779, y=u16 8) -> (x = y?=→"校零标记":bool)
        n1140 = Equal?(x=w1779, y=u16 9) -> (x = y?=→"校标标记":bool)
        n1141 = Equal?(x=w1779, y=u16 1) -> (x = y?=→"水样测量":bool)
        n1142 = Equal?(x=w1779, y=u16 7) -> (x = y?=→"质控样测量":bool)
        n1143 = Equal?(x=w1779, y=u16 10) -> (x = y?=→"加标回收测量":bool)
        n1144 = Equal?(x=w1779, y=u16 2) -> (x = y?=→"标样核查标记":bool)
        n1145 = Equal?(x=w1779, y=u16 6) -> (x = y?=→"平行样测量":bool)
        n1146 = Equal?(x=w1779, y=u16 3) -> (x = y?=→"零点核查标记":bool)
        n1147 = Equal?(x=w1779, y=u16 4) -> (x = y?=→"跨度核查标记":bool)
        n1148 = Equal?(x=w1779, y=u16 5) -> (x = y?=→"空白测试标记":bool)
      }
    }
    n1149 = First Call?() -> (First Call?: T/F=w1768:bool)
    n1150 = case shown="真" w1768 {
      tunnel: w1770 -> [w1869 w1874]
      tunnel: w1769 -> [w1868 w1873]
      tunnel: [w1869 w1872] -> w1766
      tunnel: [w1868 w1871] -> w1765
      frame False {
      }
      frame True {
        n1151 = Bundle By Name(cluster=cluster{"命令":string} {"命令"=""} ("元素"), "命令"="CODMn读取参数" ("名称（未命名）")) -> (w1877:cluster{"命令":string})
        n1152 = Enqueue Element(queue=w1874, element=w1877, timeout in ms (-1)=1000 ("超时毫秒(-1)"), error in (no error)=w1873) -> (queue out=w1872:refnum<queue>, error out=w1871:errorcluster)  [unwired: 1 out]
      }
    }
    n1153 = Wait (ms)(milliseconds to wait=u32 1000 ("等待时间（毫秒）")) -> ()  [unwired: 1 out]
    n1154 = Get Queue Status(queue=w1766, error in (no error)=w1765) -> (queue out=w1762:refnum<queue>, error out=w1761:errorcluster, # elements in queue=w1764:i32)  [unwired: 1 in, 5 out]
    n1155 = Equal To 0?(x=w1764) -> (x = 0?=w1763:bool)
    n1156 = flat-sequence {
      frame #0 {
        # "CODMn读取状态"
        n1157 = global read "COD读取DATA全局.vi" "M输出点"() -> (w1888:bool[])
        n1158 = global read "COD读取DATA全局.vi" "温度"() -> (w1889:bool[])
        n1159 = Index Array(array=w1889) -> (element=→"加热":bool)  [unwired: 1 in]
        n1160 = Index Array(array=w1888) -> (element #1=→"搅拌":bool, element #4=→"进水样":bool, element #5=→"进蒸馏水":bool, element #6=→"进标液":bool, element #7=→"进质控样":bool, element #8=→"进加标回收样":bool, element #9=→"进高锰酸钾":bool, element #10=→"进草酸钠":bool, element #11=→"进硫酸":bool)  [unwired: 11 in, 2 out]
      }
    }
    n1161 = case shown="真" w1763 {
      tunnel: w1762 -> [_ w1774]
      tunnel: w1761 -> [_ w1773]
      frame False {
      }
      frame True {
        n1162 = Bundle By Name(cluster=cluster{"命令":string} {"命令"=""} ("元素"), "命令"="CODMn读取" ("名称（未命名）")) -> (w1776:cluster{"命令":string})
        n1163 = Enqueue Element(queue=w1774, element=w1776, timeout in ms (-1)=1000 ("超时毫秒(-1)"), error in (no error)=w1773) -> ()  [unwired: 3 out]
      }
    }
    n1164 = Get Date/Time In Seconds() -> (seconds since 1Jan1904=→"系统时间":timestamp)
    n1165 = flat-sequence {
      frame #0 {
        # "A，B，K"
        # "CODMn读取状态"
        n1166 = global read "COD读取DATA全局.vi" "ORP、时间"() -> (w1892:u16[])
        n1167 = To Word Integer(number=w1892) -> (16bit integer=w1913:i16[])
        n1168 = Split 1D Array(array=w1913, index=3 ("索引")) -> (first subarray=w1894:i16[], second subarray=w1912:i16[])
        n1169 = Index Array(array=w1894) -> (element #1=w1898:i16, element #2=w1897:i16, element #3=w1896:i16)  [unwired: 3 in]
        n1170 = Index Array(array=w1912) -> (element #1=w1907:i16, element #2=w1911:i16, element #3=w1910:i16, element #4=w1909:i16)  [unwired: 4 in]
        n1171 = Build Array(w1898, w1897, w1896) -> (w1895:i16[])
        n1172 = To Single Precision Float(number=w1910) -> (single precision float=w1901:sgl)
        n1173 = To Single Precision Float(number=w1907) -> (single precision float=w1906:sgl)
        n1174 = To Single Precision Float(number=w1911) -> (single precision float=w1905:sgl)
        n1175 = To Single Precision Float(number=w1909) -> (single precision float=w1900:sgl)
        n1176 = call "HexToDate.vi"("数组"=w1895) -> ("DATE"=w1899:timestamp[])  [unwired: 10 in]
        n1177 = Divide(x=w1906, y=sgl 100.0) -> (x/y=→"COD浓度（mg/L)":sgl)
        n1178 = Index Array(array=w1899) -> (element=w1893:timestamp)  [unwired: 1 in]
        n1179 = Number To Decimal String(number=w1905) -> (decimal integer string=→"ORP-A":string)  [unwired: 1 in]
        n1180 = Number To Decimal String(number=w1901) -> (decimal integer string=→"ORP-B":string)  [unwired: 1 in]
        n1181 = Number To Decimal String(number=w1900) -> (decimal integer string=→"ORP-K":string)  [unwired: 1 in]
        n1182 = Format Date/Time String(seconds (now)=w1893) -> (date/time string=→"数据时间":string)  [unwired: 2 in]
      }
    }
    n1183 = flat-sequence {
      frame #0 {
        # "报警状态显示"
        n1184 = local read "报警数字"() -> (w1844:i16)
        n1185 = Equal?(x=w1844, y=u16 9) -> (x = y?=w1847:bool)
        "进水样超量程" <- w1847
        n1186 = Equal?(x=w1844, y=u16 10) -> (x = y?=w1846:bool)
        "排液故障" <- w1846
        n1187 = Equal?(x=w1844, y=u16 2) -> (x = y?=w1854:bool)
        "温控器故障" <- w1854
        n1188 = Equal?(x=w1844, y=u16 3) -> (x = y?=w1853:bool)
        "加热故障" <- w1853
        n1189 = Equal?(x=w1844, y=u16 4) -> (x = y?=w1852:bool)
        "高锰酸钾报警" <- w1852
        n1190 = Equal?(x=w1844, y=u16 5) -> (x = y?=w1851:bool)
        "草酸钠报警" <- w1851
        n1191 = Equal?(x=w1844, y=u16 6) -> (x = y?=w1850:bool)
        "测量错误" <- w1850
        n1192 = Equal?(x=w1844, y=u16 8) -> (x = y?=w1849:bool)
        "校零错误" <- w1849
        n1193 = Equal?(x=w1844, y=u16 7) -> (x = y?=w1848:bool)
        "校标错误" <- w1848
        n1194 = Equal?(x=w1844, y=u16 1) -> (x = y?=w1855:bool)
        "ORP故障" <- w1855
        n1195 = Compound Arithmetic op=OR ("复合运算")(w1855, w1854, w1853, w1852, w1851, w1850, w1848, w1849, w1847, w1846) -> (→"故障标记":bool)
        n1196 = Bundle By Name(cluster=T3 {"ORP故障"=FALSE, "温控器故障"=FALSE, "加热故障"=FALSE, "高锰酸钾报警"=FALSE, "草酸钠报警"=FALSE, "测量错误"=FALSE, "校零错误"=FALSE, "校标错误"=FALSE, " 进水样超量程"=FALSE, "排液阀故障"=FALSE} ("报警簇"), "ORP故障"=w1855, "温控器故障"=w1854, "加热故障"=w1853, "高锰酸钾报警"=w1852, "草酸钠报警"=w1851, "测量错误"=w1850, "校零错误"=w1849, "校标错误"=w1848, "进水样超量程"=w1847, "排液阀故障"=w1846) -> (→"报警簇":T3)
      }
    }
  }
  n1197 = disable-structure shown="禁用" {
    frame Disabled {
      n1198 = call "单步启动选择对话框.vi"() -> ("启动选择2"=w1918:u16)  [unwired: 10 in, 1 out]
      n1199 = case shown="0" w1918 {
        tunnel: [u16 4610 ("address") u16 4610 ("address") u16 4610 ("address") u16 4610 ("address") u16 4610 ("address") u16 4610 ("address") u16 4610 ("address") u16 4610 ("address") u16 4610 ("address") u16 4610 ("address") u16 4610 ("address") u16 4610 ("address") u16 4610 ("address")] -> w1920
        tunnel: [u16 1 ("address") u16 2 ("address") u16 3 ("address") u16 4 ("address") u16 5 ("address") u16 6 ("address") u16 7 ("address") u16 8 ("address") u16 9 ("holding register value") u16 10 ("holding register value") u16 11 ("holding register value") u16 12 ("address") u16 0 ("address")] -> w1917
        frame 0 {
        }
        frame 1 {
        }
        frame 2 {
        }
        frame 3 {
        }
        frame 4 {
        }
        frame 5 {
        }
        frame 6 {
        }
        frame 7 {
        }
        frame 8 {
        }
        frame 9 {
        }
        frame 10 {
        }
        frame 11 {
        }
        frame 12, Default {
        }
      }
      n1200 = Insert Into Array(array=u16[] [] ("values"), index=0 ("索引"), new element=w1917) -> (w1921:u16[])
      n1201 = call "CODMnMB_api.vi"("STEP"=enum16{"open", "read", "write", "close"}."write", "values"=w1921, "starting address"=w1920) -> ()  [unwired: 5 in, 4 out]
    }
    frame Enabled {
    }
  }
